vi "SOUR_POW_CORR_STAT.vi"(0 "VISA IN":refnum<visa-resource-name>, 5 "error in":errorcluster, 7 "Channel":i32) -> (14 "VISA Out":refnum<visa-resource-name>, 16 "Data":string, 19 "error out":errorcluster)   [LabVIEW 2018, in "PNA-X.lvlib"]
doc: "SOURce:POWer:CORRection[:STATe]? [src] \nReturn \nType \nBoolean (1 = ON, 0 = OFF) \nDefault OFF (0) \nLast modified: \nApril 17, 2007 Removed ch and port arguments for 4 settling and accuracy commands. \n9/12/06 MQ Modified for receiver only SPC \n1849\n\nStatus Register Commands \nThe status registers enable you to query the state of selected events that occur in the analyzer. \nNote: This documentation requires familiarity with the \"Standard Status Data Structure - Register \nModel\" as defined in IEEE Std 488.2-1992. \nClick on a blue keyword to view the command details. \nSee Also \nExample Programs \nLearn about Status Registers \nSynchronizing the PNA and Controller \nSCPI Command Tree \nNote: Any bit not shown in the registers is not used but may be reserved for future use. \n1850\n\nStatus Byte Register \nSummarizes the states of the other registers and monitors the PNA output queue. It also generates \nservice requests. The Enable register is called the Service Request Enable Register. \nCommands Description \n*CLS Clears ALL \"event\" registers and the SCPI Error / Event queue. The corresponding \nENABLE registers are unaffected. \n*STB? Reads the value of the analyzer's status byte. The byte remains after being read. \n*SRE? Reads the current state of the Service Request Enable Register. \n*SRE <num> Sets bits in the Service Request Enable register. The current setting of the SRE \nregister is stored in non-volatile memory. Use *SRE 0 to clear the enable. \n<num> Combined value of the weights for bits to be set. \nBit Weight Description Bit is set to 1 when the following conditions exist: \n2 4 Error / Event \nqueue Summary \n(EAV) \nthe Error / Event queue is not empty. To read the error \nmessage, use SYST:ERR? \n3 8 Questionable \nRegister Summary \nany enabled bit in the questionable event status register is \nset to 1 \n4 16 Message Available the output queue is not empty \n5 32 Standard Event \nRegister Summary \nany enabled bit in the standard event status register is set to \n1 \n6 64 Request Service any of the other bits in the status byte register is set to 1 \n(used to alert the controller of a service request within the \nanalyzer). This bit cannot be disabled. \n7 128 Operation Register \nSummary \nany enabled bit in the standard operation event status \nregister is set to 1 \n1851\n\nSTATus:QUEStionable:<keyword> \nSummarizes conditions that monitor the quality of measurement data. \n<keyword> Example \n:CONDition? STAT:QUES:COND? \n:ENABle \n<bits> \nSTAT:QUES:ENAB 1024 \n[:EVENt]? STAT:QUES? \n:NTRansition \n<bits> \nSTAT:QUES:NTR 1024 \n:PTRansition \n<bits> \nSTAT:QUES:PTR 0 \nBit Weight Description Bit is set to 1 when the following conditions exist: \n9 512 Integrity Reg \nsummary \nany enabled bit in the Integrity event register is set to 1 \n10 1024 Limit Registers \nsummary \nany enabled bit in the Limit event registers is set to 1 \n11 2048 Define Registers \nsummary \nany enabled bit in the Define event registers is set to 1 \nSTATus:QUEStionable:INTegrity <keyword> \nSummarizes conditions in the Measurement Integrity register. \n<keyword> Example \n:CONDition? STAT:QUES:INT:COND? \n:ENABle <bits> STAT:QUES:INT:ENAB 1024 \n[:EVENt]? STAT:QUES:INT? \n:NTRansition <bits> STAT:QUES:INT:NTR 1024 \n:PTRansition <bits> STAT:QUES:INT:PTR 0 \n1852\n\nBit Weight Description Bit is set to 1 when the following conditions exist: \n0 1 Measurement \nSummary \nany bit in the Measurement Integrity event register is set to \n1 \n2 4 Hardware \nSummary \nany bit in the Hardware event register is set to 1 \nSTATus:QUEStionable:INTegrity:HARDware<keyword> \nMonitors the status of hardware failures. \n<keyword> Example \n:CONDition? STAT:QUES:INT:HARD:COND? \n:ENABle <bits> STAT:QUES:INT:HARD:ENAB 1024 \n[:EVENt]? STAT:QUES:INT:HARD? \n:NTRansition <bits> STAT:QUES:INT:HARD:NTR 1024 \n:PTRansition <bits> STAT:QUES:INT:HARD:PTR 0 \nBit Weight Description Bit is set to 1 when the following conditions exist: \n1 2 Phase Unlock the source has lost phaselock, possibly caused by a reference \nchannel open or a hardware failure. \n2 4 Unleveled the source power is unleveled. This could be caused by a \nsource set for more power than it can deliver at the tuned \nfrequency. Or it could be caused by a hardware failure. \n3 8 Not used N/A \n4 16 EE Write Failed an attempted write to the EEPROM has failed, possibly \ncaused by a hardware failure. \n5 32 Not used N/A \n6 64 Ramp Cal Failed the analyzer was unable to calibrate the analog ramp \ngenerator due to a possible hardware failure. \n7 128 Not used N/A \n1853\n\nSTATus:QUEStionable:INTegrity:MEASurement<n> <keyword> \nMonitors the lag between changing a channel setting and when the data is ready to query. \nWhen you change the channel state (start/stop freq, bandwidth, and so forth), then the questionable bit \nfor that channel is set. This indicates that your desired channel state does not yet match the data you \nwould get if querying a data trace. When the next sweep is complete (without aborting in the middle), \nand the data trace matches the channel state that produced it, the bit is cleared for that channel. \n<n> Measurement register number. Choose from 1 to 3 \n<keyword> Example \n:CONDition? STAT:QUES:INT:MEAS1:COND? \n:ENABle <bits> STAT:QUES:INT:MEAS2:ENAB 1024 \n[:EVENt]? STAT:QUES:INT:MEAS3? \n:NTRansition <bits> STAT:QUES:INT:MEAS2:NTR 1024 \n:PTRansition <bits> STAT:QUES:INT:MEAS1:PTR 0 \nMeasurement Register <n> \nBit Weight 1 2 3 Bit is set to 1 when the following conditions exist: \n0 1 1 Summary \nfrom \nMeas \nReg 3 \na setting change on this channel has occurred and the \ndata does not yet reflect that change. \n1 2 2 15 29 a setting change on this channel has occurred and the \ndata does not yet reflect that change. \n2 4 3 16 30 a setting change on this channel has occurred and the \ndata does not yet reflect that change. \n3 8 4 17 31 a setting change on this channel has occurred and the \ndata does not yet reflect that change. \n4 16 5 18 32 a setting change on this channel has occurred and the \ndata does not yet reflect that change. \n5 32 6 19 a setting change on this channel has occurred and the \ndata does not yet reflect that change. \n6 64 7 20 a setting change on this channel has occurred and the \ndata does not yet reflect that change. \n1854\n\n7 128 8 21 a setting change on this channel has occurred and the \ndata does not yet reflect that change. \n8 256 9 22 a setting change on this channel has occurred and the \ndata does not yet reflect that change. \n9 512 10 23 a setting change on this channel has occurred and the \ndata does not yet reflect that change. \n10 1024 11 24 a setting change on this channel has occurred and the \ndata does not yet reflect that change. \n11 2048 12 25 a setting change on this channel has occurred and the \ndata does not yet reflect that change. \n12 4096 13 26 a setting change on this channel has occurred and the \ndata does not yet reflect that change. \n13 8192 14 27 a setting change on this channel has occurred and the \ndata does not yet reflect that change. \n14 16384 Summary \nfrom \nMeas \nReg 2 \n28 a setting change on this channel has occurred and the \ndata does not yet reflect that change. \nSTATus:QUEStionable:LIMit<n> <keyword> \nMonitors and summarizes the status of limit line failures. When a trace fails, the representative bit is \nset to 1. \nBit 0 is used to summarize failures in the registers that follow. For example, Limit Register 3, bit 0, \nsummarizes the failures from registers 4 through 10. \nAll enable bits are set to 1 by default. \nTo find the measurement number, use Calc:Par:Mnum \n<n> Limit register: Choose from 1 to 10. \n<keyword> Example \n:CONDition? STAT:QUES:LIM4:COND? \n:ENABle <bits> STAT:QUES:LIM1:ENAB 1024 \n[:EVENt]? STAT:QUES:LIM3? \n:NTRansition <bits> STAT:QUES:LIM2:NTR 1024 \n:NTRansition? STAT:QUES:LIM1:NTR? \n1855\n\n:PTRansition <bits> STAT:QUES:LIM5:PTR 0 \n:PTRansition? STAT:QUES:LIM1:PTR? \nLimit Register <n> \nBit Weight 1 2 3 4 5 6 7 8 ... 41 Bit is set to 1 when the \nfollowing conditions exist: \n0 1 2-42 3-42 4-42 5-42 6-42 7-42 8-42 9-42 ... 42 Summary Bit - If any bit \nfrom that register fails, it \npropagates to the previous \nregister, bit 0. \nTrace Numbers \n1 2 1 15 29 43 57 71 85 99 ... 575 any point on trace fails the \nlimit test \n2 4 2 16 30 44 58 72 86 100 ... 576 any point on trace fails the \nlimit test \n3 8 3 17 31 45 59 73 87 101 ... 577 any point on trace fails the \nlimit test \n4 16 4 18 32 46 60 74 88 102 ... 578 any point on trace fails the \nlimit test \n5 32 5 19 33 47 61 75 89 103 ... 579 any point on trace fails the \nlimit test \n6 64 6 20 34 48 62 76 90 104 ... 580 any point on trace fails the \nlimit test \n7 128 7 21 35 49 63 77 91 105 ... -- any point on trace fails the \nlimit test \n8 256 8 22 36 50 64 78 92 106 ... -- any point on trace fails the \nlimit test \n9 512 9 23 37 51 65 79 93 107 ... -- any point on trace fails the \nlimit test \n10 1024 10 24 38 52 66 80 94 108 ... -- any point on trace fails the \nlimit test \n11 2048 11 25 39 53 67 81 95 109 ... -- any point on trace fails the \nlimit test \n1856\n\n12 4096 12 26 40 54 68 82 96 110 ... -- any point on trace fails the \nlimit test \n13 8192 13 27 41 55 69 83 97 111 ... -- any point on trace fails the \nlimit test \n14 16384 14 28 42 56 70 84 98 112 ... -- any point on trace fails the \nlimit test \nTo determine Register, Bit number, and Weight for trace numbers between 113 and 574 (not shown in \nthe above table) use the following calculations. \nThe limit status for trace numbers higher than 580 can NOT be tracked. \nThe following example calculates the Register, Bit number, and Bit Weight for trace # 400: \nTo determine Limit Register number, use ((Trace # - 1) / 14) + 1. \nTo determine Limit Bit Number, use the remainder +1 of the above calculation. \n((400-1)/14) + 1 = Register# r+1Bit \n399/14 = 28 r7 \n28+1= Register 29 \n7+1= Bit number 8 \nTo determine Limit Bit Weight: Use above table. For example: Bit 8 = 256 \nSTATus:QUEStionable:DEFine<keyword> \nSummarizes conditions in the Questionable:Define:User<1|2|3> event registers. \n<keyword> Example \n:CONDition? STAT:QUES:DEF:COND? \n:ENABle <bits> STAT:QUES:DEF:ENAB 1024 \n[:EVENt]? STAT:QUES:DEF? \n:NTRansition <bits> STAT:QUES:DEF:NTR 1024 \n:PTRansition <bits> STAT:QUES:DEF:PTR 0 \n1857\n\nBit Weight Description Bit is set to 1 when the following conditions exist: \n1 2 USER1 any bit in the USER1 event register is set to 1 \n2 4 USER2 any bit in the USER2 event register is set to 1 \n3 8 USER3 any bit in the USER3 event register is set to 1 \nSTATus:QUEStionable:DEFine:USER<1|2|3><keyword> \nMonitors conditions that you define and map in any of the three QUES:DEF:USER event registers. \n<keyword> Example \n:ENABle <bits> STAT:QUES:DEF:USER1:ENABle 1024 \n[:EVENt]? STAT:QUES:DEF:USER1? \n:MAP <bit>,<error> STAT:QUES:DEF:USER1:MAP 0,-113 'when error -113 occurs, \nbit 0 in USER1 will set to 1. \nBit Weight Description Bit is set to 1 when the following conditions exist: \n0 1 for user user defined \n1 2 for user user defined \n2 4 for user user defined \n3 8 for user user defined \n4 16 for user user defined \n5 32 for user user defined \n6 64 for user user defined \n7 128 for user user defined \n8 256 for user user defined \n9 512 for user user defined \n10 1024 for user user defined \n11 2048 for user user defined \n12 4096 for user user defined \n13 8192 for user user defined \n14 16384 for user user defined \n1858\n\nStandard Event Status Register \nMonitors \"standard\" events that occur in the analyzer. This register can only be cleared by: \na Clear Command (*CLS). \nreading the Standard Enable Status Register (*ESE?). \na power-on transition. The analyzer clears the register and then records any transitions that occur, including \nsetting the Power On bit (7). \nCommands Description \n*ESE? Reads the settings of the standard event ENABLE register. \n*ESE <bits> Sets bits in the standard event ENABLE register. The current setting is saved in \nnon-volatile memory. \n<bits> The sum of weighted bits in the register. Use *ESE 0 to clear the enable \nregister. \n*ESR? Reads and clears the EVENT settings in the Standard Event Status register. \n*OPC Sets bit 0 when the overlapped command is complete. (see Understanding \nCommand Synchronization / OPC). \n*OPC? Operation complete query - read the Operation Complete bit (0). \nBit Weight Description Bit is set to 1 when the following conditions exist: \n0 1 Operation \nComplete \nthe two following events occur in order: \nthe *OPC command is sent to the analyzer 1. \nthe analyzer completes all pending overlapped commands 2. \n1 NA Request \nControl \nNot Supported - the analyzer application is not configured to \ncontrol GPIB operation \n2 4 Query Error a query error is detected indicating: \n- an attempt to read data from the output queue when no data was \npresent OR \n- data in the output queue was lost, as in an overflow \n4 16 Execution \nError \nan execution error is detected indicating: \n- a <PROGRAM DATA> element was outside the legal range or \ninconsistent with the operation of the analyzer OR \n1859\n\n- the analyzer could not execute a valid command due to some \ninternal condition \n5 32 Command \nError \na command error is detected indicating that the analyzer received \na command that: \ndid not follow proper syntax \nwas misspelled \nwas an optional command it does not implement \n7 128 Power ON Power to the analyzer has been turned OFF and then ON since the \nlast time this register was read. \nSTATus:OPERation<keyword> \nSummarizes conditions in the Averaging and Operation:Define:User<1|2|3> event registers. \n<keyword> Example \n:CONDition? STAT:OPER:COND? \n:ENABle <bits> STAT:OPER:ENAB 1024 \n[:EVENt]? STAT:OPER? \n:NTRansition <bits> STAT:OPER:NTR 1024 \n:PTRansition <bits> STAT:OPER:PTR 0 \nBit Weight Description Bit is set to 1 when the following conditions exist: \n8 256 Averaging \nsummary \neither enabled bit in the Averaging summary event register is set \nto 1 \n9 512 User Defined \nsummary \n10 1024 Device \nsummary \neither enabled bit in the Device summary event register is set to \n1 \n1860\n\nSTATus:OPERation:AVERaging<n> <keyword> \nMonitors and summarizes the status of Averaging on traces 1 to 128. When averaging for a trace is \ncomplete, the representative bit is set to 1. \nBit 0 is used to summarize the status in the registers that follow. For example, Average Register, bit 0, \nsummarizes the status from registers 4 through 10. \nAll enable bits are set to 1 by default. \nTo find the measurement number, use Calc:Par:Mnum. \n<n> Averaging Register. Choose from 1 to 10 \n<keyword> Example \n:CONDition? STAT:OPER:AVER1:COND? \n:ENABle <bits> STAT:OPER:AVER1:ENAB 1024 \n[:EVENt]? STAT:OPER:AVER1? \n:NTRansition <bits> STAT:OPER:AVER1:NTR 1024 \n:PTRansition <bits> STAT:OPER:AVER1:PTR 0 \nAveraging Register <n> \nBit Weight 1 2 3 4 5 6 7 8 ... 42 Bit is set to 1 when the \nfollowing conditions exist: \n0 1 2-42 3-42 4-42 5-42 6-42 7-42 8-42 9-42 ... 42 Summary Bit - If any bit \nfrom that register fails, it \npropagates to the previous \nregister, bit 0. \nTrace Numbers \n1 2 1 15 29 43 57 71 85 99 ... 575 Averaging on this trace is \ncomplete \n2 4 2 16 30 44 58 72 86 100 ... 576 Averaging on this trace is \ncomplete \n3 8 3 17 31 45 59 73 87 101 ... 577 Averaging on this trace is \ncomplete \n4 16 4 18 32 46 60 74 88 102 ... 578 Averaging on this trace is \ncomplete \n1861\n\n5 32 5 19 33 47 61 75 89 103 ... 579 Averaging on this trace is \ncomplete \n6 64 6 20 34 48 62 76 90 104 ... 580 Averaging on this trace is \ncomplete \n7 128 7 21 35 49 63 77 91 105 ... -- Averaging on this trace is \ncomplete \n8 256 8 22 36 50 64 78 92 106 ... -- Averaging on this trace is \ncomplete \n9 512 9 23 37 51 65 79 93 107 ... -- Averaging on this trace is \ncomplete \n10 1024 10 24 38 52 66 80 94 108 ... -- Averaging on this trace is \ncomplete \n11 2048 11 25 39 53 67 81 95 109 ... -- Averaging on this trace is \ncomplete \n12 4096 12 26 40 54 68 82 96 110 ... -- Averaging on this trace is \ncomplete \n13 8192 13 27 41 55 69 83 97 111 ... -- Averaging on this trace is \ncomplete \n14 16384 14 28 42 56 70 84 98 112 ... -- Averaging on this trace is \ncomplete \nTo determine Register, Bit number, and Weight for trace numbers between 113 and 574 (not shown in \nthe above table) use the following calculations. \nThe averaging status for trace numbers higher than 580 can NOT be tracked. \nThe following example calculates the Register, Bit number, and Bit Weight for trace # 400: \nTo determine Register number, use ((Trace # - 1) / 14) + 1. \nTo determine Bit Number, use the remainder +1 of the above calculation. \n((400-1)/14) + 1 = Register# r+1Bit \n399/14 = 28 r7 \n28+1= Register 29 \n7+1= Bit number 8 \n1862\n\nTo determine Bit Weight: Use above table. For example: Bit 8 = 256 \nSTATus:OPERation:DEFine<keyword> \nSummarizes conditions in the OPERation:Define:User<1|2|3> event registers. \n<keyword> Example \n:CONDition? STAT:OPER:DEF:COND? \n:ENABle <bits> STAT:OPER:DEF:ENAB 12 \n[:EVENt]? STAT:OPER:DEF? \n:NTRansition <bits> STAT:OPER:DEF:NTR 12 \n:PTRansition <bits> STAT:OPER:DEF:PTR 0 \nBit Weight Description Bit is set to 1 when the following conditions exist: \n1 2 USER1 any bit in the USER1 event register is set to 1 \n2 4 USER2 any bit in the USER2 event register is set to 1 \n3 8 USER3 any bit in the USER3 event register is set to 1 \nSTATus:OPERation:DEFine:USER<1|2|3><keyword> \nMonitors conditions that you define and map in any of the three OPER:DEF:USER event registers. \n<keyword> Example \n:ENABle <bits> STAT:OPER:DEF:USER1:ENAB 1024 \n[:EVENt]? STAT:OPER:DEF:USER1? \n:MAP <bit>,<error> STAT:OPER:DEF:USER1:MAP 0,-113 'when error -113 occurs, \nbit 0 in USER1 will set to 1. \n1863\n\nBit Weight Description Bit is set to 1 when the following conditions exist: \n0 1 for user user defined \n1 2 for user user defined \n2 4 for user user defined \n3 8 for user user defined \n4 16 for user user defined \n5 32 for user user defined \n6 64 for user user defined \n7 128 for user user defined \n8 256 for user user defined \n9 512 for user user defined \n10 1024 for user user defined \n11 2048 for user user defined \n12 4096 for user user defined \n13 8192 for user user defined \n14 16384 for user user defined \nSTATus:OPERation:DEVice<keyword> \nSummarizes conditions in the OPERation:DEVice event registers. \n<keyword> Example \n:CONDition? STAT:OPER:DEV:COND? \n:ENABle <bits> STAT:OPER:DEV:ENAB 16 \n[:EVENt]? STAT:OPER:DEV? \n:NTRansition <bits> STAT:OPER:DEV:NTR 16 \n:PTRansition <bits> STAT:OPER:DEV:PTR 0 \n1864\n\nBit Weight Description Bit is set to 1 when the following conditions exist: \n0 1 Unused \n1 2 Unused \n2 4 Unused \n3 8 Unused \n4 16 Sweep Completed When sweep is complete \n5 32 Unused \n6 64 Unused \n7 128 Unused \n8 256 Unused \n9 512 Unused \n10 1024 Unused \n11 2048 Unused \n12 4096 Unused \n13 8192 Unused \n14 16384 Unused \nLast modified: \nMay 31, 2007 Fixed typo in STAT:QUES:INT register \n9/19/06 MQ Modified for unlimited windows. \n1865\n\nSystem Commands \n1866\n\n1867\n\nClick on a blue keyword to view the command details. \nSee Also \nExample Programs \nLearn about Preset \nSynchronizing the PNA and Controller \nSCPI Command Tree \nSYSTem:ACTive:CHANnel? \n(Read-only) Returns the number of the active channel or an error message if there is no active \nchannel. The active channel is the channel number that contains the active measurement. \nExamples SYST:PRES \nSYST:ACT:CHAN? \n'Returns 1 \nReturn Type Integer \nDefault Not Applicable \nSYSTem:ACTive:MEASurement? \n(Read-only) Returns the name of the active measurement or an error message if there is no active \nmeasurement. While looking at the PNA display, the active measurement is the trace that has an \nindented Trace Status button and a label in the upper-left corner of the display. Only displayed \nmeasurements can be active. \nExamples SYST:PRES \nSYST:ACT:MEAS? \n'Returns \"CH1_S11_1\" \nReturn Type String \nDefault Not Applicable \nSYSTem:CHANnels:HOLD \n1868\n\n(Write-only) Places all channels in hold mode. To place a single channel in hold mode, use \nSENS:SWE:MODE. \nExamples SYST:CHAN:HOLD \nQuery Syntax Not Applicable \nDefault Not Applicable \nSYSTem:CHANnels:RESume \n(Write-only) Resumes the trigger mode of all channels that was in effect before sending \nSYSTem:CHANnels:HOLD (must be sent before SYST:CHAN:RESume). \nExamples SYST:CHAN:RES \nQuery Syntax Not Applicable \nDefault Not Applicable \nSYSTem:COMMunicate:GPIB:PMETer:ADDRess <num> \n(Read-Write) Specifies the GPIB address of the power meter to be used in a source power calibration. \nWhen performing a source power cal, the PNA will search VISA interfaces that are configured in the \nAgilent IO LIbraries on the PNA. \nParameters \n<num> GPIB address of the power meter. Choose any integer between 0 and 30. \nExamples SYST:COMM:GPIB:PMET:ADDR 13 \nsystem:communicate:gpib:pmeter:address 14 \nQuery Syntax SYSTem:COMMunicate:GPIB:PMETer:ADDRess? \nReturn Type Numeric \nDefault 13 \nSYSTem:COMMunicate:GPIB:RDEVice:CLOSe <ID> \n1869\n\n(Write only) Closes the remote GPIB session. This command should be sent when ending every \nsuccessful OPEN session. \nParameters \n<ID> Session identification number that was returned with the OPEN? command. \nExamples See an example program \nQuery Syntax Not Applicable \nDefault Not Applicable \nSYSTem:COMMunicate:GPIB:RDEVice:OPEN <bus>, <addr>, <timeout> \n(Read-Write) Initiates a GPIB pass-through session. First send this OPEN command, then send the \nOPEN query to read the session ID number. An existing GPIB pass-through session remains open \nafter an instrument preset. \nTo learn more about GPIB pass-through capability, see the example program. \nParameters \n<bus> Bus ID number. You can find the USB-GPIB adapter bus number by looking at \nthe dialog that appears when the USB-GPIB device is connected. Error 1073 \nindicates the bus or address number is incorrect. \n<addr> GPIB Address of the device to be controlled \n<timeout> The amount of time (in milliseconds) to wait for a response from the remote \ndevice after sending a command. A \"timeout\" error is displayed after this time \nhas passed without a response. \nExamples See an example program \nQuery Syntax SYSTem:COMMunicate:GPIB:RDEVice:OPEN? \nReturns the session identification number that is used when communicating \nwith this device. \nReturn Type Numeric \nDefault Not Applicable \nSYSTem:COMMunicate:GPIB:RDEVice:READ? <ID> \n1870\n\n(Read-only) Returns data from the GPIB pass-through device. \nParameters \n<ID> Session identification number that was returned with the OPEN? command. \nExamples See an example program \nReturn Type String \nDefault Not Applicable \nSYSTem:COMMunicate:GPIB:RDEVice:RESet \n(Write-only) Performs the same function as SYST:COMM:GPIB:RDEV:CLOS except that ALL \npass-through sessions are closed. \nExamples SYST:COMM:GPIB:RDEV:RES \nQuery Syntax Not Applicable \nDefault Not Applicable \nSYSTem:COMMunicate:GPIB:RDEVice:WBINary <ID>,<data> \n(Write-only) Sends data to a GPIB pass-through device. This command requires a header that \nspecifies the size of the data to be written. The header (described below) is not passed along to the \ndevice. \nUse this command if too many embedded quotes prevent you from using \nSYST:COMM:GPIB:RDEV:WRIT. \nUse SYST:COMM:GPIB:RDEV:OPEN to open the pass through session. \nParameters \n<ID> Session identification number that was returned with the OPEN? command. \n<data> Data to be sent to the GPIB pass-through device. Use the following syntax: \n#<num digits><byte count><data bytes><NL><END> \n<num_digits> specifies how many digits are contained in <byte_count> \n<byte_count> specifies how many data bytes will follow in <data bytes> \nExamples SYSTem:COMMunicate:GPIB:RDEVice:WBINary 101,#17ABC+XYZ<nl><end> \n# - always sent before data.\n1871\n\n1 - specifies that the byte count is one digit (7). \n7 - specifies the number of data bytes that will follow, not counting \n<NL><END>. \nABC+XYZ - Data block \n<nl><end> - always sent at the end of block data. \nThe following example sends a line feed at the end. \nSYST:COMM:GPIB:RDEV:WBIN 1,#210SYST:PRES<EOL> \nThe <EOL> represents your linefeed character. \nQuery Syntax Not Applicable \nDefault Not Applicable \nSYSTem:COMMunicate:GPIB:RDEVice:WBLock <ID>,<data> \n(Write-only) Same as SYSTem:COMM:GPIB:RDEV:WBIN (above) but the header IS passed along \nto the device. \nUse this command if too many embedded quotes prevent you from using \nSYST:COMM:GPIB:RDEV:WRIT. \nParameters \n<ID> Session identification number that was returned with the OPEN? command. \n<data> Data to be sent to the GPIB pass-through device. See previous command. \nExamples See previous example. \nQuery Syntax Not Applicable \nDefault Not Applicable \nSYSTem:COMMunicate:GPIB:RDEVice:WRITe <ID>,<string> \n1872\n\n(Write-only) Sends ASCII string data to the GPIB pass-through device. \nA line feed is NOT appended to the string data. To send a line feed, see the example in \nSYST:COMM:GPIB:RDEV:WBIN. \nParameters \n<ID> Session identification number that was returned with the OPEN? command. \n<string> Commands to be sent to the GPIB pass-through device. \nExamples See an example program \nQuery Syntax Not Applicable \nDefault Not Applicable \nSYSTem:CONFigure <model>,<address> \n(Write-only) Restarts as an \"N-port\" PNA using the specified multiport test set. \nLearn more about PNA Multiport capability. \nSee other commands to configure multiport test sets. \nParameters \n<model> String - Model of the test set with which to restart. \nUse \"Native\" to restart without a test set. \nTo see a list of supported test sets, use SENS:MULT:CAT? \n<address> Numeric - GPIB Address of the test set. Ignored when model = \"Native\". \nExamples SYST:CONF \"NATIVE\",0 \nsystem:configure \"N44xx\",18 \nQuery Syntax Not Applicable \nDefault Not Applicable \nSYSTem:CORRection:WIZard <char> \n1873\n\n(Write-only) Launches either the Calibration Wizard or the Version 2 Calibration Kit File Manager \ndialog box. \nParameters \n<char> Choose from: \nMAIN - Launches the Calibration Wizard \nCKIT - Launches the Version 2 Calibration Kit File Manager dialog box. \nBoth display on the PNA screen. \nExamples SYST:CORR:WIZ MAIN \nsystem:correction:wizard ckit \nQuery Syntax Not Applicable \nDefault Not Applicable \nSYSTem:ERRor? \n(Read-only) Returns the next error in the error queue. Each time the analyzer detects an error, it places \na message in the error queue. When the SYSTEM:ERROR? query is sent, one message is moved from \nthe error queue to the output queue so it can be read by the controller. Error messages are delivered to \nthe output queue in the order they were received. The error queue is cleared when any of the following \nconditions occur: \nWhen the analyzer is switched ON. \nWhen the *CLS command is sent to the analyzer. \nWhen all of the errors are read. \nIf the error queue overflows, the last error is replaced with a \"Queue Overflow\" error. The \noldest errors remain in the queue and the most recent error is discarded. \nExamples SYST:ERR? \nsystem:error? \nDefault Not Applicable \nSYSTem:ERRor:COUNt? \n1874\n\n(Read-only) Returns the number of errors in the error queue. Use SYST:ERR? to read an error. \nExamples SYST:ERR:COUN? \nsystem:error:count? \nDefault Not Applicable \nSYSTem:ERRor:REPort:SUNLeveled <bool> \n(Read-Write) Specifies whether or not to report Source Unleveled errors to the SCPI system error \nbuffer. \nParameters \n<bool> True (or 1) Report Source Unleveled Errors. Read errors from the system \nerror buffer using SYST:ERR? \nFalse (or 0) Do NOT report Source Unleveled Errors. \nExamples SYST:ERR:REP:SUNL 1 \nsystem:error:report:sunleveled true \nQuery Syntax SYSTem:ERRor:REPort:UNLeveled? \nDefault False \nSYSTem:FPReset \n(Write-only) Performs a standard Preset, then deletes the default trace, measurement, and window. \nThe PNA screen becomes blank. \nExamples SYST:FPR \nsystem:fpreset \nDefault Not applicable \nSYSTem:MACRo:COPY:CHANnel<cnum>[:TO] <num> \n1875\n\n(Write-only) Sets up channel <num> as a copy of channel <cnum>. Learn more about copy channels. \nParameters \n<cnum> Any existing channel number. If unspecified, value is set to 1. \n<num> Number of the channel which is to become a copy of channel <cnum>. \nExamples SYST:MACR:COPY:CHAN1 2 \nsystem:macro:copy:channel2:to 3 \nQuery Syntax Not Applicable \nDefault Not Applicable \nSYSTem:PRESet \n(Write-only) Deletes all traces, measurements, and windows. In addition, resets the analyzer to factory \ndefined default settings and creates a S11 measurement named \"CH1_S11_1\". For a list of default \nsettings, see Preset. \nRegardless of the state of the User Preset Enable checkbox, the SYST:PRESet command will always \npreset the PNA to the factory preset settings, and SYST:UPReset will always perform a User Preset. \nIf the PNA display is disabled with DISP:ENAB OFF then SYST:PRES will NOT enable the display. \nThis command performs the same function as *RST. \nExamples SYST:PRES \nsystem:preset \nDefault Not applicable \nSYSTem:PREFerences:ITEM:OFFSet:RCV <bool> \n1876\n\n(Read-Write) Set and return whether to offset the test port receivers by the amount of receiver \nattenuation. Learn more. \nTo send this command using the PNA front panel, open the GPIB Command Processor Console, then \ntype either of the following examples at the command prompt. Then type the Query Syntax and press \nenter to be sure the PNA took the command. \nThis setting remains until changed again using this command, or until the hard drive is changed or \nreformatted. \nParameters \n<bool> Choose from: \nTrue (1) Offset the test port receivers \nFalse (0) Do NOT offset the test port receivers \nExamples SYST:PREF:ITEM:OFFS:RCV 1 \nsystem:preferences:item:offset:rcv false \nQuery Syntax SYSTem:PREFerences:ITEM:OFFSet:RCV? \nReturn Type Boolean \nDefault PNA-L and E836xB: False (does NOT offset the display). \nPNA-X: True (offsets the display). \nSYSTem:PREFerences:ITEM:OFFSet:SRC <bool> \n(Read-Write) Set and return whether to offset the reference receiver by the amount of source \nattenuation. Learn more. \nTo send this command using the PNA front panel, open the GPIB Command Processor Console, then \ntype either of the following examples at the command prompt. Then type the Query Syntax and press \nenter to be sure the PNA took the command. \nThis setting remains until changed again using this command, or until the hard drive is changed or \nreformatted. \nParameters \n<bool> Choose from: \nTrue (1) Offset the reference receivers. \nFalse (0) Do NOT Offset the reference receivers. \n1877\n\nExamples SYST:PREF:ITEM:OFFS:SRC 1 \nsystem:preferences:item:offset:src false \nQuery Syntax SYSTem:PREFerences:ITEM:OFFSet:SRC? \nReturn Type Boolean \nDefault All models: True (offset the display). \nSYSTem:PREFerences:ITEM:PSRTrace <char> \n(Read-Write) At the end of a power sweep, while waiting to trigger the next sweep, maintain source \npower at either the start power level or at the stop power level. \nTo send this command using the PNA front panel, open the GPIB Command Processor Console, then \ntype either of the following examples at the command prompt. Then type the Query Syntax and press \nenter to be sure the PNA took the command. \nThis setting remains until changed again using this command, or until the hard drive is changed or \nreformatted. \nParameters \n<char> Choose from: \nSTARt - Maintain source power at the start power level. \nSTOP - Maintain source power at the stop power level. \nExamples SYST:PREF:ITEM:PSRT STOP \nsystem:preferences:item:psrtrace start \nQuery Syntax SYSTem:PREFerences:ITEM:PSRTrace? \nReturn Type Character \nDefault STARt \nSYSTem:PREFerences:ITEM:RETRace:POWer <char> \n1878\n\n(Read-Write) For single-band frequency or segment sweeps ONLY, specify whether to turn RF power \nON or OFF during a retrace. Learn more about RF power during sweep retrace. \nTo send this command using the PNA front panel, open the GPIB Command Processor Console, then \ntype either of the following examples at the command prompt. Then type the Query Syntax and press \nenter to be sure the PNA took the command. \nThis setting remains until changed using this command, or until the hard drive is changed or \nreformatted. \nParameters \n<char> Choose from: \nAUTO: Power is left ON during retrace of single-band frequency or segment \nsweeps ONLY. \nOFF: Power is turned OFF during retrace of single-band frequency or segment \nsweeps ONLY. \nExamples SYST:PREF:ITEM:RETR:POW OFF \nsystem:preferences:item:retrace:power auto \nQuery Syntax SYSTem:PREFerences:ITEM:RETRace:POWer? \nReturn Type Character \nDefault AUTO \nSYSTem:SECurity[:LEVel] <char> \n(Read-Write) Sets and returns the display of frequency information on the PNA screen and printouts. \nLearn more about security level. \nParameters \n<char> Choose from: \nNone - ALL frequency information is displayed \nLow - NO frequency information is displayed. Frequency information can be \nredisplayed using the Security Setting dialog box or this command.. \nHigh - NO frequency information is displayed. Frequency information can be \nredisplayed ONLY by performing a Preset or recalling an instrument state with \nNone or Low security settings, or using this command. \n1879\n\nExamples SYST:SEC LOW \nsystem:security:level high \nQuery Syntax SYSTem:SECurity[:LEVel]? \nReturn Type Character \nDefault None \nSYSTem:UPReset \n(Write-only) Performs a User Preset. There must be an active User Preset state file (see Load and \nSave) or an error will be returned. Learn more about User Preset. \nRegardless of the state of the User Preset Enable checkbox, the SYST:PRESet command will always \npreset the PNA to the factory preset settings, and SYST:UPReset will always perform a User Preset. \nExamples SYST:UPReset \nsystem:upreset \nQuery Syntax Not Applicable \nDefault Not Applicable \nSYSTem:UPReset:FPANel[:STATe] <bool> \n(Read-Write) 'Checks' and 'clears' the enable box on the User Preset dialog box. This only affects \nsubsequent Presets from the front panel user interface. \nRegardless of the state of the User Preset Enable checkbox, the SYST:PRESet command will always \npreset the PNA to the factory preset settings, and SYST:UPReset will always perform a User Preset. \nParameters \n<bool> Front Panel User Preset State. Choose from: \n0 User Preset OFF \n1 User Preset ON \nExamples SYST:UPR:FPAN 1 \nsystem:upreset:fpanel:state 0 \nQuery Syntax SYSTem:UPREset:FPANel[:STATe]? \nReturn Type Boolean \nDefault 0 \n1880\n\nSYSTem:UPReset:LOAD <file> \n(Read-Write) Loads an existing instrument state file (.sta or .cst) to be used for User Preset. \nSubsequent execution of SYSTem:UPReset will cause the PNA to assume this instrument state. \nRegardless of the state of the User Preset Enable checkbox, the SYST:PRESet command will always \npreset the PNA to the factory preset settings, and SYST:UPReset will always perform a User Preset. \nLearn more about User Preset. \nParameters \n<file> String - Name of the file to be loaded. The default folder \"C:\\Program \nFiles\\Agilent\\Network Analyzer\\Documents\" is used if unspecified. Change \nthe default folder name using MMEMory:CDIRectory. \nExamples SYST:UPR:LOAD '1MHzto20GHzUserPreset.cst' \nsystem:upreset:load 'C:\\Documents and Settings\\Administrator\\My \nDocuments\\NewUserPreset.cst' \nQuery Syntax Not Applicable \nDefault Not Applicable \nSYSTem:UPReset:SAVE[:STATe] \n(Write-only) Saves the current instrument settings as UserPreset.sta. Subsequent execution of \nSYSTem:UPReset will cause the PNA to assume this instrument state. \nRegardless of the state of the User Preset Enable checkbox, the SYST:PRESet command will always \npreset the PNA to the factory preset settings, and SYST:UPReset will always perform a User Preset. \nLearn more about User Preset. \nExamples SYST:UPR:SAVE \nsystem:upreset:save:state \nQuery Syntax Not Applicable \nDefault Not Applicable \nSYSTem:SHORtcut<n>:ARGuments<string> \n1881\n\n(Read-Write) Reads and writes the arguments for the specified macro. On the Edit Macro Dialog, this \nis called the \"Macro run string parameters\". \nParameters \n<n> Numeric. Number of the macro that is stored in the PNA. \nTo find the number of a macro, either open the Macro Setup dialog and count \nthe line number of the desired macro, or query the titles of all 12 macros for the \ndesired macro title. \n<string> Arguments for the specified macro. \nExamples SYST:SHOR1:ARG \n\"http://na.tm.agilent.com/pna/help/PNAWebHelp/help.htm\" \nQuery Syntax SYSTem:SHORtcut<n>:ARGuments? \nDefault Not Applicable \nSYSTem:SHORtcut<n>:DELete \n(Write-only) Removes the specified macro from the list of macros in the PNA. Does not delete the \nmacro executable file. \nParameters \n<n> Numeric. Number of the macro that is stored in the PNA. \nTo find the number of a macro, either open the Macro Setup dialog and count \nthe line number of the desired macro, or query the titles of all 12 macros for the \ndesired macro title. \nExamples SYST:SHOR1:DEL \nQuery Syntax Not Applicable \nDefault Not Applicable \nSYSTem:SHORtcut<n>:EXECute \n1882\n\n(Write-only) Executes (runs) the specified Macro (shortcut) that is stored in the PNA. \nParameters \n<n> Numeric. Number of the macro that is stored in the PNA. \nTo find the number of a macro, either open the Macro Setup dialog and count \nthe line number of the desired macro, or query the titles of all 12 macros for the \ndesired macro title. \nExamples SYST:SHOR1:EXEC \nQuery Syntax Not Applicable \nDefault Not Applicable \nSYSTem:SHORtcut<n>:PATH <string> \n(Read-Write) Defines a Macro (shortcut) by linking a path and file name to the Macro number. To be \nexecuted, the executable file must be put in the PNA at the location indicated by this command. \nParameters \n<n> Numeric. Number of the macro to be stored in the analyzer. If the index \nnumber already exists, the existing macro is replaced with the new macro. \n<string> Full path, file name, and extension, of the existing macro \"executable\" file. \nTo find the number of a macro, either open the Macro Setup dialog and count \nthe line number of the desired macro, or query the titles of all 12 macros for the \ndesired macro title. \nExamples SYST:SHOR1:PATH \"C:\\Program Files\\Agilent\\Network \nAnalyzer\\Documents\\unguideMultiple.vbs\" \nQuery Syntax SYSTem:SHORtcut<n>:PATH? \nDefault Not Applicable \nSYSTem:SHORtcut<n>:TITLe<string> \n1883\n\n(Read-Write) Reads and writes the name of the specified macro. \nParameters \n<n> Numeric. Number of the macro that is stored in the PNA. \nTo find the number of a macro, either open the Macro Setup dialog and count \nthe line number of the desired macro, or query the titles of all 12 macros for the \ndesired macro title. \n<string> The name to be assigned to the macro. \nExamples SYST:SHOR1:TITL \"Guided 4-Port Cal\" \nQuery Syntax SYSTem:SHORtcut<n>:TITLe? \nDefault Not Applicable \nSYSTem:TOUChscreen[:STATe] <bool> \n(Read-Write) Enables and disables the PNA-X touchscreen. \nThis setting remains until changed again from the front-panel or remotely, or until the hard drive is \nchanged or reformatted. \nParameters \n<bool> Choose from: \nTrue (1) Enables the touchscreen. \nFalse (0) Disables the touchscreen. \nExamples SYST:TOUC 1 \nsystem:touchscreen:state false \nQuery Syntax SYSTem:TOUChscreen[:STATe]? \nReturn Type Boolean \nDefault TRUE when shipped from factory. \nLast modified: \nFebruary 23, 2007 MX Added touchscreen command \nNov. 15, 2006 MX Added Unleveled Error reporting \nOct 31, 2006 Added PSRTrace command \n1884\n\n1885\n\nTrigger Commands \nControls the starts or ends of data acquisition. \nClick on a blue keyword to view the command details. \nSee Also \nExample program Triggering the PNA \nSee other SCPI Triggering commands \nLearn about External / Aux Triggering \nSynchronizing the PNA and Controller \n1886\n\nSCPI Command Tree \nTRIGger:AUX:COUNt? \n(Read-only) Returns the number of AUX trigger input / output connector pairs in the instrument. \nPNA-X = 2 \nE836xB and PNA-L models = 1 \nParameters \nExamples TRIG:CHAN:AUX:COUN? \ntrigger:channel2:aux:count? \nReturn Type Numeric \nDefault Not Applicable \nTRIGger:CHANnel<ch>:AUX<n>:DELay <num> \n(Read-Write) Specifies the delay that should be applied by the PNA after the Aux trigger input is \nreceived and before the acquisition is made. \nParameters \n<ch> Any existing channel number. If unspecified, value is set to 1. \n<n> Rear panel connectors used to send or receive signals. \nPNA-X - choose from 1 (AUX TRIG 1 IN) or 2 (AUX TRIG 2 IN) \nAll other models: choose 1. \nIf unspecified, value is set to 1. \n<num> Delay value in seconds. Choose a value between 0 and 3.0 seconds. \nExamples TRIG:CHAN:AUX:DEL .5 \ntrigger:channel2:aux2:delay 1.5 \nQuery Syntax TRIGger:CHANnel<ch>:AUX<n>:DELay? \nReturn Type Numeric \nDefault 0 \n1887\n\nTRIGger:CHANnel<ch>:AUX<n>:DURation <num> \n(Read-Write) Specifies the width of the output pulse, which is the time that the Aux trigger output \nwill be asserted. \nParameters \n<ch> Any existing channel number. If unspecified, value is set to 1. \n<n> Rear panel connector used to send or receive signals. \nPNA-X - choose from 1 (AUX TRIG 1) or 2 (AUX TRIG 2) \nAll other models: choose 1. (BNC Trig I/O \nIf unspecified, value is set to 1. \n<num> Duration value in seconds. Choose a value between 1us (1E-6) and 1 \nExamples TRIG:CHAN:AUX:DUR .1 \ntrigger:channel2:aux2:duration .01 \nQuery Syntax TRIGger:CHANnel<ch>:AUX<n>:DURation? \nReturn Type Numeric \nDefault 1E-6 \nTRIGger:CHANnel<ch>:AUX<n>[:ENABle] <bool> \n(Read-Write) Turns ON / OFF the trigger output. \nParameters \n<ch> Any existing channel number. If unspecified, value is set to 1. \n<n> Rear panel connector used to send or receive signals. \nPNA-X - choose from 1 (AUX TRIG 1) or 2 (AUX TRIG 2) \nAll other models: choose 1. (BNC Trig I/O \nIf unspecified, value is set to 1. \n<bool> ON (or 1) - turns trigger output ON. \nOFF (or 0) - turns trigger output OFF. \nExamples TRIG:CHAN:AUX 1 \ntrigger:channel2:aux2:enable off \n1888\n\nQuery Syntax TRIGger:CHANnel<ch>:AUX<n>:[ENABle]? \nReturn Type Boolean \nDefault OFF \nTRIGger:CHANnel<ch>:AUX<n>:HANDshake <bool> \n(Read-Write) Turns handshake ON / OFF. \nTo enable handshake, the main trigger enable must also be set using TRIG:CHAN:AUX:ENAB. \nWhen ON, PNA waits indefinitely for the input line to be asserted before continuing with the \nacquisition. When OFF, the PNA acquires data without waiting. \nParameters \n<ch> Any existing channel number. If unspecified, value is set to 1. \n<n> Rear panel connector used to send or receive signals. \nPNA-X - choose from 1 (AUX TRIG 1) or 2 (AUX TRIG 2) \nAll other models: choose 1. (BNC Trig I/O \nIf unspecified, value is set to 1. \n<bool> ON (or 1) - turns handshaking ON. \nOFF (or 0) - turns handshaking OFF. \nExamples TRIG:CHAN:AUX:HAND 1 \ntrigger:channel2:aux2:handshake off \nQuery Syntax TRIGger:CHANnel<ch>:AUX<n>:HANDshake? \nReturn Type Boolean \nDefault OFF \nTRIGger:CHANnel<ch>:AUX<n>:INTerval <char> \n1889\n\n(Read-Write) Specifies how often a trigger output signal is sent. \nParameters \n<ch> Any existing channel number. If unspecified, value is set to 1. \n<n> Rear panel connector used to send or receive signals. \nPNA-X - choose from 1 (AUX TRIG 1) or 2 (AUX TRIG 2) \nAll other models: choose 1. (BNC Trig I/O \nIf unspecified, value is set to 1. \n<char> Choose from: \nPOINt Trigger signal is sent every data point. (effectively the same as Point \nsweep) \nSWEep Trigger signal is sent once every sweep. \nExamples TRIG:CHAN:AUX:INT POI \ntrigger:channel2:aux2:interval sweep \nQuery Syntax TRIGger:CHANnel<ch>:AUX<n>:INTerval? \nReturn Type Character \nDefault SWEep \nTRIGger:CHANnel<ch>:AUX<n>:IPOLarity <char> \n(Read-Write) Specifies the polarity of the trigger IN signal to which the PNA will respond. \nParameters \n<ch> Any existing channel number. If unspecified, value is set to 1. \n<n> Rear panel connector used to send or receive signals. \nPNA-X - choose from 1 (AUX TRIG 1) or 2 (AUX TRIG 2) \nAll other models: choose 1. (BNC Trig I/O \nIf unspecified, value is set to 1. \n<char> Choose from: \nPOSitive PNA responds to leading edge or HIGH level \n1890\n\nNEGative PNA responds to trailing edge or LOW level. \nSet Edge or Level triggering using TRIG:CHAN:AUX:TYPE \nExamples TRIG:CHAN:AUX:IPOL POS \ntrigger:channel2:aux2:ipolarity negative \nQuery Syntax TRIGger:CHANnel<ch>:AUX<n>:IPOLarity? \nReturn Type Character \nDefault NEGative \nTRIGger:CHANnel<ch>:AUX<n>:OPOLarity <char> \n(Read-Write) Specifies the polarity of the Aux Output signal being supplied by the PNA. \nParameters \n<ch> Any existing channel number. If unspecified, value is set to 1. \n<n> Rear panel connector used to send or receive signals. \nPNA-X - choose from 1 (AUX TRIG 1) or 2 (AUX TRIG 2) \nAll other models: choose 1. (BNC Trig I/O \nIf unspecified, value is set to 1. \n<char> Choose from: \nPOSitive PNA sends positive going pulse. \nNEGative PNA sends negative going pulse. \nExamples TRIG:CHAN:AUX:OPOL NEG \ntrigger:channel2:aux2:opolarity positive \nQuery Syntax TRIGger:CHANnel<ch>:AUX<n>:OPOLarity? \nReturn Type Character \nDefault NEGative \nTRIGger:CHANnel<ch>:AUX<n>:POSition <char> \n1891\n\n(Read-Write) Specifies whether the aux trigger out signal is sent BEFore or AFTer the acquisition. \nParameters \n<ch> Any existing channel number. If unspecified, value is set to 1. \n<n> Rear panel connector used to send or receive signals. \nPNA-X - choose from 1 (AUX TRIG 1) or 2 (AUX TRIG 2) \nAll other models: choose 1. (BNC Trig I/O \nIf unspecified, value is set to 1. \n<char> Choose from: \nBEFore Use if the external device needs to be triggered before the data is \nacquired, such as a power meter. \nAFTer Use if the external device needs to be triggered just after data has been \nacquired, such as an external source. This could be more efficient since it allows \nthe external device to get ready for the next acquisition at the same time as the \nPNA. \nExamples TRIG:CHAN:AUX:POS BEF \ntrigger:channel2:aux2:position after \nQuery Syntax TRIGger:CHANnel<ch>:AUX<n>:POSition? \nReturn Type Character \nDefault AFTer \nTRIGger:CHANnel<ch>:AUX<n>:TYPE <char>\n1892\n\n(Read-Write) Specifies the type of Aux input detection that the PNA will employ. \nParameters \n<ch> Any existing channel number. If unspecified, value is set to 1. \n<n> Rear panel connector used to send or receive signals. \nPNA-X - choose from 1 (AUX TRIG 1) or 2 (AUX TRIG 2) \nAll other models: choose 1. (BNC Trig I/O \nIf unspecified, value is set to 1. \n<char> Choose from: \nEDGE PNA responds to the leading edge of a signal \nLEVel PNA responds to the level (HIGH or LOW) of a signal \nExamples TRIG:CHAN:AUX:TYPE EDGE \ntrigger:channel2:aux2:type level \nQuery Syntax TRIGger:CHANnel<ch>:AUX<n>:TYPE? \nReturn Type Character \nDefault EDGE \nTRIGger:DELay <num> \n(Read-Write) Sets and reads the trigger delay. This delay is only applied while in External Trigger \nmode. After an external trigger is applied, the start of the sweep is held off for an amount of time \nequal to the delay setting plus any inherent latency. \nParameters \n<num> Delay value in seconds. Choose from 0 to 107. \nExamples TRIG:DEL .0003 \nSets the trigger delay to 300 microseconds. The sweep will not \nstart until approximately 300 microseconds after an external \ntrigger is applied. \nQuery Syntax TRIGger:DELay? \nReturn Type Numeric \nDefault 0 \n1893\n\nTRIGger:CHANnel<ch>:ROUTe:INPut <char> \n(Read-Write) Specifies the connector to use for the external trigger input.(Similar to \nCONTROL:SIGNal <conn>) \nParameters \n<ch> Any existing channel number. If unspecified, value is set to 1. \n<char> Choose from: \nMAIN - meas trig ready \nMATH - material handler \nAUXT - auxio (PNA-L and E836xB ONLY) \nExamples TRIG:CHAN:ROUT:INP MAIN \ntrigger:channel2:route:input main \nQuery Syntax TRIGger:CHANnel<ch>:ROUTe:INPut? \nReturn Type Character \nDefault \nTRIGger:CHANnel<ch>:ROUTe:READy <char> \n(Read-Write) Specifies the connector to use for the external trigger OUT ready line. \nParameters \n<ch> Any existing channel number. If unspecified, value is set to 1. \n<char> Choose from: \nMAIN - Meas trig ready \nMATH - Material handler pin 21 \nAUXT - AUX I/O pin 18 (PNA-L and E836xB ONLY) \nExamples TRIG:CHAN:ROUT:READ main \ntrigger:channel2:route:ready auxt \nQuery Syntax TRIGger:CHANnel<ch>:ROUTe:READy? \nReturn Type Character \nDefault \n1894\n\nTRIGger:PREFerence:AIGLobal <bool> \n(Read-Write) Sets the External Trigger OUT behavior to either Global or Channel. Learn more. \nThis command will cause the PNA to Preset. \nThis setting remains until changed again using this command, or until the hard drive is changed or \nreformatted. \nTo send this command using the PNA front panel, open the GPIB Command Processor Console, then \ntype either of the following examples at the command prompt. Then type the Query Syntax and press \nenter to be sure the PNA took the command. \nParameters \n<bool> Choose from: \nON (or 1) - External I/O Trig properties apply to ALL channels (Global) \nOFF (or 0) - External I/O Trig properties apply to each channel independently. \nExamples TRIG:PREF:AIGL 1 \ntrigger:preference:aiglobal 0 \nQuery Syntax TRIGger:PREFerence:AIGLobal? \nReturn Type Boolean \nDefault 1 - E836xB and PNA-L models \n0 - PNA-X models \nTRIGger[:SEQuence]:LEVel <char> - Superseded \n1895\n\nThis command is replaced with CONTrol:SIGNal \n(Read-Write) Triggers either on a High or Low level trigger signal. This setting only has an effect \nwhen TRIG:SOURce EXTernal is selected. \nParameters \n<char> Choose from: \nHIGH - analyzer triggers on TTL High \nLOW - analyzer triggers on TTL Low \nExamples TRIG:LEV HIGH \ntrigger:sequence:level low \nQuery Syntax TRIGger[:SEQuence]:LEVel? \nReturn Type Character \nDefault LOW \nTRIGger[:SEQuence]:SCOPe <char> \n(Read-Write) Specifies whether a trigger signal is sent to all channels or only the current channel. \nSee Triggering the PNA using SCPI. \nParameters \n<char> Choose from: \nALL - trigger signal is sent to all channels. Also sets SENS:SWEep:TRIG:POINt \nOFF on ALL channels. \nCURRent - trigger signal is sent to only one channel at a time. With each trigger \nsignal, the channel is incremented to the next triggerable channel. \nExamples TRIG:SCOP ALL \ntrigger:sequence:scope current \nQuery Syntax TRIGger[:SEQuence]:SCOPe? \nReturn Type Character \nDefault ALL \nTRIGger[:SEQuence]:SOURce <char> \n1896\n\n(Read-Write) Sets the source of the sweep trigger signal. This command is a super-set of \nINITiate:CONTinuous, which can NOT set the source to External. To configure external triggering, \nsee CONTrol:SIGNal. \nSee Triggering the PNA using SCPI. \nParameters \n<char> Choose from: \nEXTernal - external (rear panel) source. \nIMMediate - internal source sends continuous trigger signals \nMANual - sends one trigger signal when manually triggered from the front panel or \nINIT:IMM is sent. \nExamples TRIG:SOUR EXT \ntrigger:sequence:source immediate \nQuery Syntax TRIGger[:SEQuence]:SOURce? \nReturn Type Character \nDefault IMMediate \nTRIGger:TYPE <char> \n(Read-Write) Specifies the type of EXTERNAL trigger input detection used to listen for signals on \nthe Ext I/O Trig and Meas Trig IN connectors. Edge triggers are most commonly used. \nParameters \n<ch> Any existing channel number. If unspecified, value is set to 1. \n<char> Choose from: \nEDGE PNA responds to the rising and falling edge of a signal \nLEVel PNA responds to a level (HIGH or LOW). \nExamples TRIG:TYPE EDGE \ntrigger:type level \nQuery Syntax TRIGger:TYPE? \nReturn Type Character \nDefault EDGE \n1897\n\nLast modified: \nApril 24, 2007 Clarified trigger source and scope \nFeb 15, 2007 MX Updated for AUX triggering \n1898\n\nCatalog Measurements using SCPI \nThis Visual Basic Program does the following: \nCatalogs the currently defined measurements, windows, and traces \nSelects a measurement for further definition \nAdds a Title to the window \nTo run this program, you need: \nAn established GPIB interface connection \nSee Other SCPI Example Programs \nDim Meas as String \nDim Win as String \nDim Trace as String \n'Read the current measurements in Channel 1 \nGPIB.Write \"CALCulate1:PARameter:CATalog?\" \nMeas = GPIB.Read \nMsgBox (\"Ch1 Measurments: \" & Meas) \n'Read the current windows \nGPIB.Write \"DISPlay:CATalog?\" \nWin = GPIB.Read \nMsgBox (\"Windows: \" & Win) \n'Read current traces in window 1 \nGPIB.Write \"DISPlay:WINDow1:CATalog?\" \nTrace = GPIB.Read \nMsgBox (\"Traces in Window1: \" & Win) \n1899\n\nCreate an FOM Measurement \nThis example program does the following: \ncreates several Frequency Offset measurements in separate windows \ngenerates markers \ncalculates statistics \nsets limit lines and queries results \nqueries a measurement to determine if we have a balanced parameter and what type it is. \nThe SCPI commands in this example are sent over a COM interface using the SCPIStringParser object. You do \nNOT need a GPIB connection to run this example. \nThis VBScript (*.vbs) program can be run as a macro in the PNA. To do this, copy the following code into a text \neditor file such as Notepad and save it on the PNA hard drive as Balanced.vbs. Learn how to setup and run the \nmacro. \nSee Other SCPI Example Programs \nDim app \nDim scpi \nDim Rcount \nDim Rname \n' Create / Get the PNA application. \nSet app = CreateObject(\"AgilentPNA835x.Application\") \nSet scpi = app.ScpiStringParser \n' A comment \nscpi.Execute(\"SYST:FPRESET\") \n'Create an Uncoupled S21 measurement on Chan 1 \n'Query available ranges \nRcount= scpi.Execute(\"SENS:FOM:COUN?\" \nMsgBox(Rcount) \nFor i=1 to Rcount \nRname(i)=sens:fom:rang:name? \nMsgBox(Rname(i)) \nNext \nSENS:FOM:RANG2:COUPLED OFF \n1900\n\nSENS:FOM:RANG2:FREQ:START 1Ghz \nSENS:FOM:RANG2:FREQ:STOP 2Ghz \nSENS:FOM:RANG3:COUPLED OFF \nSENS:FOM:RANG3:FREQ:START 2Ghz \nSENS:FOM:RANG3:FREQ:STOP 3Ghz \nQuestions \nIs cnum necessary on Sens FOM Count? or CAT? Name?\n1901\n\nCreate a Measurement using SCPI \nThis VBScript program creates a new S21 measurement and displays it on the PNA screen. \nThe SCPI commands in this example are sent over a COM interface using the SCPIStringParser object. You do \nNOT need a GPIB connection to run this example. \nThis VBScript (*.vbs) program can be run as a macro in the PNA. To do this, copy the following code into a text \neditor file such as Notepad and save it on the PNA hard drive as NewMeas.vbs. Learn how to setup and run the \nmacro. \nSee Other SCPI Example Programs \nDim app \nDim scpi \n' Create / Get the PNA application. \nSet app = CreateObject(\"AgilentPNA835x.Application\") \nSet scpi = app.ScpiStringParser \n' A comment \n'Preset the analyzer \nscpi.Execute (\"SYST:FPReset\") \n' Create and turn on window 1 \nscpi.Execute (\"DISPlay:WINDow1:STATE ON\") \n'Define a measurement name, parameter \nscpi.Execute (\"CALCulate:PARameter:DEFine 'MyMeas',S21\") \n'Associate (\"FEED\") the measurement name ('MyMeas') to WINDow (1), and give the new \nTRACe a number (1). \nscpi.Execute (\"DISPlay:WINDow1:TRACe1:FEED 'MyMeas'\") \n1902\n\nCreate a Balanced Measurement using SCPI \nThis example program does the following: \ncreates several Balanced measurements in separate windows \ngenerates markers \ncalculates statistics \nsets limit lines and queries results \nqueries a measurement to determine if we have a balanced parameter and what type it is. \nNote: By their nature, balanced measurements are extremely sensitive to phase differences between the two RF \npaths that make up the balanced port, especially at higher frequencies. A good calibration (not performed in this \nexample) is critical to achieving good balanced measurement results. \nThe SCPI commands in this example are sent over a COM interface using the SCPIStringParser object. You do \nNOT need a GPIB connection to run this example. \nThis VBScript (*.vbs) program can be run as a macro in the PNA. To do this, copy the following code into a text \neditor file such as Notepad and save it on the PNA hard drive as Balanced.vbs. Learn how to setup and run the \nmacro. \nSee Other SCPI Example Programs \nDim app \nDim scpi \n' Create / Get the PNA application. \nSet app = CreateObject(\"AgilentPNA835x.Application\") \nSet scpi = app.ScpiStringParser \n' A comment \nscpi.Execute(\"SYST:FPRESET\") \n' Put in \"Single\" trigger mode. \nscpi.Execute(\"SENS:SWE:GROups:COUNt 1\") \nscpi.Execute(\"SENS:SWE:MODE GROUPS\") \n' This example uses DUT topology Bal-Bal - \n' a DUT with a balanced input and balanced output. \n'\n' Port mapping for our DUT: \n' logical port 1 = physical ports 1 and 4 \n' logical port 2 = physical ports 2 and 3 \n' The default is: \n' logical port 1 = physical ports 1 and 2 \n' logical port 2 = physical ports 3 and 4 \n'\n' logical 1 logical 2 \n' ___________ \n' 1 ------| |------ 2 + \n' | DUT | \n' 4 ------|___________|------ 3 - \n1903\n\nscpi.Execute(\"CALC:FSIM:BAL:DEVice BBALanced\") \nscpi.Execute(\"CALC:FSIM:BAL:TOPology:BBAL:PPORts 1,4,2,3\") \n' Set up stimulus \nscpi.Execute(\"SENS:SWE:POINts 801\") \nscpi.Execute(\"SENS:FREQ:STARt 10e6\") \nscpi.Execute(\"SENS:FREQ:STOP 1e9\") \n' Turn on Four windows \nscpi.Execute(\"DISP:WIND1:STATe ON\") \nscpi.Execute(\"DISP:WIND2:STATe ON\") \nscpi.Execute(\"DISP:WIND3:STATe ON\") \nscpi.Execute(\"DISP:WIND4:STATe ON\") \n' Create a trace called \"sdd21\", and for that trace turn on the balanced \n' transformation and set the balanced transformation to BBAL SDD21. \nscpi.Execute(\"CALC:PAR:DEF \"\"sdd21\"\",S11\") \nscpi.Execute(\"CALC:PAR:SEL \"\"sdd21\"\"\") \nscpi.Execute(\"CALC:FSIM:BAL:PAR:STATe ON\") \nscpi.Execute(\"CALC:FSIM:BAL:PAR:BBAL:DEF SDD21\") \n' Feed the sdd21 trace to window 1, trace 1 \nscpi.Execute(\"DISP:WIND1:TRAC1:FEED \"\"sdd21\"\"\") \n' Similarly create 3 more balanced transmission/conversion parameters \n' Create Scd21 \nscpi.Execute(\"CALC:PAR:DEF \"\"scd21\"\",S11\") \nscpi.Execute(\"CALC:PAR:SEL \"\"scd21\"\"\") \nscpi.Execute(\"CALC:FSIM:BAL:PAR:STATe ON\") \nscpi.Execute(\"CALC:FSIM:BAL:PAR:BBAL:DEF SCD21\") \nscpi.Execute(\"DISP:WIND1:TRAC2:FEED \"\"scd21\"\"\") \n' Create Sdc21 \nscpi.Execute(\"CALC:PAR:DEF \"\"sdc21\"\",S11\") \nscpi.Execute(\"CALC:PAR:SEL \"\"sdc21\"\"\") \nscpi.Execute(\"CALC:FSIM:BAL:PAR:STATe ON\") \nscpi.Execute(\"CALC:FSIM:BAL:PAR:BBAL:DEF SDC21\") \nscpi.Execute(\"DISP:WIND1:TRAC3:FEED \"\"sdc21\"\"\") \n' Create Scc21 \nscpi.Execute(\"CALC:PAR:DEF \"\"scc21\"\",S11\") \nscpi.Execute(\"CALC:PAR:SEL \"\"scc21\"\"\") \nscpi.Execute(\"CALC:FSIM:BAL:PAR:STATe ON\") \nscpi.Execute(\"CALC:FSIM:BAL:PAR:BBAL:DEF SCC21\") \nscpi.Execute(\"DISP:WIND1:TRAC4:FEED \"\"scc21\"\"\") \n' Now create logical port 1 reflection parameters, and place them in window 2 \nscpi.Execute(\"CALC:PAR:DEF \"\"sdd11\"\",S11\") \nscpi.Execute(\"CALC:PAR:SEL \"\"sdd11\"\"\") \nscpi.Execute(\"CALC:FSIM:BAL:PAR:STATe ON\") \nscpi.Execute(\"CALC:FSIM:BAL:PAR:BBAL:DEF SDD11\") \n' Feed the sdd11 trace to window 2, trace 1 \nscpi.Execute(\"DISP:WIND2:TRAC1:FEED \"\"sdd11\"\"\") \n' Similarly create 3 more balanced reflection/conversion parameters \nscpi.Execute(\"CALC:PAR:DEF \"\"scd11\"\",S11\") \nscpi.Execute(\"CALC:PAR:SEL \"\"scd11\"\"\") \nscpi.Execute(\"CALC:FSIM:BAL:PAR:STATe ON\") \nscpi.Execute(\"CALC:FSIM:BAL:PAR:BBAL:DEF SCD11\") \nscpi.Execute(\"DISP:WIND2:TRAC2:FEED \"\"scd11\"\"\") \nscpi.Execute(\"CALC:PAR:DEF \"\"sdc11\"\",S11\") \n1904\n\nscpi.Execute(\"CALC:PAR:SEL \"\"sdc11\"\"\") \nscpi.Execute(\"CALC:FSIM:BAL:PAR:STATe ON\") \nscpi.Execute(\"CALC:FSIM:BAL:PAR:BBAL:DEF SDC11\") \nscpi.Execute(\"DISP:WIND2:TRAC3:FEED \"\"sdc11\"\"\") \nscpi.Execute(\"CALC:PAR:DEF \"\"scc11\"\",S11\") \nscpi.Execute(\"CALC:PAR:SEL \"\"scc11\"\"\") \nscpi.Execute(\"CALC:FSIM:BAL:PAR:STATe ON\") \nscpi.Execute(\"CALC:FSIM:BAL:PAR:BBAL:DEF SCC11\") \nscpi.Execute(\"DISP:WIND2:TRAC4:FEED \"\"scc11\"\"\") \n' Now create reverse transmission parameters, and place them in window 3 \nscpi.Execute(\"CALC:PAR:DEF \"\"sdd12\"\",S11\") \nscpi.Execute(\"CALC:PAR:SEL \"\"sdd12\"\"\") \nscpi.Execute(\"CALC:FSIM:BAL:PAR:STATe ON\") \nscpi.Execute(\"CALC:FSIM:BAL:PAR:BBAL:DEF SDD12\") \n' Feed the sdd11 trace to window 3, trace 1 \nscpi.Execute(\"DISP:WIND3:TRAC1:FEED \"\"sdd12\"\"\") \n' Similarly create 3 more balanced reverse transmission/conversion parameters \nscpi.Execute(\"CALC:PAR:DEF \"\"scd12\"\",S11\") \nscpi.Execute(\"CALC:PAR:SEL \"\"scd12\"\"\") \nscpi.Execute(\"CALC:FSIM:BAL:PAR:STATe ON\") \nscpi.Execute(\"CALC:FSIM:BAL:PAR:BBAL:DEF SCD12\") \nscpi.Execute(\"DISP:WIND3:TRAC2:FEED \"\"scd12\"\"\") \nscpi.Execute(\"CALC:PAR:DEF \"\"sdc12\"\",S11\") \nscpi.Execute(\"CALC:PAR:SEL \"\"sdc12\"\"\") \nscpi.Execute(\"CALC:FSIM:BAL:PAR:STATe ON\") \nscpi.Execute(\"CALC:FSIM:BAL:PAR:BBAL:DEF SDC12\") \nscpi.Execute(\"DISP:WIND3:TRAC3:FEED \"\"sdc12\"\"\") \nscpi.Execute(\"CALC:PAR:DEF \"\"scc12\"\",S11\") \nscpi.Execute(\"CALC:PAR:SEL \"\"scc12\"\"\") \nscpi.Execute(\"CALC:FSIM:BAL:PAR:STATe ON\") \nscpi.Execute(\"CALC:FSIM:BAL:PAR:BBAL:DEF SCC12\") \nscpi.Execute(\"DISP:WIND3:TRAC4:FEED \"\"scc12\"\"\") \n' Now create reverse reflection parameters, and place them in window 4 \nscpi.Execute(\"CALC:PAR:DEF \"\"sdd22\"\",S11\") \nscpi.Execute(\"CALC:PAR:SEL \"\"sdd22\"\"\") \nscpi.Execute(\"CALC:FSIM:BAL:PAR:STATe ON\") \nscpi.Execute(\"CALC:FSIM:BAL:PAR:BBAL:DEF SDD22\") \n' Feed the sdd11 trace to window 3, trace 1 \nscpi.Execute(\"DISP:WIND4:TRAC1:FEED \"\"sdd22\"\"\") \n' Similarly create 3 more balanced reverse reflection parameters \nscpi.Execute(\"CALC:PAR:DEF \"\"scd22\"\",S11\") \nscpi.Execute(\"CALC:PAR:SEL \"\"scd22\"\"\") \nscpi.Execute(\"CALC:FSIM:BAL:PAR:STATe ON\") \nscpi.Execute(\"CALC:FSIM:BAL:PAR:BBAL:DEF SCD22\") \nscpi.Execute(\"DISP:WIND4:TRAC2:FEED \"\"scd22\"\"\") \nscpi.Execute(\"CALC:PAR:DEF \"\"sdc22\"\",S11\") \nscpi.Execute(\"CALC:PAR:SEL \"\"sdc22\"\"\") \nscpi.Execute(\"CALC:FSIM:BAL:PAR:STATe ON\") \nscpi.Execute(\"CALC:FSIM:BAL:PAR:BBAL:DEF SDC22\") \nscpi.Execute(\"DISP:WIND4:TRAC3:FEED \"\"sdc22\"\"\") \nscpi.Execute(\"CALC:PAR:DEF \"\"scc22\"\",S11\") \nscpi.Execute(\"CALC:PAR:SEL \"\"scc22\"\"\") \n1905\n\nscpi.Execute(\"CALC:FSIM:BAL:PAR:STATe ON\") \nscpi.Execute(\"CALC:FSIM:BAL:PAR:BBAL:DEF SCC22\") \nscpi.Execute(\"DISP:WIND4:TRAC4:FEED \"\"scc22\"\"\") \n' Show statistics for forward differential transmission \nscpi.Execute(\"CALC:PAR:SEL \"\"sdd21\"\"\") \nscpi.Execute(\"CALC:FUNC:STATistics:STATe ON\") \n' Set up test range for markers. Set up range 1 to be between 100MHz and 900MHz \nscpi.Execute(\"CALC:FUNC:DOMain:USER:STARt 1,100e6\") \nscpi.Execute(\"CALC:FUNC:DOMain:USER:STOP 1,900e6\") \n' Set up a marker on Sdd21, find minimum differential transmission \n' Set this marker to use user-range 1 (previously defined) \nscpi.Execute(\"CALC:PAR:SEL \"\"sdd21\"\"\") \nscpi.Execute(\"CALC:MARK ON\") \nscpi.Execute(\"CALC:MARK:FUNC:DOM:USER:RANGE 1\") \nscpi.Execute(\"CALC:MARK:FUNC:EXEC MIN\") \n' Find Maximum common mode to differential mode conversion within user-range 1. \nscpi.Execute(\"CALC:PAR:SEL \"\"sdc21\"\"\") \nscpi.Execute(\"CALC:MARK ON\") \nscpi.Execute(\"CALC:MARK:FUNC:DOM:USER:RANGE 1\") \nscpi.Execute(\"CALC:MARK:FUNC:EXEC MAX\") \n' Set up limit lines \n' 'MIN' Limit on Sdd21 between 100MHz and 900MHz at -2dB \nscpi.Execute(\"CALC:PAR:SEL \"\"sdd21\"\"\") \nscpi.Execute(\"CALC:LIM:SEGM:TYPE LMIN\") \nscpi.Execute(\"CALC:LIM:SEGM:STIM:STARt 100e6\") \nscpi.Execute(\"CALC:LIM:SEGM:STIM:STOP 900e6\") \nscpi.Execute(\"CALC:LIM:SEGM:AMPL:STARt -2\") \nscpi.Execute(\"CALC:LIM:SEGM:AMPL:STOP -2\") \nscpi.Execute(\"CALC:LIM:DISP:STATe ON\") \nscpi.Execute(\"CALC:LIM:STATe ON\") \n' 'MAX' Limit on Sdc21 between 100MHz and 900MHz at -20dB \nscpi.Execute(\"CALC:PAR:SEL \"\"sdc21\"\"\") \nscpi.Execute(\"CALC:LIM:SEGM:TYPE LMAX\") \nscpi.Execute(\"CALC:LIM:SEGM:STIM:STARt 100e6\") \nscpi.Execute(\"CALC:LIM:SEGM:STIM:STOP 900e6\") \nscpi.Execute(\"CALC:LIM:SEGM:AMPL:STARt -20\") \nscpi.Execute(\"CALC:LIM:SEGM:AMPL:STOP -20\") \nscpi.Execute(\"CALC:LIM:DISP:STATe ON\") \nscpi.Execute(\"CALC:LIM:STATe ON\") \n' \"Single\" trigger to take data. \nscpi.Execute(\"SENS:SWE:MODE GROUPS\") \nresponse = scpi.Execute(\"*OPC?\") \n' Read the limit status byte to determine pass/fail. \n' If bit 1 is set (+2), then our first measurement failed (Sdd21). \n' If bit 3 is set (+8), then our third measurement failed (Sdc21). \n' Both measurements failing would return +10. \nresponse = scpi.Execute(\"STAT:QUES:LIM1:COND?\") \nIf response <> 0 Then \nWscript.Echo \"Failure of limit lines: \" & response \nEnd If \n' Here we demonstrate how to determine if we have \n1906\n\n' a balanced parameter and what type it is. \n' Read back one parameter to verify its type \nscpi.Execute(\"CALC:PAR:SEL \"\"sdd21\"\"\") \n' Is this a balanced parameter? \nisbal = scpi.Execute(\"CALC:FSIM:BAL:PAR?\") \n' Which topology/device is set? \ndevice = scpi.Execute(\"CALC:FSIM:BAL:DEV?\") \ndevice = Left( device, Len(device)-1 ) ' strip off newline \n' Which parameter are we measuring within that topology? \nbalparam = scpi.Execute(\"CALC:FSIM:BAL:PAR:\" & device & \":DEF?\") \nbalparam = Left( balparam, Len(balparam)-1 ) ' strip off newline \nIf isbal Then \nWScript.Echo \"Balanced Parameter: \" & balparam & \" in topology: \" & device & \".\" \nElse \nWScript.Echo \"Parameter not balanced.\" \nEnd If \n1907\n\nChannels, Windows, and Measurements using SCPI \nSOURce and most SENSe commands act on the channel that is specified in the command. Channel 1 is default if \nnot specified. \nMost DISPlay commands act on the window and trace specified in the command. Window1 and Trace1 are \ndefault if not specified. \nCALCulate commands act on the selected measurement in the specified channel. Select the measurement for \neach channel using CALCulate<channel number>:PARameter:SELect <meas name>. You can select one \nmeasurement in each channel. \nThe following Visual Basic program does the following: \nPresets the analyzer \nCreate 2 windows \nCreate 2 Measurements \nFeed the measurements to windows / traces \nChange frequency ranges for channels \nSelect both measurements \nTurn marker 1 ON for each measurement \nTo run this program, you need: \nAn established GPIB interface connection \nSee Other SCPI Example Programs \nGPIB.Write \"SYSTem:PRESet\" \n'Create Measurements \nGPIB.Write \"CALCulate1:PARameter:DEFine 'Meas1',S11\" \nGPIB.Write \"CALCulate2:PARameter:DEFine 'Meas2',S21\" \n' Turn on windows - creates if new \nGPIB.Write \"DISPlay:WINDow1:STATE ON\" \nGPIB.Write \"DISPlay:WINDow2:STATE ON\" \n'Associate (\"FEED\") the measurement name('Meas1') to WINDow(1), and give the new \nTRACe a number(1). \nGPIB.Write \"DISPlay:WINDow1:TRACe1:FEED 'Meas1'\" \nGPIB.Write \"DISPlay:WINDow2:TRACe2:FEED 'Meas2'\" \n'Change each channel's frequency range \nGPIB.Write \"SENSe1:FREQuency:SPAN 1e9\" \nGPIB.Write \"SENSe2:FREQuency:SPAN 2e9\" \n1908\n\n'Select both measurements \nGPIB.Write \"CALCulate1:PARameter:SELect 'Meas1'\" \nGPIB.Write \"CALCulate2:PARameter:SELect 'Meas2'\" \n'Turn marker 1 ON for each measurement \nGPIB.Write \"CALCulate1:MARKer:STATe ON\" \nGPIB.Write \"CALCulate2:MARKer:STATE ON\" \n1909\n\nSetup Sweep Parameters using SCPI \nThis Visual Basic program sets up sweep parameters on the Channel 1 measurement. \nTo run this program, you need: \nAn established GPIB interface connection \nSee Other SCPI Example Programs \nGPIB.Write \"SYSTem:PRESet\" \n'Select the measurement \nGPIB.Write \"CALCulate:PARameter:SELect 'CH1_S11_1'\" \n'Set sweep type to linear \nGPIB.Write \"SENSe1:SWEep:TYPE LIN\" \n'Set IF Bandwidth to 700 Hz \nGPIB.Write \"SENSe1:BANDwidth 700\" \n'Set Center and Span Freq's to 4 GHz \nGPIB.Write \"SENSe1:FREQuency:CENTer 4ghz\" \nGPIB.Write \"SENSe1:FREQuency:SPAN 4ghz\" \n'Set number of points to 801 \nGPIB.Write \"SENSe1:SWEep:POINts 801\" \n'Set sweep generation mode to Analog \nGPIB.Write \"SENSe1:SWEep:GENeration ANAL\" \n'Set sweep time to Automatic \nGPIB.Write \"SENSe1:SWEep:TIME:AUTO ON\" \n'Query the sweep time \nGPIB.Write \"SENSe1:SWEep:TIME? \nSweepTime = GPIB.Read \n1910\n\nSetup the Display using SCPI \nThis Visual Basic program: \nSets data formatting \nTurns ON the Trace, Title, and Frequency Annotation \nAutoscales the Trace \nQueries Per Division, Reference Level, and Reference Position \nTurn ON and set averaging \nTurn ON and set smoothing \nTo run this program, you need: \nAn established GPIB interface connection \nSee Other SCPI Example Programs \nGPIB.Write \"SYSTem:PRESet\" \n'Select the measurement \nGPIB.Write \"CALCulate:PARameter:SELect 'CH1_S11_1'\" \n'Set the Data Format to Log Mag \nGPIB.Write \":CALCulate1:FORMat MLOG\" \n'Turn ON the Trace, Title, and Frequency Annotation \nGPIB.Write \"Display:WINDow1:TRACe1:STATe ON\" \nGPIB.Write \"DISPlay:WINDow1:TITLe:STATe ON\" \nGPIB.Write \"DISPlay:ANNotation:FREQuency ON\" \n'Autoscale the Trace \nGPIB.Write \"Display:WINDow1:TRACe1:Y:Scale:AUTO\" \n'Query back the Per Division, Reference Level, and Reference Position \nGPIB.Write \"DISPlay:WINDow1:TRACe1:Y:SCALe:PDIVision?\" \nPdiv = GPIB.Read \nGPIB.Write \"DISPlay:WINDow1:TRACe1:Y:SCALe:RLEVel?\" \nRlev = GPIB.Read \nGPIB.Write \"DISPlay:WINDow1:TRACe1:Y:SCALe:RPOSition?\" \nPpos = GPIB.Read \n'Turn ON, and average five sweeps \nGPIB.Write \"SENSe1:AVERage:STATe ON\" \nGPIB.Write \"SENSe1:AVERage:Count 5\" \n'Turn ON, and set 20% smoothing aperture \nGPIB.Write \"CALCulate1:SMOothing:STATe ON\" \n1911\n\nGPIB.Write \"CALCulate1:SMOothing:APERture 20\" \n1912\n\nTriggering the PNA using SCPI \nTo understand how to trigger the PNA using SCPI, it is very important to understand the PNA trigger model. Here is \na very simple explanation. These three separate functions control PNA triggering: \nTrigger:Source - Where the trigger signals originate: \nInternal Continuous \nInternal Manual (Single) \nExternal - a trigger source that is connected to the PNA rear panel. \n1. \nTrigger:Scope - what gets triggered: \nGlobal - each signal triggers all channels in turn. \nChannel - each signal triggers ONE channel. \n2. \nChannel settings (Sense<ch>:Sweep:Mode) How many triggers will each channel accept before going into \nhold. \nHOLD - channel will not trigger \nCONTinuous - channel triggers indefinitely \nGROups - channel accepts the number of triggers specified with the last SENS:SWE:GRO:COUN \n<num>. \nPoint trigger SENS1:SWE:TRIG:POINt \n3. \nWhen controlling the PNA using SCPI, a SINGLE trigger is used to ensure that a complete sweep is taken. This \nexample demonstrates how to Single trigger the PNA using two methods. \nSimplest Triggering This method sets the Trigger Source to Internal Continuous - a stream of trigger \nsignals. Each channel is configured to ACCEPT only a single trigger signal, then HOLD. This method can \nalso be used when an External trigger source sends a continuous stream of trigger signals. \nAdvanced Triggering This method SENDS a single trigger from the Source, either Internal (using INIT:IMM) \nor External triggering. Each channel is configured to accept an unlimited number of triggers. This method is \nthe only way to perform point triggering. See INIT:IMM Advanced for details when requiring multiple channels \nto accept continuous and single triggers. \nThe SCPI commands in this example are sent over a COM interface using the SCPIStringParser object. You do \nNOT need a GPIB connection to run this example. \nThis VBScript (*.vbs) program can be run as a macro in the PNA. To do this, copy the following code into a text \neditor file such as Notepad and save it on the PNA hard drive as Trigger.vbs. Learn how to setup and run the \nmacro. \n1913\n\nMeasurement setup example: sets up S11 traces on two channels, 10 points, sweep time of 2 seconds, which \nallows us to verify that the trace is being triggered. \nDim app \nDim scpi \n' Create / Get the PNA application. \nSet app = CreateObject(\"AgilentPNA835x.Application\") \nSet scpi = app.ScpiStringParser \n'============================================ \n'Setup the PNA \n'Preset the analyzer \nscpi.Execute (\"SYST:FPReset\") \n' Create and turn on window/channel 1 \nscpi.Execute (\"DISPlay:WINDow1:STATE ON\") \n'Define a measurement name, parameter \nscpi.Execute (\"CALCulate1:PARameter:DEFine 'MyMeas1',S11\") \n'Associate (\"FEED\") the measurement name ('MyMeas') to WINDow (1) \nscpi.Execute (\"DISPlay:WINDow1:TRACe1:FEED 'MyMeas1'\") \n' Create and turn on window/channel 2 \nscpi.Execute (\"DISPlay:WINDow2:STATE ON\") \n'Define a measurement name, parameter \nscpi.Execute (\"CALCulate2:PARameter:DEFine 'MyMeas2',S11\") \n'Associate (\"FEED\") the measurement name ('MyMeas') to WINDow (2) \nscpi.Execute (\"DISPlay:WINDow2:TRACe2:FEED 'MyMeas2'\") \n'Set slow sweep so we can see \nscpi.Execute (\"SENS1:SWE:TIME 2\") \nscpi.Execute (\"SENS2:SWE:TIME 2\") \n'set few number of points \nscpi.Execute (\"SENS1:SWE:POIN 10\") \nscpi.Execute (\"SENS2:SWE:POIN 10\") \n'============================================ \n' Put both channels in Hold \nscpi.Execute (\"SENS1:SWE:MODE HOLD\") \nscpi.Execute (\"SENS2:SWE:MODE HOLD\") \n'================================ \n'Pick Single Send or Single Accept \nresp=Msgbox (\"Single Send? - Click No for Single Accept\", 4, \"PNA Trigger Demo\") \n1914\n\nIf resp=6 Then \nSingleSend() \nElse \nSingleAccept() \nEnd If \nSimple Triggering The following example sends a continuous stream of trigger signals and each PNA channels is \nset to ACCEPT only a signal trigger signal, then HOLD using the Groups:Count = 1 setting. \nThis example can be used to configure External triggering where the trigger source sends a continuous \nstream of trigger signals. Configure the type of trigger signal that the PNA responds to using the \nCONTrol:SIGNal command. The command in this example sets the PNA to respond to HIGH TTL signals at \nthe rear-panel BNC1 trigger IN connector. This command also automatically sets Trigger Source to External \nTrigger. \nThe TRIG SCOPE (Global or Channel) setting is NOT practical with a continuous stream of trigger signals. \nThe example program directly controls when each channel is triggered. \nAlso, Point triggering can NOT be used with a continuous stream of trigger signals because, with Group \nCount = 1, the channel will accept as many triggers as necessary to complete ONE full sweep. Therefore, \nALL data points in the channel will be continuously triggered. Use the single SEND example for point \ntriggering. \nSub SingleAccept() \n'PNA sends continuous trigger signals \nscpi.Execute (\"TRIG:SOUR IMMediate\") \n'Uncomment the following to set External triggering \n'scpi.Execute (\"CONT:SIGN BNC1,TILHIGH\") \n'IMPORTANT: First send the Count number =1, \n'This command does not make the channel sweep \nscpi.Execute (\"SENS1:SWE:GRO:COUN 1\") \nscpi.Execute (\"SENS2:SWE:GRO:COUN 1\") \nAcceptOne() \nEnd Sub \nSub AcceptOne() \n'The following command makes the channel immediately sweep \n'*OPC? allows the measurement to complete before the controller sends another \ncommand \nscpi.Execute (\"SENS1:SWE:MODE GROUPS;*OPC?\") \n1915\n\n' You could do something to ch2 here before sweeping it \nscpi.Execute (\"SENS2:SWE:MODE GROUPS;*OPC?\") \nresp=Msgbox (\"Another trigger?\", 1, \"PNA Trigger Demo\") \nIf resp=1 Then \nAcceptOne() \nEnd If \nEnd Sub \nAdvanced Trigger This example section performs Single Send triggering. Here, single triggering is accomplished \nby SENDING one trigger signal from the Trigger source and each channel is setup to accept unlimited trigger \nsignals. See the INIT:IMM command for more details. \nUsing this method, it is possible to change Trigger:Scope to Global or Channel. Set trigger scope to channel \nif there is some code to execute between channel measurements. Similarly, this method can be used to set \nPoint triggering. Use this method if there is some code to execute between data point measurements. \nIn addition, this method can also be used to perform External triggering if the external trigger source is \ncapable of SENDING single triggers. See the CONTrol:SIGNal command to set the type of signal to which \nthe PNA will respond. \nIf the external source can only send a continuous stream of trigger signals, then the Single Accept section \nmust be used. \nSub SingleSend() \n'Set Source Internal - Manual Triggering \nscpi.Execute (\"TRIG:SOUR MANual\") \n'If using an External trigger source that is capable of \n'sending SINGLE trigger signals, then uncomment the following. \n'This command automatically sets trigger source to External \n'scpi.Execute (\"CONT:SIGN BNC1,TILHIGH\") \n'Setup Trigger Scope \n'WHAT gets triggered \n'Pick one using comments \n'Set Channel triggering \n'scpi.Execute (\"TRIG:SCOPe CURRent\") \n'Set Global triggering (Default) \nscpi.Execute (\"TRIG:SCOPe ALL\") \n'Set Channel Settings \n1916\n\n'The channels respond to UNLIMITED trigger signals (Default) \nscpi.Execute (\"SENS1:SWE:MODE CONTinuous\") \nscpi.Execute (\"SENS2:SWE:MODE CONTinuous\") \n'To do Point trigger on one or more channels, uncomment the following \n'Point trigger automatically sets Trig:Scope to Current/Channel \n'scpi.Execute (\"SENS1:SWE:TRIG:POINt ON\") \n'scpi.Execute (\"SENS2:SWE:TRIG:POINt ON\") \nIntTrig() \nEnd Sub \nSub IntTrig() \n'If External triggering, replace this Sub with code \n'to single trigger the External Trig Source \nDim resp \n'*OPC? allows the measurement to complete before the controller sends another \ncommand \nscpi.Execute (\"INITiate:IMMediate;*OPC?\") \nresp=Msgbox (\"Another trigger?\", 1, \"PNA Trigger Demo\") \nIf resp=1 Then \nIntTrig() \nEnd If \nEnd Sub \nLast modified: \nApril 24, 2007 Updated with links \nOct. 5, 2006 New topic \n1917\n\nGPIB using Visual C++ \nSee Other SCPI Example Programs \n/* \n* This example assumes the user's PC has a National Instruments GPIB board. The \nexample is comprised of three basic parts: \n* \n* 1. Initialization \n* 2. Main Body \n* 3. Cleanup \n* \n* The Initialization portion consists of getting a handle to the PNA and then doing \na GPIB clear of the PNA. \n* \n* The Main Body consists of the PNA SCPI example. \n* \n* The last step, Cleanup, releases the PNA for front panel control. \n*/ \n#include <stdio.h> \n#include <stdlib.h> \n/* \n* Include the WINDOWS.H and DECL-32.H files. The standard Windows \n* header file, WINDOWS.H, contains definitions used by DECL-32.H and \n* DECL-32.H contains prototypes for the NI GPIB routines and constants. \n*/ \n#include <windows.h> \n#include \"decl-32.h\" \n#define ERRMSGSIZE 1024 // Maximum size of SCPI command string \n#define ARRAYSIZE 1024 // Size of read buffer \n#define BDINDEX 0 // Board Index of GPIB board \n#define PRIMARY_ADDR_OF_PNA 16 // GPIB address of PNA \n#define NO_SECONDARY_ADDR 0 // PNA has no Secondary address \n#define TIMEOUT T10s // Timeout value = 10 seconds \n#define EOTMODE 1 // Enable the END message \n#define EOSMODE 0 // Disable the EOS mode \nint pna; \nchar ValueStr[ARRAYSIZE + 1]; \nchar ErrorMnemonic[21][5] = {\"EDVR\", \"ECIC\", \"ENOL\", \"EADR\", \"EARG\", \n\"ESAC\", \"EABO\", \"ENEB\", \"EDMA\", \"\", \n\"EOIP\", \"ECAP\", \"EFSO\", \"\", \"EBUS\", \n\"ESTB\", \"ESRQ\", \"\", \"\", \"\", \"ETAB\"}; \nvoid GPIBWrite(char* SCPIcmd); \nchar *GPIBRead(void); \n1918\n\nvoid GPIBCleanup(int Dev, char* ErrorMsg); \nint main() \n{\nchar *opc; \nchar *result; \nchar *value; \n/* \n* ========================================= \n* INITIALIZATION SECTION \n* ========================================= \n*/ \n/* \n* The application brings the PNA online using ibdev. A device handle,pna, is \nreturned and is used in all subsequent calls to the PNA. \n*/ \npna = ibdev(BDINDEX, PRIMARY_ADDR_OF_PNA, NO_SECONDARY_ADDR, \nTIMEOUT, EOTMODE, EOSMODE); \nif (ibsta & ERR) \n{ \nprintf(\"Unable to open handle to PNA\\nibsta = 0x%x iberr = %d\\n\", \nibsta, iberr); \nreturn 1; \n} \n/* \n* Do a GPIB Clear of the PNA. If the error bit ERR is set in ibsta, call \nGPIBCleanup with an error message. \n*/ \nibclr (pna); \nif (ibsta & ERR) \n{ \nGPIBCleanup(pna, \"Unable to perform GPIB clear of the PNA\"); \nreturn 1; \n} \n/* \n* ========================================= \n* MAIN BODY SECTION \n* ========================================= \n*/ \n// Reset the analyzer to instrument preset \nGPIBWrite(\"SYSTem:FPRESET\"); \n// Create S11 measurement \nGPIBWrite(\"CALCulate1:PARameter:DEFine 'My_S11',S11\"); \n1919\n\n// Turn on Window #1 \nGPIBWrite(\"DISPlay:WINDow1:STATe ON\"); \n// Put a trace (Trace #1) into Window #1 and 'feed' it from the measurement \nGPIBWrite(\"DISPlay:WINDow1:TRACe1:FEED 'My_S11'\"); \n// Setup the channel for single sweep trigger \nGPIBWrite(\"INITiate1:CONTinuous OFF;*OPC?\"); \nopc = GPIBRead(); \nGPIBWrite(\"SENSe1:SWEep:TRIGger:POINt OFF\"); \n// Set channel parameters \nGPIBWrite(\"SENSe1:SWEep:POINts 11\"); \nGPIBWrite(\"SENSe1:FREQuency:STARt 1000000000\"); \nGPIBWrite(\"SENSe1:FREQuency:STOP 2000000000\"); \n// Send a trigger to initiate a single sweep \nGPIBWrite(\"INITiate1;*OPC?\"); \nopc = GPIBRead(); \n// Must select the measurement before we can read the data \nGPIBWrite(\"CALCulate1:PARameter:SELect 'My_S11'\"); \n// Read the measurement data into the \"result\" string variable \nGPIBWrite(\"FORMat ASCII\"); \nGPIBWrite(\"CALCulate1:DATA? FDATA\"); \nresult = GPIBRead(); \n// Print the data to the display console window \nprintf(\"S11(dB) - Visual C++ SCPI Example for PNA\\n\\n\"); \nvalue = strtok(result, \",\"); \nwhile (value != NULL) \n{ \nprintf(\"%s\\n\", value); \nvalue = strtok(NULL, \",\"); \n} \n/* \n* ========================================= \n* CLEANUP SECTION \n* ========================================= \n*/ \n/* The PNA is returned to front panel control. */ \nibonl(pna, 0); \nreturn 0; \n}\n/* \n* Write to the PNA \n*/ \n1920\n\nvoid GPIBWrite(char* SCPIcmd) \n{\nint length; \nchar ErrorMsg[ERRMSGSIZE + 1]; \nlength = strlen(SCPIcmd) ; \nibwrt (pna, SCPIcmd, length); \nif (ibsta & ERR) \n{ \nstrcpy(ErrorMsg, \"Unable to write this command to PNA:\\n\"); \nstrcat(ErrorMsg, SCPIcmd); \nGPIBCleanup(pna, ErrorMsg); \nexit(1); \n} \n}\n/* \n* Read from the PNA \n*/ \nchar* GPIBRead(void) \n{ \nibrd (pna, ValueStr, ARRAYSIZE); \nif (ibsta & ERR) \n{ \nGPIBCleanup(pna, \"Unable to read from the PNA\"); \nexit(1); \n} \nelse \nreturn ValueStr; \n}\n/* \n* After each GPIB call, the application checks whether the call succeeded. If an \nNI-488.2 call fails, the GPIB driver sets the corresponding bit in the global status \nvariable. If the call failed, this procedure prints an error message, takes the PNA \noffline and exits. \n*/ \nvoid GPIBCleanup(int Dev, char* ErrorMsg) \n{ \nprintf(\"Error : %s\\nibsta = 0x%x iberr = %d (%s)\\n\", \nErrorMsg, ibsta, iberr, ErrorMnemonic[iberr]); \nif (Dev != -1) \n{ \nprintf(\"Cleanup: Returning PNA to front panel control\\n\"); \nibonl (Dev, 0); \n} \n} \n1921\n\nPerform a Guided 2-Port or 4-Port Cal using SCPI \nThis example performs a Guided 2-Port or 4-port Calibration using ONE set of calibration standards or an ECAL \nmodule. \nA measurement must first be set up with desired frequency range, power, and so forth, ready to be calibrated. \nThe SCPI commands in this example are sent over a COM interface using the SCPIStringParser object. You do \nNOT need a GPIB connection to run this example. \nThis VBScript (*.vbs) program can be run as a macro in the PNA. To do this, copy the following code into a text \neditor file, such as Notepad, and save it on the PNA hard drive as *.vbs. \nLearn how to setup and run the macro. \nSee Guided Cal SCPI commands \nSee Other SCPI Example Programs \nDim app \nDim scpi \n' Create / Get the PNA application. \nSet app = CreateObject(\"AgilentPNA835x.Application\") \nSet scpi = app.ScpiStringParser \n' To perform 2-port cal, Uncomment TwoPortGuidedCal() \n' Then comment FourPortGuidedCal() \n'Do 2-port Cal \n'TwoPortGuidedCal() \n'Do 4-port Cal \nFourPortGuidedCal \nSub TwoPortGuidedCal() \n' Select the connectors \nscpi.Execute(\"sens:corr:coll:guid:conn:port1 \"\"APC 3.5 female\"\" \") \nscpi.Execute(\"sens:corr:coll:guid:conn:port2 \"\"APC 3.5 male\"\" \") \nscpi.Execute(\"sens:corr:coll:guid:conn:port3 \"\"Not used\"\" \") \nscpi.Execute(\"sens:corr:coll:guid:conn:port4 \"\"Not used\"\" \") \nMsgBox(\"Connectors defined for Ports 1 and 2\") \n' Select the Cal Kit for each port being calibrated. \nscpi.Execute(\"sens:corr:coll:guid:ckit:port1 \"\"85052D\"\" \") \nscpi.Execute(\"sens:corr:coll:guid:ckit:port2 \"\"85052D\"\" \") \n' To use an ECal module instead, comment out the above two lines \n' and uncomment these two lines and use the part number printed \n' on your module (which in our case was N4691-60004), followed \n' by the word 'ECal'. Your ECal module must already be connected \n' via USB to the PNA. \n'scpi.Execute(\"sens:corr:coll:guid:ckit:port1 \"\"N4691-60004 ECal\"\" \") \n'scpi.Execute(\"sens:corr:coll:guid:ckit:port2 \"\"N4691-60004 ECal\"\" \") \n1922\n\nMsgBox(\"Cal kits defined for Ports 1 and 2\") \n' Initiate the calibration and query the number of steps \nnumSteps = GenerateSteps() \n' Measure the standards, compute and apply the cal \nMeasureAndComplete(numSteps) \nEnd Sub \nSub FourPortGuidedCal() \n' Select the connectors \nscpi.Execute(\"sens:corr:coll:guid:conn:port1 \"\"APC 3.5 female\"\" \") \nscpi.Execute(\"sens:corr:coll:guid:conn:port2 \"\"APC 3.5 female\"\" \") \nscpi.Execute(\"sens:corr:coll:guid:conn:port3 \"\"APC 3.5 female\"\" \") \nscpi.Execute(\"sens:corr:coll:guid:conn:port4 \"\"APC 3.5 female\"\" \") \nMsgBox(\"Connectors defined for Ports 1 to 4\") \n' Select the Cal Kit for each port being calibrated. \nscpi.Execute(\"sens:corr:coll:guid:ckit:port1 \"\"85052D\"\" \") \nscpi.Execute(\"sens:corr:coll:guid:ckit:port2 \"\"85052D\"\" \") \nscpi.Execute(\"sens:corr:coll:guid:ckit:port3 \"\"85052D\"\" \") \nscpi.Execute(\"sens:corr:coll:guid:ckit:port4 \"\"85052D\"\" \") \n' To use an ECal module instead, comment out the above four lines \n' and uncomment these four lines and use the part number printed \n' on your module (which in our case was N4431-60003), followed \n' by the word 'ECal'. Your ECal module must already be connected \n' via USB to the PNA. \n'scpi.Execute(\"sens:corr:coll:guid:ckit:port1 \"\"N4431-60003 ECal\"\" \") \n'scpi.Execute(\"sens:corr:coll:guid:ckit:port2 \"\"N4431-60003 ECal\"\" \") \n'scpi.Execute(\"sens:corr:coll:guid:ckit:port3 \"\"N4431-60003 ECal\"\" \") \n'scpi.Execute(\"sens:corr:coll:guid:ckit:port4 \"\"N4431-60003 ECal\"\" \") \nMsgBox(\"Cal kits defined for Ports 1 to 4\") \n' Initiate the calibration and query the number of steps \nnumSteps = GenerateSteps() \n' If your selected cal kit is not a 4-port ECal module which can \n' mate to all 4 ports at once, then you may want to choose which \n' thru connections to measure for the cal. You must measure at \n' least 3 different thru paths for a 4-port cal (for greatest \n' accuracy you can choose to measure a thru connection for all 6 \n' pairings of the 4 ports). If you omit this command, the default \n' is to measure from port 1 to port 2, port 1 to port 3, and \n' port 1 to port 4. For this example we select to measure \n' from port 1 to port 2, port 2 to port 3, and port 2 to port 4. \nscpi.Execute(\"sens:corr:coll:guid:thru:ports 1,2,2,3,2,4\") \n' Re-generate the connection steps to account for the thru changes \nnumSteps = GenerateSteps() \n' Measure the standards, compute and apply the cal \nMeasureAndComplete(numSteps) \nEnd Sub \nFunction GenerateSteps() \n' Initiate the calibration and query the number of steps \nscpi.Execute(\"sens:corr:coll:guid:init\") \nGenerateSteps = scpi.Execute(\"sens:corr:coll:guid:steps?\") \nEnd Function \n1923\n\nSub MeasureAndComplete(numSteps) \nMsgBox(\"Number of steps is \" + CStr(numSteps)) \n' Measure the standards \nFor i = 1 To numSteps \nstep = \"Step \" + CStr(i) + \" of \" + CStr(numSteps) \nstrPrompt = scpi.Execute(\"sens:corr:coll:guid:desc? \" + CStr(i)) \nMsgBox strPrompt, vbOKOnly, step \nscpi.Execute(\"sens:corr:coll:guid:acq STAN\" + CStr(i)) \nNext \n' Conclude the calibration \nscpi.Execute(\"sens:corr:coll:guid:save\") \nMsgBox (\"Cal is done!\") \nEnd Sub \n1924\n\nPerform a Guided Calibration using SCPI \nThis VBScript program performs a Guided Calibration using ECal or Mechanical standards. This example includes \noptional ECal orientation features. \nThis example has been updated to include the setting of Unknown Thru or Adapter Removal adapter delay. \n(March 2006). \nThis example has been updated to show the activation of a channel to be calibrated. (Aug. 2006). \nThe SCPI commands in this example are sent over a COM interface using the SCPIStringParser object. You do \nNOT need a GPIB connection to run this example. \nThis VBScript (*.vbs) program can be run as a macro in the PNA. To do this, copy the following code into a text \neditor file such as Notepad and save it on the PNA hard drive as Guided.vbs. Learn how to setup and run the \nmacro. \n' Performing a Guided 2-port cal (Ports 1 and 2) \nTwoPortGuidedCal \nSub TwoPortGuidedCal \nDim app \nDim scpi \nDim connList \nDim selectedConn1, selectedConn2 \nDim kitList \nDim selectedKit \nDim message \n' Create / Get the PNA application. \nSet app = CreateObject(\"AgilentPNA835x.Application\") \nSet scpi = app.ScpiStringParser \n'The following demonstrates that the Active Channel is cal'd \n'Preset the PNA \nscpi.Execute \"SYST:PRES\" \n'Create a new measurement on Chan 2 \n'Now there are two windows, channels and measurements \n'This becomes the Active Measurement \nscpi.Execute (\"DISPlay:WINDow2:STATE ON\") \n'Define a measurement name, parameter \nscpi.Execute (\"CALCulate2:PARameter:DEFine 'MyMeas',S21\") \n'\"FEED\" the measurement \nscpi.Execute (\"DISPlay:WINDow2:TRACe1:FEED 'MyMeas'\") \n1925\n\n'This is the Active Measurement \n'Activate the 'Preset' measurement to cal chan 1 \nscpi.Execute (\"CALC1:PAR:SEL 'CH1_S11_1'\") \n' Query the list of connectors that the PNA system recognizes \nconnList = scpi.Execute(\"sens:corr:coll:guid:conn:cat?\") \n' Format the list with linefeed characters in place of the commas \nconnList = FormatList(connList) \nmessage = \"Enter your DUT connector for Port 1. Choose from this list:\" \nmessage = message & Chr(10) & Chr(10) & connList \n' Select the connector for Port 1 \nselectedConn1 = InputBox(message) \nIf selectedConn1 = \"\" Then Exit Sub \nscpi.Execute \"sens:corr:coll:guid:conn:port1 '\" & selectedConn1 & \"'\" \nmessage = \"Enter your DUT connector for Port 2. Again, choose from this list:\" \nmessage = message & Chr(10) & Chr(10) & connList \n' Select the connector for Port 2 \nselectedConn2 = InputBox(message) \nIf selectedConn2 = \"\" Then Exit Sub \nscpi.Execute \"sens:corr:coll:guid:conn:port2 '\" & selectedConn2 & \"'\" \n' Note: If your PNA has more than 2 ports, then uncomment \n' one or both of these next two lines. \n'scpi.Execute \"sens:corr:coll:guid:conn:port3 \"\"Not used\"\" \" \n'scpi.Execute \"sens:corr:coll:guid:conn:port4 \"\"Not used\"\" \" \n' This next block of commented code demonstrates how to specify an adapter \n' and it's electrical delay, in situations where you are performing an \n' Unknown Thru or Adapter Removal calibration. In most situations, the \n' PNA is able to correctly determine an adapter's electrical length \n' at the end of the calibration. However, there are scenarios where \n' the PNA cannot correctly calculate the length -- such as when the channel \n' has a relatively small number of measurement points (for example, 201 or less) \n' and the adapter is significantly long (for example, a cable that is several feet). \n' In these cases, the ADAP commands (below) enable you to explicitly specify \n' the adapter you are using. \n' Send these commands prior to the \"sens:corr:coll:guid:init\" command. \n1926\n\n' Create adapter and return the adapter number \n'adapterNum = scpi.Execute(\"sens:corr:coll:guid:adap:cre? '\" & selectedConn1 & \"','\"& selectedConn2 & \"'\") \n' The adapterNum string contains a '+' character. \n' Here we convert to integer to remove that. \n'adapterNum = CStr( CInt(adapterNum) ) \n' Specify that this adapter has 10 nanoseconds electrical delay (coaxial). \n'scpi.Execute \"sens:corr:coll:guid:adap\" & adapterNum & \":del 10E-9\" \n' Text description of adapter \n'scpi.Execute \"sens:corr:coll:guid:adap\" & adapterNum & \":desc 'My adapter'\" \n' Select to use this adapter specifically between ports 1 and 2 \n'scpi.Execute \"sens:corr:coll:guid:adap\" & adapterNum & \":path 1,2\" \n' End of adapter block \n' Query the list of acceptable cal kits and \n' ECal module characterizations for Port 1. \nkitList = scpi.Execute(\"sens:corr:coll:guid:ckit:port1:cat?\") \n' Format the list with linefeed \n' characters in place of the commas \nkitList = FormatList(kitList) \nmessage = \"Enter your cal kit or ECal module characterization for Port 1. \" \nmessage = message & \"Choose from this list:\" \nmessage = message & Chr(10) & Chr(10) & kitList \n' Select the Cal Kit or ECal module \n' characterization to use for Port 1. \nselectedKit = InputBox(message) \nIf selectedKit = \"\" Then Exit Sub \nscpi.Execute \"sens:corr:coll:guid:ckit:port1 '\" & selectedKit & \"'\" \n' Query the list of acceptable cal kits \n' and ECal module characterizations for Port 2. \nkitList = scpi.Execute(\"sens:corr:coll:guid:ckit:port2:cat?\") \n' Format the list with linefeed characters in place of the commas \nkitList = FormatList(kitList) \nmessage = \"Enter your cal kit or ECal module characterization for Port 2. \" \nmessage = message & \"Choose from this list:\" \nmessage = message & Chr(10) & Chr(10) & kitList \n' Select the Cal Kit or ECal module \n1927\n\n' characterization to use for Port 2. \nselectedKit = InputBox(message) \nIf selectedKit = \"\" Then Exit Sub \nscpi.Execute \"sens:corr:coll:guid:ckit:port2 '\" & selectedKit & \"'\" \n' This next block of commented code \n' shows optional functions when using ECal. \n' Send these \"sens:corr:pref\" commands prior to the \n' \"sens:corr:coll:guid:init\" command. \n' Read ECAL information from ECal module #1 on the USB bus \n' about the Agilent factory characterization data \n'module1Info = scpi.Execute(\"sens:corr:coll:ckit:inf? ECAL1,CHAR0\") \n'MsgBox \"Description of ECal Module #1:\" & Chr(10) & Chr(10) & module1Info \n' The following command enables auto orientation of \n' the ECal module (The PNA senses which port of the \n' module is connected to which port of the PNA). \n'scpi.Execute \"sens:corr:pref:ecal:ori ON\" \n' However, if you are measuring at very low power levels where \n' the PNA may fail to sense the module's orientation, then turn auto \n' orientation OFF and specify how the module is connected. \n' \"A1,B2\" indicates Port A of the module is connected \n' to PNA Port 1 and Port B is connected to PNA Port 2). \n'scpi.Execute \"sens:corr:pref:ecal:ori OFF\" \n'scpi.Execute \"sens:corr:pref:ecal:pmap ECAL1,'A1,B2'\" \n' End of optional ECal setup \n' Select the thru method of \"Default\". This instructs the PNA to \n' determine which thru standard measurement technique to use \n' based upon the selected connectors and \n' calibration kit(s) and the PNA model number. \n' with new CMET and TMET 'default' is set by not sending the commands \n'\n' Initiate the calibration and query the number of steps \nscpi.Execute \"sens:corr:coll:guid:init\" \nnumSteps = scpi.Execute(\"sens:corr:coll:guid:steps?\") \n1928\n\nMsgBox \"Number of steps is \" + CStr(numSteps) \n' Measure the standards \nFor i = 1 To numSteps \nstep = \"Step \" + CStr(i) + \" of \" + CStr(numSteps) \nstrPrompt = scpi.Execute(\"sens:corr:coll:guid:desc? \" + CStr(i)) \nMsgBox strPrompt, vbOKOnly, step \nscpi.Execute \"sens:corr:coll:guid:acq STAN\" + CStr(i) \nNext \n' Conclude the calibration \nscpi.Execute \"sens:corr:coll:guid:save\" \nMsgBox \"Cal is done!\" \nEnd Sub \nFunction FormatList(list) \nDim tokens \n' Strip the leading and trailing quotation \n' marks from the list string \nlist = Mid(list, 2, Len(list) - 3) \n' Tokenize the comma-delimited list string \n' into an array of the individual substrings \ntokens = Split(list, \",\") \n' Rebuild the list string, placing linefeed \n' characters where the commas were, \n' using Trim to remove leading and trailing spaces. \nlist = \"\" \nFor i = 0 To UBound(tokens) \ntokens(i) = Trim(tokens(i)) \nlist = list & tokens(i) & Chr(9) \nIf i < UBound(tokens) Then \ni = i + 1 \ntokens(i) = Trim(tokens(i)) \nlist = list & tokens(i) & Chr(10) \nEnd If \nNext \nFormatList = list \nEnd Function \n1929\n\nLast Modified: \n14-May-2007 MX Updated for new CMET and TMET commands \n1930\n\nPerform Guided ECal using SCPI \nThis VBScript program performs a Guided ECal Calibration. While this example is good to use as a starting point \nfor Guided ECal, the Guided comprehensive cal example has some advanced features that are not in this program. \nThe SCPI commands in this example are sent over a COM interface using the SCPIStringParser object. You do \nNOT need a GPIB connection to run this example. \nThis VBScript (*.vbs) program can be run as a macro in the PNA. To do this, copy the following code into a text \neditor file such as Notepad and save it on the PNA hard drive as Guided.vbs. Learn how to setup and run the \nmacro. \n' Performing a 2-port cal (Ports 1 and 2) \nDim app \nDim scpi \n' Create / Get the PNA application. \nSet app = CreateObject(\"AgilentPNA835x.Application\") \nSet scpi = app.ScpiStringParser \n' Specify the DUT connectors \n' (for each connector of your DUT, one of the ECal module's ports must have \n' that same connector, or else you cannot achieve the cal using that module). \nscpi.Execute \"sens:corr:coll:guid:conn:port1 \"\"APC 3.5 female\"\" \" \nscpi.Execute \"sens:corr:coll:guid:conn:port2 \"\"APC 3.5 male\"\" \" \n' Note: If your PNA has more than 2 ports, you would need to uncomment \n' one or both of these next two lines, to explicitly specify this is \n' just a 2-port cal. \n'scpi.Execute \"sens:corr:coll:guid:conn:port3 \"\"Not used\"\" \" \n'scpi.Execute \"sens:corr:coll:guid:conn:port4 \"\"Not used\"\" \" \nMsgBox \"Connectors defined for Ports 1 and 2\" \n' Select the ECal module for each port being calibrated. \n' Replace N4691-60004 with the part number printed on your module \n' followed by User x if using a User characterization, then the word 'ECal' \n' Your ECal module must already be connected via USB to the PNA. \nscpi.Execute \"sens:corr:coll:guid:ckit:port1 \"\"N4691-60004 ECal\"\" \" \nscpi.Execute \"sens:corr:coll:guid:ckit:port2 \"\"N4691-60004 User 1 ECal\"\" \" \nMsgBox \"Cal kits defined for Ports 1 and 2\" \n' Initiate the calibration and query the number of steps \nscpi.Execute \"sens:corr:coll:guid:init\" \nnumSteps = scpi.Execute(\"sens:corr:coll:guid:steps?\") \nMsgBox \"Number of steps is \" + CStr(numSteps) \n' Measure the standards \nFor i = 1 To numSteps \nstep = \"Step \" + CStr(i) + \" of \" + CStr(numSteps) \nstrPrompt = scpi.Execute(\"sens:corr:coll:guid:desc? \" + CStr(i)) \nMsgBox strPrompt, vbOKOnly, step \nscpi.Execute \"sens:corr:coll:guid:acq STAN\" + CStr(i) \n1931\n\nNext \n' Conclude the calibration \nscpi.Execute \"sens:corr:coll:guid:save\" \nMsgBox \"Cal is done!\" \n1932\n\nPerform Guided Mechanical Cal using SCPI \nThis VBScript program performs a Guided Calibration using Mechanical standards. While this example is good to \nuse as a starting point for guided mechanical cal, the Guided comprehensive cal example has some advanced \nfeatures that are not in this program. \nThe SCPI commands in this example are sent over a COM interface using the SCPIStringParser object. You do \nNOT need a GPIB connection to run this example. \nThis VBScript (*.vbs) program can be run as a macro in the PNA. To do this, copy the following code into a text \neditor file such as Notepad and save it on the PNA hard drive as Guided.vbs. Learn how to setup and run the \nmacro. \n' Performing a 2-port cal (Ports 1 and 2) \nDim app \nDim scpi \n' Create / Get the PNA application. \nSet app = CreateObject(\"AgilentPNA835x.Application\") \nSet scpi = app.ScpiStringParser \n' Specify the DUT connectors \nscpi.Execute \"sens:corr:coll:guid:conn:port1 \"\"APC 3.5 female\"\" \" \nscpi.Execute \"sens:corr:coll:guid:conn:port2 \"\"APC 3.5 male\"\" \" \n' Note: If your PNA has more than 2 ports, you would need to uncomment \n' one or both of these next two lines, to explicitly specify this is \n' just a 2-port cal. \n'scpi.Execute \"sens:corr:coll:guid:conn:port3 \"\"Not used\"\" \" \n'scpi.Execute \"sens:corr:coll:guid:conn:port4 \"\"Not used\"\" \" \nMsgBox \"Connectors defined for Ports 1 and 2\" \n' Select the Cal Kit for each port being calibrated. \nscpi.Execute \"sens:corr:coll:guid:ckit:port1 \"\"85052D\"\" \" \nscpi.Execute \"sens:corr:coll:guid:ckit:port2 \"\"85052D\"\" \" \nMsgBox \"Cal kits defined for Ports 1 and 2\" \n' Initiate the calibration and query the number of steps \nscpi.Execute \"sens:corr:coll:guid:init\" \nnumSteps = scpi.Execute(\"sens:corr:coll:guid:steps?\") \nMsgBox \"Number of steps is \" + CStr(numSteps) \n' Measure the standards \n'The following series of commands shows that standards \n'can be measured in any order. These steps acquire \n'measurement of standards in reverse order. \n'It is easiest to iterate through standards using \n'a For-Next Loop. \nFor i = numSteps To 1 \nstep = \"Step \" + CStr(i) + \" of \" + CStr(numSteps) \nstrPrompt = scpi.Execute(\"sens:corr:coll:guid:desc? \" + CStr(i)) \nMsgBox strPrompt, vbOKOnly, step \n1933\n\nscpi.Execute \"sens:corr:coll:guid:acq STAN\" + CStr(i) \nNext \n' Conclude the calibration \nscpi.Execute \"sens:corr:coll:guid:save\" \nMsgBox \"Cal is done!\" \nLast Modified: \n20-Jan-2007 Added note about any order for steps. \n1934\n\nPerform a Guided 1-Port Cal on Port 2 \nThis VBScript program does the following: \nClear measurements from the PNA 1. \nCreate a new S22 measurement 2. \nSet an instrument state 3. \nSelect the connector types 4. \nSelect a cal kit 5. \nInitiate a Guided calibration 6. \nDisplay a prompt to connect each standard 7. \nSave the calibration to a newly created cal set 8. \nNote: This example illustrates an important step when calibrating a reflection measurement in the reverse direction. \nYou MUST create a reverse (S22) measurement and have it be the active (selected) measurement on the channel \nthat is being calibrated. This is not necessary for any calibrating any other measurement parameter. \nThe SCPI commands in this example are sent over a COM interface using the SCPIStringParser object. You do \nNOT need a GPIB connection to run this example. \nThis VBScript (*.vbs) program can be run as a macro in the PNA. To do this, copy the following code into a text \neditor file such as Notepad and save it on the PNA hard drive as Guided.vbs. Learn how to setup and run the \nmacro. \nDim App \nSet App = CreateObject(\"AgilentPNA835x.Application\") \nApp.Preset \nDim step \nDim Parser \nDim prompt \nDim txtDat \nDim Chan \nRem Clear old measurements \nApp.Reset \nRem Create a new Measurement \nSet Parser = App.SCPIStringParser \nParser.Parse \"DISPlay:WINDow1:STATE ON\" \nParser.Parse \"CALCulate:PARameter:DEFine 'MyMeas',S22\" \nParser.Parse \"DISPlay:WINDow1:TRACe1:FEED 'MyMeas'\" \nRem Initialize state \nSet Chan = App.ActiveChannel \nChan.StartFrequency = 200e6 \n1935\n\nChan.StopFrequency = 1.5e9 \nChan.IFBandwidth = 1000 \nstep = 3 \nRem Begin a guided calibration \nParser.Parse \"SENS:CORR:COLL:GUID:CONN:PORT1 'Not used'\" \nParser.Parse \"SENS:CORR:COLL:GUID:CONN:PORT2 'Type N (50) male'\" \nParser.Parse \"SENS:CORR:COLL:GUID:CKIT:PORT1 ''\" \nParser.Parse \"SENS:CORR:COLL:GUID:CKIT:PORT2 '85054D'\" \nParser.Parse \"SENS:CORR:COLL:GUID:INIT\" \nRem Query the number of steps \ntxtDat = Parser.Parse(\"SENS:CORR:COLL:GUID:STEP?\") \nRem Display the number of steps \nMsgBox(\"Number of steps is \" + txtDat) \nRem Set the loop counter limit \nstep = txtDat \nRem Measure the standards \nFor i = 1 To step \nIf i= 1 Then \nprompt = Parser.Parse(\"sens:corr:coll:guid:desc? 1\") \nMsgBox(prompt) \nParser.Parse (\"sens:corr:coll:guid:acq STAN1\") \nElseIf i = 2 then \nprompt = Parser.Parse(\"sens:corr:coll:guid:desc? 2\") \nMsgBox(prompt) \nParser.Parse (\"sens:corr:coll:guid:acq STAN2\") \nElseIf i = 3 then \nprompt = Parser.Parse(\"sens:corr:coll:guid:desc? 3\") \nMsgBox(prompt) \nParser.Parse (\"sens:corr:coll:guid:acq STAN3\") \nEnd If \nNext \nRem All standards have been measured. Save the result \nParser.Parse \"SENS:CORR:COLL:GUID:SAVE\" \nMsgBox(\"The calibration has been completed\") \n1936\n\nPerform Guided TRL Calibration \nThis VBScript file performs a 2-Port Guided TRL calibration on 2-port PNA analyzers. (See an example of TRL cal \non a 4-port PNA.) This program does the following: \nClear old measurements from the PNA \nCreate a new S22 measurement \nSet an instrument state \nSelect the connectors and cal kit \nInitiate a Guided calibration \nDisplay a prompt as each new standard must be connected \nSave the calibration to a newly created cal set. \nNote: This program runs without error on all PNA code revisions 7.21 and higher. \nThe SCPI commands in this example are sent over a COM interface using the SCPIStringParser object. You do \nNOT need a GPIB connection to run this example. \nThis VBScript (*.vbs) program can be run as a macro in the PNA. To do this, copy the following code into a text \neditor file such as Notepad and save it on the PNA hard drive as TRL.vbs. Learn how to setup and run the macro. \nDim App \nDim Parser \nDim Chan \nDim txtDat \nDim step \nDim parserTxt \nDim prompt \nSet App = CreateObject(\"AgilentPNA835x.Application\") \n' Clear old measurements \nApp.Reset \n' Create a new Measurement \nSet Parser = App.SCPIStringParser \nParser.Parse \"DISPlay:WINDow1:STATE ON\" \nParser.Parse \"CALCulate:PARameter:DEFine 'MyMeas',S12\" \nParser.Parse \"DISPlay:WINDow1:TRACe1:FEED 'MyMeas'\" \n' Initialize state \nSet Chan = App.ActiveChannel \n1937\n\nChan.StartFrequency = 18.0e9 \nChan.StopFrequency = 20.0e9 \nChan.IFBandwidth = 1000 \n' Begin a guided calibrations \nParser.Parse \"SENS:CORR:COLL:GUID:CONN:PORT1 'APC 3.5 male'\" \nParser.Parse \"SENS:CORR:COLL:GUID:CONN:PORT2 'APC 3.5 female'\" \nParser.Parse \"SENS:CORR:COLL:GUID:CKIT:PORT1 '85052C'\" \nParser.Parse \"SENS:CORR:COLL:GUID:CKIT:PORT2 '85052C'\" \n' Select TRL cal method. \nParser.Parse \"SENS:CORR:COLL:GUID:PATH:CMET 1,2,'TRL'\" \ntxtDat = Parser.Parse(\"SENS:CORR:COLL:GUID:PATH:CMET? 1,2\") \nMsgBox(\"Method \" + txtDat) \nParser.Parse \"SENS:CORR:COLL:GUID:INIT\" \n' Query the number of steps \ntxtDat = Parser.Parse(\"SENS:CORR:COLL:GUID:STEP?\") \n' Display the number of steps \nMsgBox(\"Number of steps is \" + txtDat) \n' Set the loop counter limit \nstep = CInt(txtDat) \n' Measure the standards \nFor i = 1 To step \nparserTxt = \"sens:corr:coll:guid:desc? \" + CStr(i) \nprompt = Parser.Parse(parserTxt) \nMsgBox(prompt) \nparserTxt = \"sens:corr:coll:guid:acq STAN\" + CStr(i) \nParser.Parse (parserTxt) \nNext \n' All standards have been measured. Save the result \nParser.Parse \"SENS:CORR:COLL:GUID:SAVE\" \nMsgBox(\"The TRL calibration has been completed\") \nLast Modified: \n9-Apr-2007 MX Updated for new CMethod command \n1938\n\nPerform Unknown Thru or TRL Cal \nThe following program performs either a 2-port SOLT Unknown Thru Cal or a 2-port TRL Cal. The 85052C Cal Kit \nused in this program contains both types of standards. This program can be run on 2-port or 4-port PNAs. When \nrun on a multiport (4 or more ports) PNA, which does not have a reference receiver per port, a Delta Match Cal is \nrequired. \nSee example of Delta Match Cal. \nSee the Guided Cal commands \nThis VBScript (*.vbs) program can be run as a macro in the PNA. To do this, copy the following code into a text \neditor file such as Notepad and save it on the PNA hard drive as Unknown.vbs. Learn how to setup and run the \nmacro. \nSub PerformUnknownThruOrTRLCal() \nSet pna = CreateObject(\"AgilentPNA835x.Application\") \nSet scpi = pna.ScpiStringParser \n' Specify connectors for Ports 1 and 2 \nscpi.Parse \"SENS:CORR:COLL:GUID:CONN:PORT1 'APC 3.5 female'\" \nscpi.Parse \"SENS:CORR:COLL:GUID:CONN:PORT2 'APC 3.5 male'\" \n'If your PNA has 3 or 4 ports, uncomment one or both of \n'these next two lines, to explicitly specify this is a 2-port cal. \n'scpi.Parse \"SENS:CORR:COLL:GUID:CONN:PORT3 'Not used'\" \n'scpi.Parse \"SENS:CORR:COLL:GUID:CONN:PORT4 'Not used'\" \n' Specify cal kit for Ports 1 and 2 \nscpi.Parse \"SENS:CORR:COLL:GUID:CKIT:PORT1 '85052C'\" \nscpi.Parse \"SENS:CORR:COLL:GUID:CKIT:PORT2 '85052C'\" \n' Since the 85052C cal kit contains SOLT standards and also TRL \n' standards, these next two lines set cal and thru method \nscpi.Execute \"SENS:CORR:COLL:GUID:PATH:CMEThod 1,2,\"SOLT\" \nscpi.Execute \"SENS:CORR:COLL:GUID:PATH:TMEThod 1,2,\"UNKN\" \n' To set up the cal as TRL, comment the previous line and uncomment \n' this next line. The TMEThod is set by default \n'scpi.Execute \"SENS:CORR:COLL:GUID:PATH:CMEThod 1,2,\"TRL\" \n' Initiate the calibration \nscpi.Parse \"SENS:CORR:COLL:GUID:INIT\" \n' Query the list of ports that need delta match \nretStr = scpi.Parse(\"SENS:CORR:COLL:GUID:DMAT:APPL:PORT?\") \nportList = Split(retStr, \",\") \n' If portList contains just one element and it's value is 0, then that indicates \n' none of the ports being calibrated require delta match data. \n' Note: if each testport on the PNA has it's own reference receiver (R channel), \n' then delta match is never needed, so portList will always be just 0. \nlowerBound = LBound(portList) \nIf (UBound(portList) <> lowerBound) Or (CInt( portList(lowerBound) ) <> 0) Then \n1939\n\n' Delta match data is required for at least one port. \n' For this example, we assume a Global Delta Match Cal has previously been \n' performed so the Global Delta Match CalSet exists. \n' The Global Delta Match CalSet is used when the APPL command is invoked \n' without a specific calset ID (GUID). \nscpi.Parse \"SENS:CORR:COLL:GUID:DMAT:APPL\" \nEnd If \n' Query the number of calibration steps \nretStr = scpi.Parse(\"SENS:CORR:COLL:GUID:STEP?\") \nnumSteps = CInt(retStr) \n' Measure the cal standards \nFor i = 1 To numSteps \nprompt = scpi.Parse(\"SENS:CORR:COLL:GUID:DESC? \" & CStr(i)) \nretVal = MsgBox(prompt, vbOKCancel) \nIf retVal = vbCancel Then Exit Sub \nretStr = scpi.Parse(\"SENS:CORR:COLL:GUID:ACQ STAN\" & CStr(i) & \";*OPC?\") \nNext \n' Compute the error coefficients and save the cal to CalSet, and turn it on \nscpi.Parse \"SENS:CORR:COLL:GUID:SAVE\" \nMsgBox \"Cal is done!\" \nEnd Sub \nLast Modified: \n14-May-2007 MX Updated for new CMET and TMET commands \n1940\n\nPerform Global Delta Match Cal \nThe following program performs a Global Delta Match Calibration. This is required when performing an Unknown \nThru Cal or TRL Cal on PNAs without a reference receiver for each test port. See example of Unknown Thru or \nTRL Cal. \nThis VBScript (*.vbs) program can be run as a macro in the PNA. To do this, copy the following code into a text \neditor file such as Notepad and save it on the PNA hard drive as Delta.vbs. Learn how to setup and run the macro. \nSub PerformGlobalDeltaMatchCal() \nSet pna = CreateObject(\"AgilentPNA835x.Application\") \nSet scpi = pna.ScpiStringParser \n' Initiate a Global Delta Match calibration, choosing connector and cal kit \nscpi.Parse \"SENS:CORR:COLL:GUID:DMAT 'APC 3.5 female', '85033D/E'\" \n' Query the number of calibration steps \nretStr = scpi.Parse(\"SENS:CORR:COLL:GUID:STEP?\") \nnumSteps = CInt(retStr) \n' Measure the cal standards \nFor i = 1 To numSteps \nprompt = scpi.Parse(\"SENS:CORR:COLL:GUID:DESC? \" & CStr(i)) \nretVal = MsgBox(prompt, vbOKCancel) \nIf retVal = vbCancel Then Exit Sub \nretStr = scpi.Parse(\"SENS:CORR:COLL:GUID:ACQ STAN\" & CStr(i) & \";*OPC?\") \nNext \n' Compute the error coefficients and save the cal to Global Delta Match CalSet \nscpi.Parse \"SENS:CORR:COLL:GUID:SAVE\" \nMsgBox \"Cal is done!\" \nEnd Sub \n1941\n\nPerform an Unguided ECal \nThis VBScript program performs an Unguided Full 2-Port ECal. \nThe SCPI commands in this example are sent over a COM interface using the SCPIStringParser object. You do \nNOT need a GPIB connection to run this example. \nThis VBScript (*.vbs) program can be run as a macro in the PNA. To do this, copy the following code into a text \neditor file such as Notepad and save it on the PNA hard drive as Unguided.vbs. Learn how to setup and run the \nmacro. \nSet pna = CreateObject(\"AgilentPNA835x.Application\") \nSet scpi = pna.ScpiStringParser \n' Preset the analyzer \nscpi.Execute \"SYSTem:PRESet\" \n' Start frequency of 10 MHz \nscpi.Execute \"SENSe:FREQuency:STARt 10E6\" \n' Stop frequency of 9 GHz \nscpi.Execute \"SENSe:FREQuency:STOP 9E9\" \n' Select the preset S11 measurement \nscpi.Execute \"CALCulate:PARameter:SELect 'CH1_S11_1'\" \n' Read the information about the Agilent factory \n' characterization data of ECal module #1 on the USB bus \nmodule1Info = scpi.Execute(\"SENSe:CORRection:COLLect:CKIT:INFormation? ECAL1,CHAR0\") \n' Prompt for the ECal module \nMsgBox \"Description of ECal Module #1:\" & Chr(10) & Chr(10) & module1Info & _Chr(10) \n& Chr(10) & \"Make port connections to the ECal module, then press enter\" \n' ECal full 1 port and 2 port \n' Choose a Calibration Type (comment out one of these) \nscpi.Execute \"SENSe:CORRection:COLLect:METHod refl3\" \nscpi.Execute \"SENSe:CORRection:COLLect:METHod SPARSOLT\" \n' Specify to have the PNA automatically determine which port of the \n' ECal module is connected to which port of the PNA. \nscpi.Execute \"SENSe:CORRection:PREFerence:ECAL:ORIentation ON\" \n' Alternatively, if you are measuring at very low power levels where \n' the PNA fails to sense the module's orientation, you may need to turn \n' off the auto orientation and specify how the module is connected (as in \n' these next two commented lines of code -- \"A1,B2\" would indicate Port A \n' of the module is connected to Port 1 and Port B is connected to Port 2). \n'scpi.Execute \"SENSe:CORRection:PREFerence:ECAL:ORIentation OFF\" \n'scpi.Execute \"SENSe:CORRection:PREFerence:ECAL:PMAP ECAL1,'A1,B2'\" \n' Acquire and store the calibration terms. *OPC? causes a \"+1\" to be \n' returned when finished. CHAR0 indicates to use the Agilent factory \n' characterized data within the ECal module (as opposed to a user characterization). \nx = scpi.Execute(\"SENSe:CORRection:COLLect:ACQuire ECAL1,CHAR0;*OPC?\") \nMsgBox \"Done with calibration.\" \n1942\n\nPerform an Unguided 2-Port Mechanical Cal \nThis VBScript program performs an Unguided, Full 2-Port, calibration using ONE set of mechanical calibration \nstandards. \nThe SCPI commands in this example are sent over a COM interface using the SCPIStringParser object. You do \nNOT need a GPIB connection to run this example. \nThis VBScript (*.vbs) program can be run as a macro in the PNA. To do this, copy the following code into a text \neditor file such as Notepad and save it on the PNA hard drive as Unguided.vbs. Learn how to setup and run the \nmacro. \nSet App = CreateObject(\"AgilentPNA835x.Application\") \nSet Scpi = App.SCPIStringParser \n'Initialize state \nScpi.Execute (\"SYSTem:PRESet\") \n'Select the Preset measurement \nScpi.Execute (\"CALCulate:PARameter:SELect 'CH1_S11_1'\") \n'Set the calibration method \nScpi.Execute (\"SENSe:CORRection:COLLect:METHod SPARSOLT\") \n'Select a cal kit \nScpi.Execute (\"SENSe:CORRection:COLLect:CKIT:SELect 1\") \n'Set one set of standards \nScpi.Execute (\"SENSe:CORRection:TSTandards OFF\") \n'Set acquisition to FORWARD \nScpi.Execute (\"SENSe:CORRection:SFORward ON\") \n'Measure the standards in forward direction \nMsgBox \"Connect OPEN to Port 1; then press OK\" \nScpi.Execute (\"SENSe:CORRection:COLLect:ACQuire stan1\") \nMsgBox \"Connect SHORT to Port 1; then press OK\" \nScpi.Execute (\"SENSe:CORRection:COLLect:ACQuire stan2\") \nMsgBox \"Connect LOAD to Port 1; then press OK\" \nScpi.Execute (\"SENSe:CORRection:COLLect:ACQuire stan3\") \n'Set acquisition to REVERSE \nScpi.Execute (\"SENSe:CORRection:SFORward OFF\") \n'Measure the standards in reverse direction \nMsgBox \"Connect OPEN to Port 2; then press OK\" \nScpi.Execute (\"SENSe:CORRection:COLLect:ACQuire stan1\") \nMsgBox \"Connect SHORT to Port 2; then press OK\" \nScpi.Execute (\"SENSe:CORRection:COLLect:ACQuire stan2\") \n1943\n\nMsgBox \"Connect LOAD to Port 2; then press OK\" \nScpi.Execute (\"SENSe:CORRection:COLLect:ACQuire stan3\") \n'Measure the thru standard \nMsgBox \"Connect THRU between Ports 1 and 2; then press OK\" \nScpi.Execute (\"SENSe:CORRection:COLLect:ACQuire stan4\") \n'OPTIONAL Measure Isolation \nMsgBox \"Connect LOADS to Port 1 AND Port 2; then press OK\" \nScpi.Execute (\"SENSe:CORRection:COLLect:ACQuire stan5\") \n'All standards have been measured. Save the result \nScpi.Execute (\"SENS:CORR:COLL:SAVE\") \nMsgBox \"The calibration has been completed\" \n1944\n\nPerform an Unguided 1-Port Cal on Port 2 \nThis VBScript program does the following: \nClear measurements from the PNA 1. \nCreate a new S22 measurement 2. \nSet an instrument state 3. \nSelect a cal kit 4. \nInitiate an Unguided calibration 5. \nDisplay a prompt to connect each standard 6. \nSave the calibration to a newly created cal set 7. \nNote: This example illustrates an important step when calibrating a reflection measurement in the reverse direction. \nYou MUST create a reverse (S22) measurement and have it be the active (selected) measurement on the channel \nthat is being calibrated. This is not necessary for any calibrating any other measurement parameter. \nThe SCPI commands in this example are sent over a COM interface using the SCPIStringParser object. You do \nNOT need a GPIB connection to run this example. \nThis VBScript (*.vbs) program can be run as a macro in the PNA. To do this, copy the following code into a text \neditor file such as Notepad and save it on the PNA hard drive as Unguided.vbs. Learn how to setup and run the \nmacro. \nDim App \nSet App = CreateObject(\"AgilentPNA835x.Application\") \nApp.Preset \nDim Parser \nDim Chan \nRem Clear old measurements \nApp.Reset \nRem Create a new Measurement \nSet Parser = App.SCPIStringParser \nParser.Parse \"DISPlay:WINDow1:STATE ON\" \nParser.Parse \"CALCulate:PARameter:DEFine 'MyMeas',S22\" \nParser.Parse \"DISPlay:WINDow1:TRACe1:FEED 'MyMeas'\" \nRem Initialize state \nSet Chan = App.ActiveChannel \nChan.StartFrequency = 200e6 \nChan.StopFrequency = 1.5e9 \nChan.IFBandwidth = 1000 \nRem Begin an unguided calibration \n1945\n\nRem Set the calibration method \nParser.Parse \"SENSe:CORRection:COLLect:METHod REFL3\" \nRem Turn off continuous sweep \nParser.Parse \"INITiate:CONTinuous OFF\" \nRem Select a cal kit \nParser.Parse \"SENSe:CORRection:COLLect:CKIT:SELect 1\" \nRem Measure the standards \nMsgBox(\"Connect OPEN to port 2. Then press OK\") \nParser.Parse (\"sens:corr:coll:acq STAN1\") \nMsgBox(\"Connect SHORT to port 2. Then press OK\") \nParser.Parse (\"sens:corr:coll:acq STAN2\") \nMsgBox(\"Connect LOAD to port 2. Then press OK\") \nParser.Parse (\"sens:corr:coll:acq STAN3\") \nRem All standards have been measured. Save the result \nParser.Parse \"SENS:CORR:COLL:SAVE\" \nRem Turn ON continuous sweep \nParser.Parse \"INITiate:CONTinuous ON\" \nMsgBox(\"The calibration has been completed\") \n1946\n\nPerform an Unguided Cal on a 4-Port PNA \nThis topic describes how to perform an unguided calibration on a multiport network analyzer using SCPI. The \nobjective here is to make clear the relationship between the physical port on which a standard is being measured, \nthe actual device in the cal kit, and the SCPI command used to acquire the device. \nThere are two sets of SCPI commands that acquire calibrations. One set is used for guided cal, the other for \nunguided. The SCPI commands that provide remote access to unguided cal are in the SENS:CORR:COLL block: \nSENS:CORR:COLL:METHod \nSENS:CORR:COLL:ACQuire \nSENS:CORR:COLL:SAVE \nOn a four port network analyzer, the remote programmer needs to be aware of the relationship between the \nphysical port and the calibration kit class assignments. The example program (below) illustrates the usage by \nperforming three unique 2 port cals, taking care to acquire the appropriate standards. \nCalibration standards classes are �categories� of standard types. To perform a 2 port calibration, the cal wizard \nrequires the user to measure: \n3 reflection standards on the forward port: \nClass S11A typically an open \nClass S11B typically a short \nClass S11C typically a load \nLikewise, 3 reflection standards are required for the reverse port: \nClass S22A typically an open \nClass S22B typically a short \nClass S22C typically a load \nThere is also a transmission standard that is measured in both directions: \nClass S21T typically a thru \nThe following illustrates the relationship between cal kit physical standards and calibration classes. \nHere is a list of the physical devices in my calibration kit. \nStandard #1 = \"3.5 mm male short\" \nStandard #2 = \"3.5 mm male open\" \nStandard #3 = \"3.5 mm male broadband load\" \nStandard #4 = \"Insertable thru standard\" \n1947\n\nStandard #5 = \"3.5 mm male sliding load\" \nStandard #6 = \"3.5 mm male lowband load\" \nStandard #7 = \"3.5 mm female short\" \nStandard #8 = \"female to female characterized thru adapter\" \nStandard #9 = \"0-2 Load\" \nStandard #10 = \"Open\" \nStandard #11 = \"Non-insertable thru\" \nStandard #12 = \"3.5 mm female lowband load\" \nStandard #13 = \"3.5 mm female sliding load\" \nStandard #14 = \"3.5 mm female broadband load\" \nStandard #15 = \"3.5 mm female open\" \nWhen you perform a calibration remotely using SCPI, you don�t specify the device number directly. Rather, you \nspecify the class you want to measure. Each device in the calibration kit is assigned to a class. And since more \nthan one device can be assigned to the same class, each class contains an ordered list of devices. The class \nassignments are user-settable using the Advanced Modify Cal Kit dialog or the SCPI command: \nSENS:CORR:COLL:CKIT:ORDer<class>, <std>, <std>, <std>, <std>,<std>,<std>,<std> \nThe 85052B kit used in the example program had the following standard list for each class: The list was obtained \nby issuing the corresponding SCPI query: \nSENS:CORR:COLL:CKIT:OLIST1? S11A = +2,+15,+0,+0,+0,+0,+0 \nSENS:CORR:COLL:CKIT:OLIST2? S11B = +1,+7,+0,+0,+0,+0,+0 \nSENS:CORR:COLL:CKIT:OLIST3? S11C = +6,+5,+3,+12,+13,+14,+0 \nSENS:CORR:COLL:CKIT:OLIST4? S21T = +4,+8,+0,+0,+0,+0,+0 \nSENS:CORR:COLL:CKIT:OLIST5? S22A = +2,+15,+0,+0,+0,+0,+0 \nSENS:CORR:COLL:CKIT:OLIST6? S22B = +1,+7,+0,+0,+0,+0,+0 \nSENS:CORR:COLL:CKIT:OLIST7? S22C = +6,+5,+3,+12,+13,+14,+0 \nSENS:CORR:COLL:CKIT:OLIST8? S12T = +4,+8,+0,+0,+0,+0,+0 \nWhen you perform the calibration, you acquire data by issuing the ACQuire command: \nSENS:CORR:COLL:ACQ <class>[, <subst> ] \nFor example: \nSENS:CORR:COLL:SFOR 1 \nSENS:CORR:COLL:ACQ STANA, SST2 \nThe SFOR command tells the wizard to make the next acquisition in the forward direction. The ACQuire command \nspecifies that we are measuring the 2nd device in the list for STANA. And since we are measuring SFORward, \nSTANA refers to class #1 or S11A. The list of devices for this class are specified in the OLIST1 query above. The \nassociations are shown in red. \nAlternately, you could modify the device order for the S11A class to move device #15 into the first position \n(SENS:CORR:COLL:CKIT:ORDER1). When the desired device is in the first position, you needn�t specify the \norder number in the ACQuire command. The default is the first device in the OLIST. This worked well for two port \nnetwork analyzers where the order for S11A,B,C classes were setup for port 1 and the order for S22A,B,C was set \nup for port 2. With the kit setup in the proper order, you could eliminate the specification of the substandard \n1948\n\nnumber (SST<n>). \nWhen performing 2 port calibrations on 4 Port Network Analyzers (e.g.: PNA Model N5230A), the wizard applies \nS11A,B,C standards to the lower numbered port, S22A,B,C standards to the higher numbered port. Since the two \nclasses (S11A,B,C and S22A,B,C) are applied to multiple ports, the programmer must take into account the ports \nbeing measured and take greater care when specifying the ACQuire command to ensure that the correct device is \nbeing measured. \nPort to class relationship \nPorts S11A Port S22A Port \n1,2 1 2 \n1,3 1 3 \n1,4 1 4 \n2,3 2 3 \n2,4 2 4 \n3,4 3 4 \nThe following example program shows one method of handling two port cals on a multiport network analyzer. The \nconnectors at the measurement plane are assumed to be (1) male, (2) female, (3) male, and (4) male. In the \nexample, three cals are performed: 1-2 (insertable male to female), 2-3 (insertable female to male), and 3-4 \n(noninsertable using an characterized adapter). \noption explicit \npublic scpi \npublic pna \n' assume a 4 port PNA with the following connectors: \n' the standard measured on these ports will be the opposite gender \n' PORT 1 = 3.5 male \n' PORT 2 = 3.5 female \n' PORT 3 = 3.5 male \n' PORT 4 = 3.5 male \n'To perform 2 port calibrations between 1-2, 2-3, and 3-4 you need to do the \nfollowing \ncall main \nsub main \nset pna = CreateObject(\"AgilentPnA835x.Application\") \nset scpi = pna.ScpiStringParser \npna.Preset \n' select a kit to use for this demonstration \n' kit #1 for the N5230A is the 85052B 3.5mm kit with sliding load \nscpi.execute(\"SENS:CORR:COLL:CKIT:SELECT 1\" ) \n1949\n\nPrintKitStandardInfo 1 \nPrintKitOlist 1 \n' -------------------------------------------- \n' CALIBRATE PORTS 1 and 2, insertable cal \n' -------------------------------------------- \nwscript.echo \nwscript.echo \"Calibrating ports 1 and 2\" \nscpi.execute(\"SYST:PRES;\") \nscpi.execute(\"calc:par:sel CH1_S11_1\") \nscpi.execute(\"SENS:CORR:TST:STATE 0\") \nscpi.execute(\"SENS:CORR:COLL:METHod SPARSOLT\") \nscpi.execute(\"SENS:CORR:SFOR 1\") \nMeasureFemaleStandards 1 \nscpi.execute(\"SENS:CORR:SFOR 0\") \nMeasureMaleStandards 2 \nMeasureTransmissionStandards 1,2 \nscpi.execute(\"SENS:CORR:COLL:SAVE\") \n' -------------------------------------------- \n' CALIBRATE PORTS 2 and 3, insertable cal \n' -------------------------------------------- \nwscript.echo \nwscript.echo \"Calibrating ports 2 and 3\" \nscpi.execute(\"SYST:PRES;\") \nscpi.execute(\"calc:par:sel CH1_S11_1\") \nscpi.execute(\"calc:par:mod S23\") \nscpi.execute(\"SENS:CORR:TST:STATE 0\") \nscpi.execute(\"SENS:CORR:COLL:METHod SPARSOLT\") \nscpi.execute(\"SENS:CORR:SFOR 1\") \nMeasureMaleStandards 2 \nscpi.execute(\"SENS:CORR:SFOR 0\") \nMeasureFemaleStandards 3 \nMeasureTransmissionStandards 2,3 \nscpi.execute(\"SENS:CORR:COLL:SAVE\") \n' -------------------------------------------- \n' CALIBRATE PORTS 3 and 4, non-insertable cal \n' -------------------------------------------- \nwscript.echo \nwscript.echo \"Calibrating ports 3 and 4\" \nscpi.execute(\"SYST:PRES;\") \nscpi.execute(\"calc:par:sel CH1_S11_1\") \nscpi.execute(\"calc:par:mod S43\") \nscpi.execute(\"SENS:CORR:COLL:METHod SPARSOLT\") \nscpi.execute(\"SENS:CORR:SFOR 1\") \nMeasureFemaleStandards 3 \nscpi.execute(\"SENS:CORR:SFOR 0\") \nMeasureFemaleStandards 4 \nMeasureAdapter 3, 4 \nscpi.execute(\"SENS:CORR:COLL:SAVE\") \nend sub \n1950\n\nsub MeasureMaleStandards ( portNumber ) \ndim portstr \nportstr = formatnumber(portNumber,0) \nPromptconnect1 1, 1, portNumber \nscpi.execute(\"SENS:CORR:COLL:ACQ STAN1;*OPC?\") \nPromptconnect1 2, 1, portNumber \nscpi.execute(\"SENS:CORR:COLL:ACQ STAN2;*OPC?\") \nPromptconnect1 3, 3, portNumber \nscpi.execute(\"SENS:CORR:COLL:ACQ STAN3,SST3;*OPC?\") \nend sub \nsub MeasureFemaleStandards (portNumber) \ndim portstr \nportstr = formatnumber(portNumber,0) \nPromptconnect1 1, 2, portNumber \nscpi.execute(\"SENS:CORR:COLL:ACQ STAN1,SST2;*OPC?\") \nPromptconnect1 2, 2, portNumber \nscpi.execute(\"SENS:CORR:COLL:ACQ STAN2,SST2;*OPC?\") \nPromptconnect1 3, 6, portNumber \nscpi.execute(\"SENS:CORR:COLL:ACQ STAN3,SST6;*OPC?\") \nend sub \nsub MeasureTransmissionStandards( port1, port2) \ndim p1str \ndim p2str \np1str = formatnumber( port1, 0) \np2str = formatnumber( port2, 0) \nPromptconnect2 4, 1, port1, port2 \nscpi.execute(\"SENS:CORR:COLL:ACQ STAN4;*OPC?\") \nend sub \nsub MeasureAdapter( port1, port2) \ndim p1str \ndim p2str \np1str = formatnumber( port1, 0) \np2str = formatnumber( port2, 0) \nPromptconnect2 4, 2, port1, port2 \nscpi.execute(\"SENS:CORR:COLL:ACQ STAN4,SST2;*OPC?\") \nend sub \n' return the nth item in the comma separated list \nFunction GetItemNumber( list, n) \ndim strVector \nstrVector = split(list,\",\",-1,1) \nGetItemNumber = strVector(n-1) \nend function \n' remove the trailing newline from str \nfunction chop( str ) \n1951\n\ndim tmp \ntmp = str \n' remove the appended newline \ndim pos \npos = InStrRev(tmp,vblf) \nif (pos >0) then \ntmp = mid(tmp,1,pos-1) \nend if \nchop = tmp \nend function \n'return the label for the nth standard assigned to the class described by \nclass_index. \n' if class_index = 1, class is S11A (STAN1) \n' if class_index = 2, class is S11B (STAN2), etc \nfunction GetStandardLabel( class_index, nth) \ndim olist \ndim stdnum \ndim resp \nolist = scpi.execute(\"SENS:CORR:COLL:CKIT:OLIST\" + formatnumber(class_index,0)+\"?\") \nstdnum = GetItemNumber( olist, nth) \nscpi.execute(\"SENS:CORR:COLL:CKIT:STAN \" + formatnumber(stdnum,0)) \nresp = scpi.execute(\"SENS:CORR:COLL:CKIT:STAN:LABel?\") \nGetStandardLabel = chop(resp) \nend function \nsub PromptConnect1( class_index, nth, port) \nwscript.echo \"CONNECT \" + GetStandardLabel( class_index, nth) + \" to port \" + \nformatnumber(port,0) \nend sub \nsub PromptConnect2( class_index, nth, port1, port2) \nwscript.echo \"CONNECT \" + GetStandardLabel( class_index, nth) + \" between ports \" + \nformatnumber(port1,0) + \" and \" + formatnumber(port2,0) \nend sub \n' Print the order of standards per class for this kit \nsub PrintKitOlist( kit ) \ndim i \ndim cmd \ndim resp \nwscript.echo \ndim olistcmd \nolistcmd = \"SENS:CORR:COLL:CKIT:OLIST\" \n' list the sub standards for each of the following classes \n' S11A, S11B, S11C, FWD TRANS, FWD ISOL, S22A, S22B, S22C, REV TRANS, REV ISOL \nfor i = 1 to 8 \ncmd = olistcmd + formatNumber(i,0) + \"?\" \nresp = scpi.execute(cmd) \nwscript.echo cmd + \"= \" + chop(resp) \nnext \nend sub \n1952\n\nsub PrintKitStandardInfo( kit ) \nwscript.echo scpi.execute(\"SENS:CORR:COLL:CKIT:NAME?\") \ndim i \nfor i = 1 to 30 \ndim slabel \ndim snum \nsnum = formatNumber(i,0) \nscpi.execute(\"SENS:CORR:COLL:CKIT:STAN \" + snum) \nslabel=scpi.execute(\"SENS:CORR:COLL:CKIT:STAN:LABel?\") \nwscript.echo \"Standard #\"+snum+ \" = \" + chop(slabel) \nnext \nend sub \nThe output from this program is as follows: \nMicrosoft (R) Windows Script Host Version 5.6 \nCopyright (C) Microsoft Corporation 1996-2001. All rights reserved. \n\"85052B 3.5 mm with sliding load\" \nStandard #1 = \"3.5 mm male short\" \nStandard #2 = \"3.5 mm male open\" \nStandard #3 = \"3.5 mm male broadband load\" \nStandard #4 = \"Insertable thru standard\" \nStandard #5 = \"3.5 mm male sliding load\" \nStandard #6 = \"3.5 mm male lowband load\" \nStandard #7 = \"3.5 mm female short\" \nStandard #8 = \"female to female characterized thru adapter\" \nStandard #9 = \"0-2 Load\" \nStandard #10 = \"Open\" \nStandard #11 = \"Non-insertable thru\" \nStandard #12 = \"3.5 mm female lowband load\" \nStandard #13 = \"3.5 mm female sliding load\" \nStandard #14 = \"3.5 mm female broadband load\" \nStandard #15 = \"3.5 mm female open\" \nStandard #16 = \"Open\" \nStandard #17 = \"Open\" \nStandard #18 = \"Open\" \nStandard #19 = \"Open\" \nStandard #20 = \"Open\" \nStandard #21 = \"Open\" \n1953\n\nStandard #22 = \"Open\" \nStandard #23 = \"Open\" \nStandard #24 = \"Open\" \nStandard #25 = \"Open\" \nStandard #26 = \"Open\" \nStandard #27 = \"Open\" \nStandard #28 = \"Open\" \nStandard #29 = \"Open\" \nStandard #30 = \"Open\" \nSENS:CORR:COLL:CKIT:OLIST1?= +2,+15,+0,+0,+0,+0,+0 \nSENS:CORR:COLL:CKIT:OLIST2?= +1,+7,+0,+0,+0,+0,+0 \nSENS:CORR:COLL:CKIT:OLIST3?= +6,+5,+3,+12,+13,+14,+0 \nSENS:CORR:COLL:CKIT:OLIST4?= +4,+8,+0,+0,+0,+0,+0 \nSENS:CORR:COLL:CKIT:OLIST5?= +2,+15,+0,+0,+0,+0,+0 \nSENS:CORR:COLL:CKIT:OLIST6?= +1,+7,+0,+0,+0,+0,+0 \nSENS:CORR:COLL:CKIT:OLIST7?= +6,+5,+3,+12,+13,+14,+0 \nSENS:CORR:COLL:CKIT:OLIST8?= +4,+8,+0,+0,+0,+0,+0 \nCalibrating ports 1 and 2 \nCONNECT \"3.5 mm female open\" to port 1 \nCONNECT \"3.5 mm female short\" to port 1 \nCONNECT \"3.5 mm female broadband load\" to port 1 \nCONNECT \"3.5 mm male open\" to port 2 \nCONNECT \"3.5 mm male short\" to port 2 \nCONNECT \"3.5 mm male broadband load\" to port 2 \nCONNECT \"Insertable thru standard\" between ports 1 and 2 \nCalibrating ports 2 and 3 \nCONNECT \"3.5 mm male open\" to port 2 \nCONNECT \"3.5 mm male short\" to port 2 \nCONNECT \"3.5 mm male broadband load\" to port 2 \nCONNECT \"3.5 mm female open\" to port 3 \nCONNECT \"3.5 mm female short\" to port 3 \nCONNECT \"3.5 mm female broadband load\" to port 3 \nCONNECT \"Insertable thru standard\" between ports 2 and 3 \nCalibrating ports 3 and 4 \nCONNECT \"3.5 mm female open\" to port 3 \nCONNECT \"3.5 mm female short\" to port 3 \n1954\n\nCONNECT \"3.5 mm female broadband load\" to port 3 \nCONNECT \"3.5 mm female open\" to port 4 \nCONNECT \"3.5 mm female short\" to port 4 \nCONNECT \"3.5 mm female broadband load\" to port 4 \nCONNECT \"female to female characterized thru adapter\" between ports 3 and 4 \n1955\n\nPerform an Unguided Cal on Multiple Channels \nThis VBScript program performs an Unguided Calibration simultaneously on two channels. \nThis could be used in the following cases: \nIf you need more than the current number of data points per trace, so the additional points must be added to \na different channel. \nIf you need several channels with independent settings, but you want to calibrate all channels with a minimal \nnumber of standard connections. This would be especially critical for on wafer calibration. \nThe SCPI commands in this example are sent over a COM interface using the SCPIStringParser object. You do \nNOT need a GPIB connection to run this example. \nThis VBScript (*.vbs) program can be run as a macro in the PNA. To do this, copy the following code into a text \neditor file such as Notepad and save it on the PNA hard drive as Unguided.vbs. Learn how to setup and run the \nmacro. \nDim app \nDim scpi \nDim NumberOfActiveChannels \nNumberOfActiveChannels = 2 \n' Create / Get the PNA application. \nSet app = CreateObject(\"AgilentPNA835x.Application\") \nSet scpi = app.ScpiStringParser \n' Query the list of connectors that the PNA system recognizes \nscpi.Execute(\"SYST:PRES\") \n'Wait for successful preset before continuing \ndone=scpi.Execute(\"*OPC?\") \n'The following section sets up 2 channels with different frequency ranges \nscpi.Execute(\"DISP:WIND1:STATE OFF\") \n'Reset Windows \nscpi.Execute(\"DISP:WIND1:STATE ON\") \nscpi.Execute(\"DISP:WIND2:STATE ON\") \n'\n' Assign a measurement to the first window \nscpi.Execute(\"CALC1:PAR:DEF 'Meas1', S21\") \nscpi.Execute(\"DISP:WIND1:TRAC1:FEED 'Meas1'\") \n'Assign a measurement to the second window \nscpi.Execute(\"CALC2:PAR:DEF 'Meas2', S21\") \nscpi.Execute(\"DISP:WIND2:TRAC1:FEED 'Meas2'\") \n1956\n\n'Set up two channels with independent parameters \nscpi.Execute(\"SENS1:FREQ:SPAN 1e9\") \nscpi.Execute(\"SENS2:FREQ:SPAN 1e6\") \n'Wait for changes before continuing \ndone=scpi.Execute(\"*OPC?\") \n'\n'This section sets the calibration kits for channel 1 and channel 2 \n'Select a trace from channel 1 and set calibration type and cal kit \nscpi.Execute(\"CALC1:PAR:SEL 'Meas1'\") \nscpi.Execute(\"SENS1:CORR:COLL:METH SPARSOLT\") \nscpi.Execute(\"SENS1:CORR:COLL:CKIT 2\") '85056D for default settings \n'Same standards for forward and reverse direction \nscpi.Execute(\"SENS1:CORR:TST OFF\") \n'Select a trace from channel 2 and set calibration type and cal kit \nscpi.Execute(\"CALC2:PAR:SEL 'Meas2'\") \nscpi.Execute(\"SENS2:CORR:COLL:METH SPARSOLT\") \nscpi.Execute(\"SENS2:CORR:COLL:CKIT 2\") '85056D for default settings \n'Same standards for forward and reverse direction \nscpi.Execute(\"SENS2:CORR:TST OFF\") \n'Set both channels to manual triggering \nscpi.Execute(\"INIT1:CONT OFF\") \nscpi.Execute(\"INIT2:CONT OFF\") \n'\n'The following assumes female port connector on port 1 \n' and male port connector on port 1 \n'Step through all active channels and calibrate and measure all standards. \nscpi.Execute(\"SENS1:CORR:SFOR ON\") 'Set acquisition to forward \nscpi.Execute(\"SENS2:CORR:SFOR ON\") 'Set acquisition to forward \nMsgBox(\"Connect OPEN standard to port 1\") \nFor CurrentChannel = 1 To NumberOfActiveChannels \nscpi.Execute(\"CALC\" & CurrentChannel & \":PAR:SEL 'Meas\" & CurrentChannel & \"'\") \nscpi.Execute(\"SENS\" & CurrentChannel & \":CORR:COLL stan1\") \ndone= scpi.Execute(\"*OPC?\") \nNext \n1957\n\nMsgBox(\"Connect SHORT standard to port 1\") \nFor CurrentChannel = 1 To NumberOfActiveChannels \nscpi.Execute(\"CALC\" & CurrentChannel & \":PAR:SEL 'Meas\" & CurrentChannel & \"'\") \nscpi.Execute(\"SENS\" & CurrentChannel & \":CORR:COLL stan2\") \ndone=scpi.Execute(\"*OPC?\") \nNext \nMsgBox(\"Connect LOAD standard to port 1\") \nFor CurrentChannel = 1 To NumberOfActiveChannels \nscpi.Execute(\"CALC\" & CurrentChannel & \":PAR:SEL 'Meas\" & CurrentChannel & \"'\") \nscpi.Execute(\"SENS\" & CurrentChannel & \":CORR:COLL stan3\") \ndone=scpi.Execute(\"*OPC?\") \nNext \nscpi.Execute(\"SENS1:CORR:SFOR OFF\") 'Set acquisition to reverse \nscpi.Execute(\"SENS2:CORR:SFOR OFF\") 'Set acquisition to forward \nMsgBox(\"Connect OPEN standard to port 2\") \nFor CurrentChannel = 1 To NumberOfActiveChannels \nscpi.Execute(\"CALC\" & CurrentChannel & \":PAR:SEL 'Meas\" & CurrentChannel & \"'\") \nscpi.Execute(\"SENS\" & CurrentChannel & \":CORR:COLL stan1\") \ndone=scpi.Execute(\"*OPC?\") \nNext \nMsgBox(\"Connect SHORT standard to port 2\") \nFor CurrentChannel = 1 To NumberOfActiveChannels \nscpi.Execute(\"CALC\" & CurrentChannel & \":PAR:SEL 'Meas\" & CurrentChannel & \"'\") \nscpi.Execute(\"SENS\" & CurrentChannel & \":CORR:COLL stan2\") \ndone=scpi.Execute(\"*OPC?\") \nNext \nMsgBox(\"Connect LOAD standard to port 2\") \nFor CurrentChannel = 1 To NumberOfActiveChannels \nscpi.Execute(\"CALC\" & CurrentChannel & \":PAR:SEL 'Meas\" & CurrentChannel & \"'\") \nscpi.Execute(\"SENS\" & CurrentChannel & \":CORR:COLL stan3\") \ndone=scpi.Execute(\"*OPC?\") \nNext \n1958\n\n'\n'Measure thru standard for all channels in both forward and reverse direction \nMsgBox(\"Connect THRU between ports 1 and 2\") \nscpi.Execute(\"SENS1:CORR:SFOR ON\") 'Set acquisition to forward \nscpi.Execute(\"SENS2:CORR:SFOR ON\") 'Set acquisition to forward \nFor CurrentChannel = 1 To NumberOfActiveChannels \nscpi.Execute(\"CALC\" & CurrentChannel & \":PAR:SEL 'Meas\" & CurrentChannel & \"'\") \nscpi.Execute(\"SENS\" & CurrentChannel & \":CORR:COLL stan4\") \ndone=scpi.Execute(\"*OPC?\") \nNext \nscpi.Execute(\"SENS1:CORR:SFOR OFF\") 'Set acquisition to reverse \nscpi.Execute(\"SENS2:CORR:SFOR OFF\") 'Set acquisition to reverse \nFor CurrentChannel = 1 To NumberOfActiveChannels \nscpi.Execute(\"CALC\" & CurrentChannel & \":PAR:SEL 'Meas\" & CurrentChannel & \"'\") \nscpi.Execute(\"SENS\" & CurrentChannel & \":CORR:COLL stan4\") \ndone=scpi.Execute(\"*OPC?\") \nNext \nFor CurrentChannel = 1 To NumberOfActiveChannels \nscpi.Execute(\"CALC\" & CurrentChannel & \":PAR:SEL 'Meas\" & CurrentChannel & \"'\") \nscpi.Execute(\"SENS\" & CurrentChannel & \":CORR:COLL:SAVE\") \ndone=scpi.Execute(\"*OPC?\") \nNext \n'Set both channels to continuous triggering \nscpi.Execute(\"INIT1:CONT ON\") \nscpi.Execute(\"INIT2:CONT ON\") \n1959\n\nECALConfidence Check using SCPI \nThis Visual Basic program performs a complete ECAL confidence check. \nTo run this program, you need: \nAn established GPIB interface connection \nAgilent's VISA or National Instrument's VISA installed on your PC \nThe module visa32.bas added to your VB project. \nA form with two buttons: cmdRun and cmdQuit \nA calibrated S11 1-port or N-port measurement active on Channel 1 \nWindow 1 is visible \nSee Other SCPI Example Programs \n'Session to VISA Default Resource Manager \nPrivate defRM As Long \n'Session to PNA \nPrivate viPNA As Long \n'VISA function status return code \nPrivate status As Long \nPrivate Sub Form_Load() \ndefRM = 0 \nEnd Sub \nPrivate Sub cmdRun_Click() \n'String to receive data from the PNA \nDim strReply As String * 200 \n' Open the VISA default resource manager \nstatus = viOpenDefaultRM(defRM) \nIf (status < VI_SUCCESS) Then HandleVISAError \n' Open a VISA session (viPNA) to the PNA at GPIB address 16. \nstatus = viOpen(defRM, \"GPIB0::16::INSTR\", 0, 0, viPNA) \nIf (status < VI_SUCCESS) Then HandleVISAError \n' Need to set the VISA timeout value to give all our GPIB Reads \n' sufficient time to complete before a timeout error occurs. \n' For this example, let's try setting the limit to \n' 10000 milliseconds (10 seconds). \nstatus = viSetAttribute(viPNA, VI_ATTR_TMO_VALUE, 10000) \nIf (status < VI_SUCCESS) Then HandleVISAError \n' Get the catalog of all the measurements currently on Channel 1. \nstatus = myGPIBWrite(viPNA, \"CALC1:PAR:CAT?\") \nIf (status < VI_SUCCESS) Then HandleVISAError \nstatus = myGPIBRead(viPNA, strReply) \nIf (status < VI_SUCCESS) Then HandleVISAError \n1960\n\n' If an S11 measurement named \"MY_S11\" doesn't already exist, \n' then create it. \nIf InStr(strReply, \"MY_S11\") = 0 Then \nstatus = myGPIBWrite(viPNA, \"CALC1:PAR:DEF MY_S11,S11\") \nIf (status < VI_SUCCESS) Then HandleVISAError \nEnd If \nstrReply = \"\" \n' Get the catalog of all the trace numbers currently active \n' in Window 1. \nstatus = myGPIBWrite(viPNA, \"DISP:WIND1:CAT?\") \nIf (status < VI_SUCCESS) Then HandleVISAError \nstatus = myGPIBRead(viPNA, strReply) \nIf (status < VI_SUCCESS) Then HandleVISAError \n' If a trace number 4 already exists in Window 1, then this \n' will remove it. \nIf InStr(strReply, \"4\") > 0 Then \nstatus = myGPIBWrite(viPNA, \"DISP:WIND1:TRAC4:DEL\") \nIf (status < VI_SUCCESS) Then HandleVISAError \nEnd If \n' Set trace number 4 to MY_S11. \nstatus = myGPIBWrite(viPNA, \"DISP:WIND1:TRAC4:FEED MY_S11\") \nIf (status < VI_SUCCESS) Then HandleVISAError \n' Set up trace view so we are viewing only the data trace. \nstatus = myGPIBWrite(viPNA, \"DISP:WIND1:TRAC4 ON\") \nIf (status < VI_SUCCESS) Then HandleVISAError \nstatus = myGPIBWrite(viPNA, \"DISP:WIND1:TRAC4:MEM OFF\") \nIf (status < VI_SUCCESS) Then HandleVISAError \n' Select MY_S11 as the measurement to be used for the \n' Confidence Check. \nstatus = myGPIBWrite(viPNA, \"SENS1:CORR:CCH:PAR MY_S11\") \nIf (status < VI_SUCCESS) Then HandleVISAError \n' Acquire the S11 confidence check data from ECal Module A \n' into the memory buffer (asking for an OPC reply when it's done). \nstatus = myGPIBWrite(viPNA, \"SENS1:CORR:CCH:ACQ ECAL1;*OPC?\") \nIf (status < VI_SUCCESS) Then HandleVISAError \n' The PNA sends an OPC reply (\"+1\") when the confidence data \n' acquisition into memory is complete, so this Read is waiting on \n' the reply until it is received. \nstatus = myGPIBRead(viPNA, strReply) \nIf (status < VI_SUCCESS) Then HandleVISAError \n' Turn on trace math so the trace shows data divided by memory. \n' You can be confident the S11 calibration is reasonably good if \n1961\n\n' the displayed trace varies no more than a few tenths of a dB \n' from 0 dB across the entire span. \nstatus = myGPIBWrite(viPNA, \"CALC1:PAR:SEL MY_S11\") \nIf (status < VI_SUCCESS) Then HandleVISAError \nstatus = myGPIBWrite(viPNA, \"CALC1:MATH:FUNC DIV\") \nIf (status < VI_SUCCESS) Then HandleVISAError \nEnd Sub \nPrivate Sub cmdQuit_Click() \n' Turn off trace math \nstatus = myGPIBWrite(viPNA, \"CALC1:MATH:FUNC NORM\") \nIf (status < VI_SUCCESS) Then HandleVISAError \n' Conclude the confidence check to set the ECal module \n' back to it's idle state. \nstatus = myGPIBWrite(viPNA, \"SENS1:CORR:CCH:DONE\") \nIf (status < VI_SUCCESS) Then HandleVISAError \n' Close the resource manager session (which also closes \n' the session to the PNA). \nIf defRM <> 0 Then Call viClose(defRM) \n' End the program \nEnd \nEnd Sub \nPrivate Function myGPIBWrite(ByVal viHandle As Long, ByVal strOut As String) As Long \n' The \"+ Chr$(10)\" appends an ASCII linefeed character to the output, for \n' terminating the write transaction. \nmyGPIBWrite = viVPrintf(viHandle, strOut + Chr$(10), 0) \nEnd Function \nPrivate Function myGPIBRead(ByVal viHandle As Long, strIn As String) As Long \nmyGPIBRead = viVScanf(viHandle, \"%t\", strIn) \nEnd Function \nSub HandleVISAError() \nDim strVisaErr As String * 200 \nCall viStatusDesc(defRM, status, strVisaErr) \nMsgBox \"*** Error : \" + strVisaErr, vbExclamation \nEnd \nEnd Sub \n1962\n\nPerform a Source and Receiver Power Cal using SCPI \nProgramming the PNA using COM or using SICL/VISA over LAN (as in this example) leaves the PNA free to \ncontrol GPIB devices as needed. \nThe first example, using Visual Basic, demonstrates the following: \nPerforming a source power calibration of Port 2 for Channel 1. \nReading the calibration data. \nThe second example performs a Receiver Power Cal using VBScript. \nLearn more about Power Calibrations. \nSee an example that Uploads a Source Power Cal. \nOther SCPI Example Programs \nTo run this program, you need: \nOne of the following power meters connected to the PNA through GPIB: E4416A, E4417A, E4418A/B, \nE4419A/B, 437B, 438A, EPM-441A, EPM-442A \nNote: If your power meter is other than these, you can create your own Power Meter Driver using our template. \nYour PC and PNA both connected to a LAN (for communicating with each other). \nThe SICL and VISA components of Agilent�s I/O Libraries software installed on your PC (both are included when \nyou install the software, unless you already have another vendor's VISA installed. Then specify Full SICL and \nVISA installation to overwrite the other vendor's VISA. \nThe module visa32.bas added to your VB project. \nA form with one button labeled cmdRun. \nA VISA interface configured on your remote PC to control the PNA. This could be GPIB interface or a VISA LAN \nClient. \nOn the PNA connect a Thru cable from port 1 to port 2. \nNote: The SOURce:POWer:CORRection:COLLect:ACQuire command, when used with a power meter, cannot be \nsent over the GPIB unless the power meter is connected to a different GPIB interface. See the alternative methods \ndescribed in the command details. \n'Session to VISA Default Resource Manager \nPrivate defRM As Long \n1963\n\n'Session to PNA \nPrivate viPNA As Long \n'VISA function status return code \nPrivate status As Long \nPrivate Sub Form_Load() \ndefRM = 0 \nEnd Sub \nPrivate Sub cmdRun_Click() \n' String to receive data from the PNA. \n' Dimensioned large enough to receive scalar comma-delimited values \n' for 21 frequency points (20 ASCII characters per point) \nDim strReply As String * 420 \nDim strStimulus, strCalValue \nDim strResult As String \n' Open the VISA default resource manager \nstatus = viOpenDefaultRM(defRM) \nIf (status < VI_SUCCESS) Then HandleVISAError \n' Open a session (viPNA) to the PNA at \"address 16\" on the VISA \n' interface configured as \"GPIB1\" on this PC. This could be a \n' VISA LAN Client pointing to the SICL LAN Server on the PNA, or \n' an actual GPIB interface on this PC connected to the PNA GPIB \n' (in which case the power meter would need to be connected to a \n' different GPIB interface on the PNA, such as the Agilent 82357A \n' USB-to-GPIB). \nstatus = viOpen(defRM, \"GPIB0::16::INSTR\", 0, 0, viPNA) \nIf (status < VI_SUCCESS) Then HandleVISAError \n' Set the number of sweep points to 21 on Channel 1. \nstatus = myGPIBWrite(viPNA, \"SENS1:SWE:POIN 21\") \nIf (status < VI_SUCCESS) Then HandleVISAError \n1964\n\n' Specify the GPIB address of the power meter \n' that will be used in performing the calibration. \nstatus = myGPIBWrite(viPNA, \"SYST:COMM:GPIB:PMET:ADDR 13\") \nIf (status < VI_SUCCESS) Then HandleVISAError \n' Turn use of the loss table OFF (this assumes there is \n' virtually no loss in the RF path to the power sensor \n' due to a splitter, coupler or adapter). \nstatus = myGPIBWrite(viPNA, \"SOUR:POW:CORR:COLL:TABL:LOSS OFF\") \nIf (status < VI_SUCCESS) Then HandleVISAError \n' Turn frequency checking OFF (so one power sensor is used for the entire cal \n' acquisition sweep regardless of frequency span). \nstatus = myGPIBWrite(viPNA, \"SOUR:POW:CORR:COLL:FCH OFF\") \nIf (status < VI_SUCCESS) Then HandleVISAError \n' Specify a nominal power accuracy tolerance (NTOLerance) in dB for the \ncalibration, \n' and the maximum number (COUNt) of iterations to adjust power at each point, \n' attempting to achieve within tolerance of the desired power. If at any \nstimulus \n' point the power fails to reach within the set tolerance of the desired power \n' after the maximum number of iterations, the power at that point will be set to \nthe \n' value determined by the last iteration (the Source Power Cal dialog box will \n' indicate the FAIL, but we can still apply the cal if desired when it's \ncomplete). \n' Each iteration is based upon a SETTLED power reading (see comments preceding \nthe \n' next two commands below). \nstatus = myGPIBWrite(viPNA, \"SOUR1:POW2:CORR:COLL:ITER:NTOL 0.1\") \nIf (status < VI_SUCCESS) Then HandleVISAError \nstatus = myGPIBWrite(viPNA, \"SOUR1:POW2:CORR:COLL:ITER:COUN 3\") \nIf (status < VI_SUCCESS) Then HandleVISAError \n' The worst-case window of power uncertainty (for a calibration which meets \n' tolerance) is the sum of the iteration tolerance and the power meter settling \n' tolerance (which is described below). \n1965\n\n' At each stimulus point, the PNA takes power meter readings and determine when \n' they have settled by comparing the magnitude difference between consecutive \n' readings versus a nominal dB tolerance limit (NTOLerance) on that magnitude \n' difference. When consecutive readings are within tolerance of each other, or \n' if they are not within tolerance but we've taken a maximum number of readings \n' (COUNt), the PNA does a weighted average of the readings taken at that stimulus \n' point and that is considered our settled power reading. \nstatus = myGPIBWrite(viPNA, \"SOUR1:POW2:CORR:COLL:AVER:NTOL 0.1\") \nIf (status < VI_SUCCESS) Then HandleVISAError \nstatus = myGPIBWrite(viPNA, \"SOUR1:POW2:CORR:COLL:AVER:COUN 5\") \nIf (status < VI_SUCCESS) Then HandleVISAError \n' Specify if the cal power level is offset (positive value for a gain, negative \n' value for a loss) from the PNA port power setting on the channel when no source \n' power cal is active. This is to account for components between the PNA test \n' port and cal reference plane. In this example, we will calibrate at the PNA \n' test port, so there is no offset (it is zero). \nstatus = myGPIBWrite(viPNA, \"SOUR1:POW2:CORR:OFFS 0 DB\") \nIf (status < VI_SUCCESS) Then HandleVISAError \n' Show the source power cal dialog during the source power cal acquisition. \n' (this is the default, so this command is only necessary if this setting \n' may have been changed beforehand, perhaps by another program). \nstatus = myGPIBWrite(viPNA, \"SOUR1:POW2:CORR:COLL:DISP ON\") \nIf (status < VI_SUCCESS) Then HandleVISAError \n' Specify the method (type of device) that will be used to perform the cal. \n' Choose from power meter (PMETer), power meter and receiver (PMReceiver) \n' or just receiver (RECeiver). \n' PMReceiver uses the power meter for the first iteration of each point and \n' the PNA's reference receiver for subsequent iterations, so is much faster \n' than using power meter only. But the power meter accounts for compression \n' when calibrating at the output of an active device, whereas the reference \n' receiver cannot unless it is coupled to the cal reference plane (on a PNA \n1966\n\n' which allows direct access to the receivers). \n' Perform the source power cal acquisition sweep using the sensor attached to \n' Channel A of the power meter (asking for an OPC reply when it�s done). This \n' assumes that the power sensor is already connected to Port 2 of the PNA. \n' We'll put up an hourglass cursor while waiting for the acquire to complete. \nScreen.MousePointer = vbHourglass \nstatus = myGPIBWrite(viPNA, \"SOUR1:POW2:CORR:COLL:ACQ PMET,'ASEN';*OPC?\") \nIf (status < VI_SUCCESS) Then HandleVISAError \n' Other valid selections would be the following: \n� This mode uses Power Meter and Reference Receiver \n�status = myGPIBWrite(viPNA, \"SOUR1:POW2:CORR:COLL:ACQ PMR,'BSEN';*OPC?\") \n� This mode uses PNA receiver only (no power meter) \n�status = myGPIBWrite(viPNA, \"SOUR1:POW2:CORR:COLL:ACQ REC,'b1';*OPC?\") \n' In the process of beginning a source power cal acquisition, the PNA searches \n' for the power meter on VISA interfaces configured in the Agilent I/O Libraries \n' on the PNA. One of those interfaces is the SICL/VISA LAN server, so if this \n' program is using that interface, we need to ensure our program is not pending \n' an operation on that interface when the PNA wants to search it. So this \n' Wait subroutine suspends execution of our program (for 6000 milliseconds = \n' 6 seconds), giving the PNA time to search that interface and discover that the \n' power meter is not there (the 6 seconds is just to be safe, the search actually \n' takes only a few seconds). \n' Note: If instead of using the VISA LAN server interface, you are having this \n' program communicate with the PNA via it's GPIB interface (which requires the \n' power meter be connected to a different GPIB interface on the PNA, such as the \n' Agilent 82357A USB-to-GPIB), then this Wait is not needed. \nWait 6000 \n' The PNA sends an OPC reply (\"+1\") when the cal acquisition is complete, so \n' our Read operation will wait on the reply until it is received. We need to \n' set the VISA timeout value long enough to give our Read sufficient time to \n' complete before a timeout error occurs. For this example, let's try setting \n' the limit to 60000 milliseconds (60 seconds). \nstatus = viSetAttribute(viPNA, VI_ATTR_TMO_VALUE, 60000) \n1967\n\nIf (status < VI_SUCCESS) Then HandleVISAError \nstatus = myGPIBRead(viPNA, strReply) \nIf (status < VI_SUCCESS) Then HandleVISAError \n' Change mouse cursor from hourglass back to normal \nScreen.MousePointer = vbDefault \n' Conclude the calibration. This applies the cal data to PNA channel memory, \n' and turns the correction ON for Port 2 on Channel 1, \n' but does NOT save the calibration. \nstatus = myGPIBWrite(viPNA, \"SOUR1:POW2:CORR:COLL:SAVE\") \nIf (status < VI_SUCCESS) Then HandleVISAError \n' At this point, if you choose to save the instrument state as a \".CST\" file, \n' the calibration will be saved with the instrument state in that file. \n' Prepare for doing data transfer in ASCII format. \nstatus = myGPIBWrite(viPNA, \"FORM:DATA ASCII\") \nIf (status < VI_SUCCESS) Then HandleVISAError \n' Read the stimulus values from Channel 1. \nstatus = myGPIBWrite(viPNA, \"SENS1:X?\") \nIf (status < VI_SUCCESS) Then HandleVISAError \nstatus = myGPIBRead(viPNA, strReply) \nIf (status < VI_SUCCESS) Then HandleVISAError \n' Tokenize the reply string into an array containing the values \nstrStimulus = Split(strReply, \",\") \n' Read the source power correction data. \nstatus = myGPIBWrite(viPNA, \"SOUR1:POW2:CORR:DATA?\") \nIf (status < VI_SUCCESS) Then HandleVISAError \nstatus = myGPIBRead(viPNA, strReply) \nIf (status < VI_SUCCESS) Then HandleVISAError \n' Tokenize the reply string into an array containing the values \n1968\n\nstrCalValue = Split(strReply, \",\") \n' Print the data using a message box (here, Chr returns the ASCII characters \n' for Tab (9) and Linefeed (10)). \nstrResult = \"Stimulus\" & Chr(9) & Chr(9) & \"Cal Value\" & Chr(10) \nFor i = 0 To UBound(strStimulus) \nstrResult = strResult & Val(strStimulus(i)) & Chr(9) & Val(strCalValue(i)) & \nChr(10) \nNext \nMsgBox strResult \nEnd Sub \nPrivate Function myGPIBWrite(ByVal viHandle As Long, ByVal strOut As String) As \nLong \n' The \"+ Chr$(10)\" appends an ASCII linefeed character to the \n' output, for terminating the write transaction. \nmyGPIBWrite = viVPrintf(viHandle, strOut + Chr$(10), 0) \nEnd Function \nPrivate Function myGPIBRead(ByVal viHandle As Long, strIn As String) As Long \nmyGPIBRead = viVScanf(viHandle, \"%t\", strIn) \nEnd Function \nSub HandleVISAError() \nDim strVisaErr As String * 200 \nCall viStatusDesc(defRM, status, strVisaErr) \nMsgBox \"*** Error : \" + strVisaErr, vbExclamation \n' Close the resource manager session (which also closes \n' the session to the PNA). \nIf defRM <> 0 Then Call viClose(defRM) \nEnd \nEnd Sub \nPublic Sub Wait(ByVal mS_delay As Long) \n1969\n\nDim t0 As Single \nt0 = Timer \nDo While Timer - t0 < mS_delay / 1000 \nDim dummy As Integer \ndummy = DoEvents() ' if we cross midnight, back up one day \nIf Timer < t0 Then t0 = t0 - 86400 \nLoop \nEnd Sub \nPerform a Receiver Power Cal \nThe SCPI commands in this example are sent over a COM interface using the SCPIStringParser object. You do \nNOT need a GPIB connection to run this example. \nThis VBScript (*.vbs) program can be run as a macro in the PNA. To do this, copy the following code into a text \neditor file, such as Notepad, and save it on the PNA hard drive as *.vbs. \nLearn how to setup and run the macro. \nDim pna \nDim scpi \nSet pna = CreateObject(\"AgilentPNA835x.Application\") \nSet scpi = pna.ScpiStringParser \n' For simplicity, this example starts from the preset instrument state \nscpi.Execute \"SYST:PRESet\" \n' Turn off continuous sweep \nscpi.Execute \"INITiate:CONTinuous OFF\" \n' Select the S11 measurement that was created by the instrument preset \nscpi.Execute \"CALCulate:PARameter:SELect 'CH1_S11_1'\" \n' Change the measurement parameter to measure the B receiver \nscpi.Execute \"CALCulate:PARameter:MODify B,1\" \n' Specify the Calibration Type, then Prompt \n' to ensure the receiver is connected to port 1. \nscpi.Execute \"SENSe:CORRection:COLLect:METHod RPOWer\" \nMsgBox \"Connect port 1 to port 2 so power is supplied to the B receiver, then press \nenter\" \n' Acquire the power measurement; returning reply to *OPC? when finished. \nresponse = scpi.Execute( \"SENSe:CORRection:COLLect:ACQuire POWer;*OPC?\" ) \n' Compute the error term, store to calset and turn on the calibration. \nresponse = scpi.Execute( \"SENSe:CORRection:COLLect:SAVE\" ) \nMsgBox \"Done with calibration.\" \nLast modified: \n9/22/06 Modified for receiver only feature \n1970\n\n1971\n\nUploading a Source Power Cal using SCPI \nProgramming the PNA using COM or using SICL/VISA over LAN (as in this example) leaves the PNA free to \ncontrol GPIB devices as needed. This Visual Basic program demonstrates: \nUploading a source power calibration of Port 2 for Channel 1. \nReading the calibration data. \nLearn more about Power Calibrations \nOther SCPI Example Programs \nTo run this program, you need: \nYour PC and PNA both connected to a LAN (if using VISA LAN server / client). \nThe SICL and VISA components of Agilent�s I/O Libraries software installed on your PC (both are included when \nyou install the software, unless you already have another vendor's VISA installed. Then specify Full SICL and \nVISA installation to overwrite the other vendor's VISA. \nThe module visa32.bas added to your VB project. \nA form with two buttons: cmdRun and cmdQuit. \nA VISA interface configured on your remote PC to control the PNA. This could be GPIB interface or a VISA LAN \nClient. \n'Session to VISA Default Resource Manager \nPrivate defRM As Long \n'Session to PNA \nPrivate viPNA As Long \n'VISA function status return code \nPrivate status As Long \nPrivate Sub Form_Load() \ndefRM = 0 \nEnd Sub \nPrivate Sub cmdRun_Click() \n' String to receive data from the PNA. \n' Dimensioned large enough to receive scalar comma-delimited values \n' for 21 frequency points (20 ASCII characters per point) \nDim strReply As String * 420 \nDim strPower As String, strCalPower As String \nDim strStimulus, strCalValue \nDim strResult As String \n' Open the VISA default resource manager \n1972\n\nstatus = viOpenDefaultRM(defRM) \nIf (status < VI_SUCCESS) Then HandleVISAError \n' Open a session (viPNA) to the PNA at \"address 16\" on the VISA \n' interface configured as \"GPIB0\" on this PC. \nstatus = viOpen(defRM, \"GPIB0::16::INSTR\", 0, 0, viPNA) \nIf (status < VI_SUCCESS) Then HandleVISAError \n' Set the number of sweep points to 2 on Channel 1. \nstatus = myGPIBWrite(viPNA, \"SENS1:SWE:POIN 2\") \nIf (status < VI_SUCCESS) Then HandleVISAError \n' Ensure there's currently no source power cal on for this channel and port. \nstatus = myGPIBWrite(viPNA, \"SOUR1:POW2:CORR OFF\") \nIf (status < VI_SUCCESS) Then HandleVISAError \n' Specify if the cal power level is offset (positive value for a gain, negative \n' value for a loss) from the PNA port power setting on the channel when no source \n' power cal is active. This is to account for components between the PNA test \n' port and cal reference plane. In this example, let's set up our calibration \n' at the output of an amplifier with 15 dB gain. \nstatus = myGPIBWrite(viPNA, \"SOUR1:POW2:CORR:OFFS 15 DB\") \nIf (status < VI_SUCCESS) Then HandleVISAError \n' Prepare for doing data transfer in ASCII format. \nstatus = myGPIBWrite(viPNA, \"FORM:DATA ASCII\") \nIf (status < VI_SUCCESS) Then HandleVISAError \n' Send our source power correction data to the PNA. For purpose of simplicity \n' in this example, we'll set up for no correction (0) at our start stimulus and \n' 0.5 dB at our stop stimulus (recall that our sweep currently has just 2 points). \nstatus = myGPIBWrite(viPNA, \"SOUR1:POW2:CORR:DATA 0,0.5\") \nIf (status < VI_SUCCESS) Then HandleVISAError \n' Set the number of sweep points to 21 on Channel 1. \nstatus = myGPIBWrite(viPNA, \"SENS1:SWE:POIN 21\") \nIf (status < VI_SUCCESS) Then HandleVISAError \n' Read the fixed power level for this port on Channel 1. \nstatus = myGPIBWrite(viPNA, \"SOUR1:POW2:LEV?\") \nIf (status < VI_SUCCESS) Then HandleVISAError \nstatus = myGPIBRead(viPNA, strReply) \nIf (status < VI_SUCCESS) Then HandleVISAError \nstrPower = strReply \n' Turn the source power cal on. \nstatus = myGPIBWrite(viPNA, \"SOUR1:POW2:CORR ON\") \nIf (status < VI_SUCCESS) Then HandleVISAError \n' Again read the fixed power level for this port on Channel 1 \n' (with our calibration turned on, this should now include the 15 dB offset \n' we indicated our power amplifier provides). \n1973\n\nstatus = myGPIBWrite(viPNA, \"SOUR1:POW2:LEV?\") \nIf (status < VI_SUCCESS) Then HandleVISAError \nstatus = myGPIBRead(viPNA, strReply) \nIf (status < VI_SUCCESS) Then HandleVISAError \nstrCalPower = strReply \n' Read the stimulus values from Channel 1. \nstatus = myGPIBWrite(viPNA, \"SENS1:X?\") \nIf (status < VI_SUCCESS) Then HandleVISAError \nstatus = myGPIBRead(viPNA, strReply) \nIf (status < VI_SUCCESS) Then HandleVISAError \n' Tokenize the reply string into an array containing the values \nstrStimulus = Split(strReply, \",\") \n' Read back the source power correction data, now interpolated for 21 points \nstatus = myGPIBWrite(viPNA, \"SOUR1:POW2:CORR:DATA?\") \nIf (status < VI_SUCCESS) Then HandleVISAError \nstatus = myGPIBRead(viPNA, strReply) \nIf (status < VI_SUCCESS) Then HandleVISAError \n' Tokenize the reply string into an array containing the values \nstrCalValue = Split(strReply, \",\") \n' Print the data using a message box (here, Chr returns the ASCII characters \n' for Tab (9) and Linefeed (10)). \nstrResult = \"PNA port power = \" & Val(strPower) & Chr(10) \nstrResult = strResult & \"Power at reference plane = \" & Val(strCalPower) & Chr(10) \nChr(10) \nstrResult = strResult & \"Stimulus\" & Chr(9) & Chr(9) & \"Cal Value\" & Chr(10) \nFor i = 0 To UBound(strStimulus) \nstrResult = strResult & Val(strStimulus(i)) & Chr(9) & Val(strCalValue(i)) & \nChr(10) \nNext \nMsgBox strResult \nEnd Sub \nPrivate Sub cmdQuit_Click() \n' Close the resource manager session (which also closes \n' the session to the PNA). \nIf defRM <> 0 Then Call viClose(defRM) \n' End the program \nEnd \nEnd Sub \nPrivate Function myGPIBWrite(ByVal viHandle As Long, ByVal strOut As String) As Long \n' The \"+ Chr$(10)\" appends an ASCII linefeed character to the \n' output, for terminating the write transaction. \nmyGPIBWrite = viVPrintf(viHandle, strOut + Chr$(10), 0) \nEnd Function \nPrivate Function myGPIBRead(ByVal viHandle As Long, strIn As String) As Long \n1974\n\nmyGPIBRead = viVScanf(viHandle, \"%t\", strIn) \n' Remove trailing linefeed character \nIf Right(strIn, 1) = Chr(10) Then strIn = Left(strIn, Len(strIn) - 1) \nEnd Function \nSub HandleVISAError() \nDim strVisaErr As String * 200 \nCall viStatusDesc(defRM, status, strVisaErr) \nMsgBox \"*** Error : \" + strVisaErr, vbExclamation \n' Close the resource manager session (which also closes \n' the session to the PNA). \nIf defRM <> 0 Then Call viClose(defRM) \nEnd \nEnd Sub \n1975\n\nPerform a Sliding Load Calibration using GPIB \nThis Visual Basic program does a only the sliding load portion of a Calibration. \nTo run this program, you need: \nAn established GPIB interface connection \nA measurement and calibration routine to call this sub-program \nSTAN3 set up as a sliding load standard \nSee Other SCPI Example Programs \nSub slide() \n'Measure the sliding load for at least 5 and no more than 7 slides \n'Note that \"SLSET\" and \"SLDONE\" must be executed before the actual acquisition of a \nslide \nMsgBox \"Connect Sliding Load; set to Position 1; then press OK\" \nGPIB.Write \"SENS:CORR:COLL SLSET\" \nGPIB.Write \"SENS:CORR:COLL STAN3;\" \nMsgBox \"Set Sliding Load to position 2; then press OK\" \nGPIB.Write \"SENS:CORR:COLL SLSET\" \nGPIB.Write \"SENS:CORR:COLL STAN3;\" \nMsgBox \"Set Sliding Load to position 3; then press OK\" \nGPIB.Write \"SENS:CORR:COLL SLDONE\" \nGPIB.Write \"SENS:CORR:COLL STAN3;\" \nEnd Sub \n1976\n\nLoad Error Terms during a Cal Sequence \nThis example requires that you already have a Cal Set named \"foo\" that contains a 1-port cal on port 1 and a 1-port \ncal on port 2. \nThis example starts a Guided Calibration specifying an Unknown Thru. It loads the 1-port Cals from the existing \n\"foo\" Cal Set, then recalculates the number of steps required to complete the cal. After loading the 1-port cals, only \nthe Unknown Thru standard is left to acquire. \nSENS:CORR:COLL:GUID:CONN:PORT1 \"APC 3.5 female\" \nSENS:CORR:COLL:GUID:CONN:PORT2 \"APC 3.5 female\" \nSENS:CORR:COLL:GUID:CKIT:PORT1 \"85033D/E\" \nSENS:CORR:COLL:GUID:CKIT:PORT2 \"85033D/E\" \nSENS:CORR:COLL:GUID:METH UNKN \n' auto-create user calsets for SCPI \nSENS:CORR:PREF:CSET:SAVU 1 \nSENS:CORR:COLL:GUID:INIT \n' should return the number 7 \nSENS:CORR:COLL:GUID:STEPS? \n' to port 1, from port 1 in calset \nSENS:CORR:COLL:GUID:ETER:LOAD \"foo\",1,1 \n' to port 2, from port 2 in calset \nSENS:CORR:COLL:GUID:ETER:LOAD \"foo\",2,2 \n' should now return the number 1 \nSENS:CORR:COLL:GUID:STEPS? \n' measure the unknown thru \nSENS:CORR:COLL:GUID:ACQ STAN1 \n' save the cal to new user calset \nSENS:CORR:COLL:GUID:SAVE \n1977\n\nCreate New Cal Kit using SCPI \nWhen creating new cal kits programmatically, the order in which cal kit commands are sent can be important. \nFor example to create a kit with opens, shorts, loads, and thrus. Be sure to use the following sequence for each \nnewly defined standard. \nProgrammatically select the standard number 1. \nProgrammatically select the standard type. 2. \nProgram the cal standard's values. 3. \nRepeat steps 1, 2, 3 for additional new standards being defined. 4. \n10 ! \n20 ! \n30 ! This example program demonstrates how to create \n40 ! new PNA calibration kits. \n50 ! \n60 ! 1) Select a kit not previously defined \n70 ! 2) Define open, short, load, and thru cal standards \n80 ! Note: Each of the newly defined standards is assigned \n90 ! a default connector name. These default connector names \n100 ! will be replaced in subsequent steps. \n110 ! 3) Use the delete connector command to remove default \n120 ! connector names. \n130 ! 4) Add connectors. Specify: \n140 ! Start and Stop Freq \n150 ! Z - Impedance \n160 ! sex - MALE, FEMALE, NONE \n170 ! media - COAX, WAVE \n180 ! cutoff - Frequency for waveguide \n190 ! 5) Assign the appropriate connector to each standard \n200 ! 6) Modify the class assignments for the standards defined \n210 ! 7) Verify the kit values \n220 ! \n230 ! Additional Note: After setting each new cal kit value, it is \n240 ! recommended that the program periodically perform queries to \n250 ! verify the new values. \n260 ! \n270 ! This will prevent program synchronization issues that can affect \n280 ! final values stored within new cal kits. \n290 ! \n300 !------------------------------------------------------------ \n310 ! \n320 ! Set up I/O path \n330 ASSIGN @Na TO 716 \n340 DIM Calkname$[80],Conn$[80] \n350 INTEGER Calkitnum \n1978\n\n360 ! \n370 CLEAR SCREEN \n380 ! \n390 !!!!!!!!!!!!!!!!!!!!!!!!!!!!!!!!!!!!!!!!!!!!!!!!!!!!!!! \n400 ! Designate the kit selection to be used for performing cal's \n410 OUTPUT @Na;\":sens:corr:ckit:count?\" \n420 ENTER @Na;Calkitnum \n430 Calkitnum=Calkitnum+1 \n440 OUTPUT @Na;\":sens:corr:coll:ckit \"&VAL$(Calkitnum) \n450 ! \n460 ! Name this kit with your own name \n470 OUTPUT @Na;\":sens:corr:coll:ckit:name \"\"Special 2.4 mm Model 85056\"\"\" \n480 ! \n490 ! \n500 DISP \"Defining kit std 1...\" \n510 ! Now set up standard #1 \n520 OUTPUT @Na;\":sens:corr:coll:ckit:stan 1\" \n530 OUTPUT @Na;\":sens:corr:coll:ckit:stan:type SHORT\" \n540 Get_std \n550 OUTPUT @Na;\":sens:corr:coll:ckit:stan:char coax\" \n560 OUTPUT @Na;\":sens:corr:coll:ckit:stan:label \"\"My Short\"\"\" \n570 Get_label \n580 ! \n590 DISP \"Defining kit std 2...\" \n600 ! Now set up standard #2 \n610 OUTPUT @Na;\":sens:corr:coll:ckit:stan 2\" \n620 OUTPUT @Na;\":sens:corr:coll:ckit:stan:type OPEN\" \n630 Get_std \n640 OUTPUT @Na;\":sens:corr:coll:ckit:stan:char coax\" \n650 OUTPUT @Na;\":sens:corr:coll:ckit:stan:label \"\"My Open\"\"\" \n660 Get_label \n670 ! \n680 DISP \"Defining kit std 3...\" \n690 ! Now set up standard #3 \n700 OUTPUT @Na;\":sens:corr:coll:ckit:stan 3\" \n710 OUTPUT @Na;\":sens:corr:coll:ckit:stan:type LOAD\" \n720 Get_std \n730 OUTPUT @Na;\":sens:corr:coll:ckit:stan:char coax\" \n740 OUTPUT @Na;\":sens:corr:coll:ckit:stan:label \"\"My Fixed Load\"\"\" \n750 Get_label \n760 ! \n770 DISP \"Defining kit std 4...\" \n780 ! Now set up standard #4 \n790 OUTPUT @Na;\":sens:corr:coll:ckit:stan 4\" \n800 OUTPUT @Na;\":sens:corr:coll:ckit:stan:type THRU\" \n810 Get_std \n820 OUTPUT @Na;\":sens:corr:coll:ckit:stan:char coax\" \n830 OUTPUT @Na;\":sens:corr:coll:ckit:stan:label \"\"My Thru\"\"\" \n840 Get_label \n1979\n\n850 ! \n860 DISP \"Defining kit std 5...\" \n870 ! Now set up standard #5 \n880 OUTPUT @Na;\":sens:corr:coll:ckit:stan 5\" \n890 OUTPUT @Na;\":sens:corr:coll:ckit:stan:type SLOAD\" \n900 Get_std \n910 OUTPUT @Na;\":sens:corr:coll:ckit:stan:char coax\" \n920 OUTPUT @Na;\":sens:corr:coll:ckit:stan:label \"\"Sliding Load\"\"\" \n930 Get_label \n940 ! \n950 DISP \"Defining kit std 6...\" \n960 ! Now set up standard #6 \n970 ! \n980 OUTPUT @Na;\":sens:corr:coll:ckit:stan 6\" \n990 OUTPUT @Na;\":sens:corr:coll:ckit:stan:type SHORT\" \n1000 Get_std \n1010 OUTPUT @Na;\":sens:corr:coll:ckit:stan:char coax\" \n1020 OUTPUT @Na;\":sens:corr:coll:ckit:stan:label \"\"Short\"\"\" \n1030 Get_label \n1040 ! \n1050 DISP \"Defining kit std 7...\" \n1060 ! Now set up standard #7 \n1070 OUTPUT @Na;\":sens:corr:coll:ckit:stan 7\" \n1080 OUTPUT @Na;\":sens:corr:coll:ckit:stan:type SHORT\" \n1090 Get_std \n1100 OUTPUT @Na;\":sens:corr:coll:ckit:stan:char coax\" \n1110 OUTPUT @Na;\":sens:corr:coll:ckit:stan:label \"\"Short\"\"\" \n1120 Get_label \n1130 ! \n1140 DISP \"Defining kit std 8...\" \n1150 ! Now set up standard #8 \n1160 ! \n1170 OUTPUT @Na;\":sens:corr:coll:ckit:stan 8\" \n1190 OUTPUT @Na;\":sens:corr:coll:ckit:stan:type ARBI\" \n1200 Get_std \n1210 OUTPUT @Na;\":sens:corr:coll:ckit:stan:char coax\" \n1220 OUTPUT @Na;\":sens:corr:coll:ckit:stan:TZR 15;\" \n1230 OUTPUT @Na;\":sens:corr:coll:ckit:stan:TZI -9;\" \n1240 OUTPUT @Na;\":sens:corr:coll:ckit:stan:label \"\"Z Load\"\"\" \n1250 Get_label \n1260 ! \n1270 ! \n1280 ! \n1290 ! First remove any old connector names \n1300 OUTPUT @Na;\":sens:corr:coll:ckit:conn:del\" \n1310 ! Verify that no connectors are currently installed \n1320 OUTPUT @Na;\":sens:corr:coll:ckit:conn:cat?\" \n1330 ENTER @Na;Conn$ \n1340 PRINT \"Verify empty list: \";Conn$ \n1980\n\n1350 ! \n1360 ! Define your new connectors \n1370 OUTPUT @Na;\":sens:corr:coll:ckit:conn:add \"\"PSC \n2.4\"\",0HZ,999GHZ,50.0,MALE,COAX,0.0\" \n1380 OUTPUT @Na;\":sens:corr:coll:ckit:conn:add \"\"PSC \n2.4\"\",0HZ,999GHZ,50.0,FEMALE,COAX,0.0\" \n1390 ! \n1400 ! Verify that the new connectors are installed \n1410 OUTPUT @Na;\":sens:corr:coll:ckit:conn:cat?\" \n1420 ENTER @Na;Conn$ \n1430 PRINT \"Verify new connectors: \";Conn$ \n1440 DISP \"\" \n1450 ! \n1460 DISP \"Defining conn std 1...\" \n1470 ! Now set up standard #1 \n1480 OUTPUT @Na;\":sens:corr:coll:ckit:stan 1\" \n1490 Verify_std \n1500 OUTPUT @Na;\":sens:corr:coll:ckit:conn:snam \"\"PSC 2.4\"\",FEMALE,1\" \n1510 Print_connector \n1520 ! \n1530 DISP \"Defining conn std 2...\" \n1540 ! Now set up standard #2 \n1550 OUTPUT @Na;\":sens:corr:coll:ckit:stan 2\" \n1560 Verify_std \n1570 OUTPUT @Na;\":sens:corr:coll:ckit:conn:snam \"\"PSC 2.4\"\",FEMALE,1\" \n1580 Print_connector \n1590 ! \n1600 DISP \"Defining conn std 3...\" \n1610 ! Now set up standard #3 \n1620 OUTPUT @Na;\":sens:corr:coll:ckit:stan 3\" \n1630 Verify_std \n1640 OUTPUT @Na;\":sens:corr:coll:ckit:conn:snam \"\"PSC 2.4\"\",FEMALE,1\" \n1650 Print_connector \n1660 ! \n1670 DISP \"Defining conn std 4...\" \n1680 ! Now set up standard #4 \n1690 OUTPUT @Na;\":sens:corr:coll:ckit:stan 4\" \n1700 Verify_std \n1710 OUTPUT @Na;\":sens:corr:coll:ckit:conn:snam \"\"PSC 2.4\"\",FEMALE,1\" \n1720 OUTPUT @Na;\":sens:corr:coll:ckit:conn:snam \"\"PSC 2.4\"\",MALE,2\" \n1730 Print_connector \n1740 ! \n1750 DISP \"Defining conn std 5...\" \n1760 ! Now set up standard #5 \n1770 OUTPUT @Na;\":sens:corr:coll:ckit:stan 5\" \n1780 OUTPUT @Na;\":sens:corr:coll:ckit:stan:label \"\"Sliding Load\"\"\" \n1790 Verify_std \n1800 OUTPUT @Na;\":sens:corr:coll:ckit:conn:snam \"\"PSC 2.4\"\",MALE,1\" \n1810 Print_connector \n1981\n\n1820 ! \n1830 DISP \"Defining conn std 6...\" \n1840 ! Now set up standard #6 \n1850 ! \n1860 OUTPUT @Na;\":sens:corr:coll:ckit:stan 6\" \n1870 Verify_std \n1880 OUTPUT @Na;\":sens:corr:coll:ckit:conn:snam \"\"PSC 2.4\"\",MALE,1\" \n1890 Print_connector \n1900 ! \n1910 DISP \"Defining conn std 7...\" \n1920 ! Now set up standard #7 \n1930 OUTPUT @Na;\":sens:corr:coll:ckit:stan 7\" \n1940 Verify_std \n1950 OUTPUT @Na;\":sens:corr:coll:ckit:conn:snam \"\"PSC 2.4\"\",MALE,1\" \n1960 Print_connector \n1970 ! \n1980 DISP \"Defining conn std 8...\" \n1990 ! Now set up standard #8 \n2000 OUTPUT @Na;\":sens:corr:coll:ckit:stan 8\" \n2010 Verify_std \n2020 OUTPUT @Na;\":sens:corr:coll:ckit:conn:snam \"\"PSC 2.4\"\",MALE,1\" \n2030 Print_connector \n2040 ! \n2050 DISP \"Class assignments...\" \n2060 ! \n2070 ! Designate the \"order\" associated with measuring the standards \n2080 ! \n2090 ! Set Port 1, 1st standard measured to be standard #2 \n2100 OUTPUT @Na;\":sens:corr:coll:ckit:order1 2\" \n2110 ! Set Port 1, 2nd standard measured to be standard #1 \n2120 OUTPUT @Na;\":sens:corr:coll:ckit:order2 1,6,7\" \n2130 ! Set Port 1, 3nd standard measured to be standard #3 and #5 \n2140 OUTPUT @Na;\":sens:corr:coll:ckit:order3 3,5\" \n2150 ! Set Port 1, 4th standard measured to be standard #4 \n2160 OUTPUT @Na;\":sens:corr:coll:ckit:order4 4\" \n2170 ! \n2180 ! Set Port 2, 1st standard measured to be standard #2 \n2190 OUTPUT @Na;\":sens:corr:coll:ckit:order5 2\" \n2200 ! Set Port 2, 2nd standard measured to be standard #1 \n2210 OUTPUT @Na;\":sens:corr:coll:ckit:order6 1,6,7\" \n2220 ! Set Port 2, 3nd standard measured to be standard #3 and #6 \n2230 OUTPUT @Na;\":sens:corr:coll:ckit:order7 3,5\" \n2240 ! Set Port 2, 4th standard measured to be standard #4 \n2250 OUTPUT @Na;\":sens:corr:coll:ckit:order8 4\" \n2260 ! \n2270 ! Set Port 1, 1st standard \n2280 OUTPUT @Na;\":sens:corr:coll:ckit:olabel1 \"\"MyOpen1\"\"\" \n2290 ! Set Port 1, 2nd standard \n2300 OUTPUT @Na;\":sens:corr:coll:ckit:olabel2 \"\"MyShorts1\"\"\" \n1982\n\n2310 ! Set Port 1, 3nd standard \n2320 OUTPUT @Na;\":sens:corr:coll:ckit:olabel3 \"\"MyLoads1\"\"\" \n2330 ! Set Port 1, 4th standard measured to be standard #4 \n2340 OUTPUT @Na;\":sens:corr:coll:ckit:olabel4 \"\"MyThru1\"\"\" \n2350 ! \n2360 ! Set Port 2, 1st standard \n2370 OUTPUT @Na;\":sens:corr:coll:ckit:olabel5 \"\"MyOpen2\"\"\" \n2380 ! Set Port 2, 2nd standard \n2390 OUTPUT @Na;\":sens:corr:coll:ckit:olabel6 \"\"MyShorts2\"\"\" \n2400 ! Set Port 2, 3nd standard \n2410 OUTPUT @Na;\":sens:corr:coll:ckit:olabel7 \"\"MyLoads2\"\"\" \n2420 ! Set Port 2, 4th standard \n2430 OUTPUT @Na;\":sens:corr:coll:ckit:olabel8 \"\"MyThrus2\"\"\" \n2440 ! \n2450 BEEP \n2460 DISP \"Done!\" \n2470 END \n2480 SUB Get_label \n2490 OUTPUT 716;\":sens:corr:coll:ckit:stan:label?\" \n2500 ENTER 716;Label$ \n2510 PRINT Label$ \n2520 SUBEND \n2530 ! \n2540 SUB Get_std \n2550 OUTPUT 716;\":sens:corr:coll:ckit:stan:type?\" \n2560 ENTER 716;Type$ \n2570 PRINT Type$ \n2580 SUBEND \n2590 ! \n2600 SUB Print_connector \n2610 DIM Nam$[40] \n2620 OUTPUT 716;\":sens:corr:coll:ckit:conn:sname?\" \n2630 ENTER 716;Nam$ \n2640 PRINT Nam$ \n2650 SUBEND \n2660 ! \n2670 SUB Verify_std \n2680 OUTPUT 716;\":sens:corr:coll:ckit:stan:label?\" \n2690 ENTER 716;Label$ \n2700 SUBEND \n2710 ! \n1983\n\nModify a Calibration Kit using SCPI \nThis Visual Basic program: \nModifies Calibration kit number 3 \nCompletely defines standard #4 (thru) \nTo run this program, you need: \nAn established GPIB interface connection \nSee Other SCPI Example Programs \n'Modifying cal kit number 3 \nCalkitnum = 3 \n'Designate the kit selection to be used for performing cal's \nGPIB.Write \"SENSe:CORRection:COLLect:CKIT:SELect \" & Val(Calkitnum) \n'Reset to factory default values. \nGPIB.Write \"SENSe:CORRection:COLLect:CKIT:RESet \" & Val(Calkitnum) \n'Name this kit with your own name \nGPIB.Write \"SENSe:CORRection:COLLect:CKIT:NAME 'My Cal Kit'\" \n'Assign standard numbers to calibration classes \n'Set Port 1, class 1 (S11A) to be standard #8 \nGPIB.Write \"SENSe:CORRection:COLLect:CKIT:ORDer1 8\" \n'Set Port 1, class 2 (S11B) to be standard #7 \nGPIB.Write \"SENSe:CORRection:COLLect:CKIT:ORDer2 7\" \n'Set Port 1, class 3 (S11C) to be standard #3 \nGPIB.Write \"SENSe:CORRection:COLLect:CKIT:ORDer3 3\" \n'Set Port 1, class 4 (S21T) to be standard #4 \nGPIB.Write \"SENSe:CORRection:COLLect:CKIT:ORDer4 4\" \n'Set Port 2, class 1 (S22A) to be standard #8 \nGPIB.Write \"SENSe:CORRection:COLLect:CKIT:ORDer5 8\" \n'Set Port 2, class 2 (S22B) to be standard #7 \nGPIB.Write \"SENSe:CORRection:COLLect:CKIT:ORDer6 7\" \n'Set Port 2, class 3 (S22C) to be standard #3 \nGPIB.Write \"SENSe:CORRection:COLLect:CKIT:ORDer7 3\" \n'Set Port 2, class 4 (S12T) to be standard #4 \nGPIB.Write \"SENSe:CORRection:COLLect:CKIT:ORDer8 4\" \n'Set up Standard #4 completely \n'Select Standard #4; the rest of the commands act on it \nGPIB.Write \"SENSe:CORRection:COLLect:CKIT:STANdard 4\" \nGPIB.Write \"SENSe:CORRection:COLLect:CKIT:STANdard:FMIN 300KHz\" \nGPIB.Write \"SENSe:CORRection:COLLect:CKIT:STANdard:FMAX 9GHz\" \nGPIB.Write \"SENSe:CORRection:COLLect:CKIT:STANdard:IMPedance 50\" \nGPIB.Write \"SENSe:CORRection:COLLect:CKIT:STANdard:DELay 1.234 ns\" \n1984\n\nGPIB.Write \"SENSe:CORRection:COLLect:CKIT:STANdard:LOSS 23e6\" \nGPIB.Write \"SENSe:CORRection:COLLect:CKIT:STANdard:C0 0\" \nGPIB.Write \"SENSe:CORRection:COLLect:CKIT:STANdard:C1 1\" \nGPIB.Write \"SENSe:CORRection:COLLect:CKIT:STANdard:C2 2\" \nGPIB.Write \"SENSe:CORRection:COLLect:CKIT:STANdard:C3 3\" \nGPIB.Write \"SENSe:CORRection:COLLect:CKIT:STANdard:L0 10\" \nGPIB.Write \"SENSe:CORRection:COLLect:CKIT:STANdard:L1 11\" \nGPIB.Write \"SENSe:CORRection:COLLect:CKIT:STANdard:L2 12\" \nGPIB.Write \"SENSe:CORRection:COLLect:CKIT:STANdard:L3 13\" \nGPIB.Write \"SENSe:CORRection:COLLect:CKIT:STANdard:LABel 'My Special Thru'\" \nGPIB.Write \"SENSe:CORRection:COLLect:CKIT:STANdard:TYPE THRU\" \nGPIB.Write \"SENSe:CORRection:COLLect:CKIT:STANdard:CHARacteristic Coax\" \n1985\n\nCreate and Calibrate a VMC Measurement \nThis VB Script example creates and calibrates a Vector mixer measurement. To run this example without \nmodification you need the following: \nA Mixer setup file saved on the PNA: C:\\Program Files\\Agilent\\Network \nAnalyzer\\Documents\\Mixer\\MyMixer.mxr. \nIf the mixer file uses an external LO source, it must also be attached and configured. \nAn ECal module that covers the frequency range of the measurement. \nThe SCPI commands in this example are sent over a COM interface using the SCPIStringParser object. You do \nNOT need a GPIB connection to run this example. However, some modification is necessary to make the program \nrun on a traditional GPIB Interface. \nThis VBScript (*.vbs) program can be run as a macro in the PNA. To do this, copy the following code into a text \neditor file such as Notepad and save it on the PNA hard drive as VMC.vbs. Learn how to setup and run the macro. \nDim app \nDim scpi \n' Create / Get the PNA application. \nSet app = CreateObject(\"AgilentPNA835x.Application\") \nSet scpi = app.ScpiStringParser \n'---Create a Vector Mixer Measurement \n'First, delete all measurements on the channel \nscpi.Execute \"CALC:PAR:DEL:ALL\" \n'Create a forward scalar mixer measurement and configure \n'it in channel 1. \n'The first parameter is a unique identifying string \n'(specified by the user) to allow subsequent \n'commands to be directed at this specific measurement. \nSCPI.Execute \"CALC:CUST:DEF 'My VC21', 'Vector Mixer/Converter', 'VC21'\" \n'Setup the new measurement as the 2nd trace in the active window \nSCPI.Execute \"DISP:WIND:TRAC2:FEED 'My VC21'\" \n'Make the new trace the active measurement \nSCPI.Execute \"CALC:PAR:SEL 'My VC21'\" \n'The parameters of the mixer measurement can now be configured. \n'This can be done by either using the SENS:MIX commands \n'for each of the parameters or by loading a mixer setup file. \n'This example loads a mixer setup file. The path name \n'for the mixer file may be loaded from other mapped drives. \nSCPI.Execute \"SENS:MIXer:Load 'C:\\Program Files\\Agilent\\Network \nAnalyzer\\Documents\\Mixer\\MyMixer.mxr'\" \n'--------------Perform A Vector Mixer Calibration------------- \n'Initialize an VMC guided calibration for session number 6 \nSCPI.Execute \"SENS:CORR:COLL:SESS6:INIT \"\"VMC\"\"\" \n'This sets the VMC operation to full system cal as opposed to \n'performing a mixer characterization only. \n1986\n\nSCPI.Execute \"SENS:CORR:COLL:SESS6:VMC:OPER \"\"CAL\"\"\" \n'This example uses ECal for the 2-port cal portion of the procedure \n'To use a mechanical kit you will have to use the following command: \n'SCPI.Execute \"SENS:CORR:COLL:SESS6:SMC:TWOPort:OPTion\"\"MECH\"\"\" \nSCPI.Execute \"SENS:CORR:COLL:SESS6:VMC:TWOPort:OPTion \"\"ECAL\"\"\" \n'If you select the mechanical method then you also have to \n'specify the connector types and the cal kits for each of the ports. \n'The comments below show an example of how that is done: \n'SCPI.Execute \"SENS:CORR:COLL:SESS6:CONN:PORT1:SEL \"\"APC 3.5 male\"\"\" \n'SCPI.Execute \"SENS:CORR:COLL:SESS6:CONN:PORT2:SEL \"\"APC 3.5 female\"\"\" \n'SCPI.Execute \"SENS:CORR:COLL:SESS6:CKIT:PORT1:SEL \"\"85052D\"\"\" \n'SCPI.Execute \"SENS:CORR:COLL:SESS6:CKIT:PORT2:SEL \"\"85052D\"\"\" \n'Choose the between ECal or Mechanical calibration for the \n'Mixer Characterization portion of the VMC cal. \nSCPI.Execute \"SENS:CORR:COLL:SESS6:VMC:MIX:CHAR:CAL:OPT \"\"ECAL\"\"\" \n'This command sets the port mapping for the ECal to be used \n'during the Mixer Characterization portion of the VMC cal. \n'It is a required command if in the previous command the option \n'was set to 'ECAL'. The only valid port maps are either 'A1' \n'or 'B1'. \nSCPI.Execute \"SENS:CORR:COLL:SESS6:VMC:MIX:ECAL:PORT 1, \"\"A1\"\"\" \n'Specify the ECal module and the ECal characterization for the \n'two port calibration portion of this session. FCA calibrations \n'currently only support ECal module number 1. In this example \n'the factory characterization is used by specifying 0 for the \n'characterization number. \nSCPI.Execute \"SENS:CORR:COLL:SESS6:VMC:TWOP:ECAL:CHAR 1,0\" \n'Specify the ECal module and the ECal characterization for the \n'Mixer Characterization portion of this session. FCA calibrations \n'currently only support ECal module number 1. In this example \n'the factory characterization is used by specifying 0 for the \n'characterization number. \nSCPI.Execute \"SENS:CORR:COLL:SESS6:VMC:MIX:ECAL:CHAR 1,0\" \n'Specify the thru measurement method. This applies to both ECal \n'and mechanical calibrations. For ECal 'DEFAULT' will use the ECal \n'thru. Other choices may be used depending on the genders and types \n'of the connectors on the test interface. \nSCPI.Execute \"SENS:CORR:COLL:SESS6:VMC:TWOP:METH \"\"DEFAULT\"\"\" \n'Omit the isolation part of the 2-port cal \nSCPI.Execute \"SENS:CORR:COLL:SESS6:VMC:TWOP:OMIT 1\" \n'Turn on auto orientation for the ECal \nSCPI.Execute \"SENS:CORR:COLL:SESS6:VMC:TWOP:ECAL:ORI:STATE 1\" \n'Tell the wizard to generate and report the number of steps in this \n'cal session \nDim steps \nDim desc \n'Determine the number of steps required to complete the calibration. \n'First send the write command, then the query. \nSCPI.Execute \"SENS:CORR:COLL:SESS6:STEP\" \nsteps = SCPI.Execute (\"SENS:CORR:COLL:SESS6:STEP?\") \nFor i = 1 To steps \n1987\n\n'Display the prompt for each step \ndesc = SCPI.Execute (\"SENS:CORR:COLL:SESS6:DESC? \" & CStr(i)) \nMsgBox (desc) \n'Perform the measurement for each step \nSCPI.Execute \"SENS:CORR:COLL:SESS6:ACQ \" & CStr(i) \nNext \nDim calset \n'Finish the cal and save the calset \ncalset = SCPI.Execute (\"SENS:CORR:COLL:SESS6:SAVE?\") \nMsgbox (\"VMC Cal Complete!\") \n1988\n\nCreate and Cal an SMC Measurement \nThis Visual Basic example creates and calibrates a scalar mixer measurement. \nTo run this example without modification you need the following: \nA Mixer setup file saved on the PNA: C:\\Program Files\\Agilent\\Network \nAnalyzer\\Documents\\Mixer\\MyMixer.mxr. \nIf the mixer file uses an external LO source, it must also be attached and configured. \nAn ECAL module that covers the frequency range of the measurement. \nA power meter must be attached to the PNA. If this example is run in the PNA, the power meter does not \nneed to be attached using a GPIB/USB interface. \nThe SCPI commands in this example are sent over a COM interface using the SCPIStringParser object. You do \nNOT need a GPIB connection to run this example. However, some modification is necessary to make the program \nrun on a traditional GPIB Interface. For example, during the power meter portion of this calibration, scpi.Execute \nwill not process a command until the power meter routine has completed. Traditional GPIB would require a serial \npolling technique to ensure the routine has completed before proceeding. \nThis VBScript (*.vbs) program can be run as a macro in the PNA. To do this, copy the following code into a text \neditor file such as Notepad and save it on the PNA hard drive as SMC.vbs. Learn how to setup and run the macro. \nDim app \nDim scpi \n' Create / Get the PNA application. \nSet app = CreateObject(\"AgilentPNA835x.Application\") \nSet scpi = app.ScpiStringParser \n'---Create a Scalar Mixer Forward Measurement \n'First, delete all measurements on the channel \nscpi.Execute \"CALC:PAR:DEL:ALL\" \n'Create a forward scalar mixer measurement and configure it in \n'channel 1. The first parameter is a unique \n'identifying string (specified by the user) to allow subsequent \n'commands to be directed at this specific measurement. \nscpi.Execute \"CALC:CUST:DEF 'My SC21', 'Scalar Mixer/Converter', 'SC21'\" \n'Setup the new measurement as the 2nd trace in the active window \nscpi.Execute \"DISP:WIND:TRAC2:FEED 'My SC21'\" \n'Make the new trace the active measurement \nscpi.Execute \"CALC:PAR:SEL 'My SC21'\" \n'The parameters of the mixer measurement can now be configured. \n'This can be done by either using the individual SENS:MIX commands \n'for each of the parameters or by loading a mixer setup file. This \n'example loads a mixer setup file. The path name \n'for the mixer file may be loaded from other mapped drives \nscpi.Execute \"SENS:MIXer:Load \"\"C:\\Program Files\\Agilent\\Network \nAnalyzer\\Documents\\Mixer\\MyMixer.mxr\"\"\" \n'--------------Perform A Scalar Mixer Calibration---------------------- \n'Initialize an SMC guided calibration for session number 6 \n1989\n\nscpi.Execute \"SENS:CORR:COLL:SESS6:INIT \"\"SMC\"\"\" \n'Select to use an ECal for the 2-port cal portion of the procedure \n'To use a mechanical kit you will have to use the following command: \n'scpi.Execute \"SENS:CORR:COLL:SESS6:SMC:TWOPort:OPTion \"\"MECH\"\"\" \nscpi.Execute \"SENS:CORR:COLL:SESS6:SMC:TWOPort:OPTion \"\"ECAL\"\"\" \n'If you select the mechanical method then you also have to \n'specify the connector types and the cal kits for each of the ports. \n'The comments below show an example of how that is done: \n'scpi.Execute \"SENS:CORR:COLL:SESS6:CONN:PORT1:SEL \"\"APC 3.5 male\"\"\" \n'scpi.Execute \"SENS:CORR:COLL:SESS6:CONN:PORT2:SEL \"\"APC 3.5 female\"\"\" \n'scpi.Execute \"SENS:CORR:COLL:SESS6:CKIT:PORT1:SEL \"\"85052D\"\"\" \n'scpi.Execute \"SENS:CORR:COLL:SESS6:CKIT:PORT2:SEL \"\"85052D\"\"\" \n'Specify the ECal module and the ECal characterization for this \n'session. FCA calibrations currently only support ECal module \n'number 1. In this example the factory characterization is used \n'by specifying 0 for the characterization number. \nscpi.Execute \"SENS:CORR:COLL:SESS6:SMC:ECAL:CHAR 1,0\" \n'Specify the thru measurement method. This applies to both ECal \n'and mechanical calibrations. For ECal 'DEFAULT' will use the ECal \n'thru. Other choices may be used depending on the genders and types \n'of the connectors on the test interface. \nscpi.Execute \"SENS:CORR:COLL:SESS6:SMC:TWOP:METH \"\"DEFAULT\"\"\" \n'Omit the isolation part of the 2-port cal \nscpi.Execute \"SENS:CORR:COLL:SESS6:SMC:TWOP:OMIT 1\" \n'Turn on auto orientation for the ECal \nscpi.Execute \"SENS:CORR:COLL:SESS6:SMC:TWOP:ECAL:ORI:STATE 1\" \n'Tell the wizard to generate and report the number of steps in this \n'cal session \nDim steps \nDim desc \n'Determine the number of steps required to complete the calibration. \n'First send the write command, then the query. \nscpi.Execute \"SENS:CORR:COLL:SESS6:STEP\" \nsteps = scpi.Execute (\"SENS:CORR:COLL:SESS6:STEP?\") \nFor i = 1 To steps \n'Display the prompt for each step \ndesc = scpi.Execute (\"SENS:CORR:COLL:SESS6:DESC? \" & CStr(i)) \nMsgBox (desc) \n'Perform the measurement for each step \nscpi.Execute \"SENS:CORR:COLL:SESS6:ACQ \" & CStr(i) \nNext \nDim calset \n'Finish the cal and save the calset \ncalset = scpi.Execute (\"SENS:CORR:COLL:SESS6:SAVE?\") \nMsgbox (\"SMC Cal Complete!\") \n1990\n\nCreate an SMC Fixed Output Measurement \nThis VB Script example creates a calibrated SMC fixed output measurement using a controlled LO. Then a single \nsweep is taken and data is retrieved. \nThis example requires that an external LO be previously setup and named '8360'. \nFixed output measurements require that an external LO source be swept and synchronized with the PNA source. \nFCA performs this synchronization using the external source configuration settings. \nThe fastest, and recommended, method of controlling the LO source is Hardware List (BNC) triggering mode. \nHowever, in this mode, FCA channels will not respond to manual triggers. Therefore, the example uses the \nfollowing mechanism to trigger a sweep: \nWrite \"SENS:SWE:MODE HOLD\" 'place channel 1 in HOLD mode \nWrite \"INIT:CONT ON\" 'place PNA in internal trigger mode \nWrite \"SENS:SWE:GRO:COUNT 1\" 'specify that the group count is 1 sweep \nWrite \"SENS:SWE:MODE GROUPS\" 'execute group count (1 sweep) \nWrite \"*OPC?\" 'wait until the sweep is complete \nRead \nThe SCPI commands in this example are sent over a COM interface using the SCPIStringParser object. You can \nrun a VBScript (*.vbs) program from the PNA using Macros. To run this program, copy the following code into a text \neditor and save it as a *.vbs file. \noption explicit \n' Setup infrastructure to use the SCPI over COM \ndim app \nset app = createobject(\"Agilentpna835x.application\") \ndim p \nset p = app.scpistringparser \ndim returnStr \nsub Write (command) \nif len(returnStr) <> 0 then \nerr.Raise 55,\"Write\",\"Query Unterminated\" \nend if \nreturnStr = p.parse(command) \nend sub \nsub WriteIgnoreError(command) \nreturnStr = p.Execute(command) \np.Parse(\"SYST:ERR?\") ' clear error queue \nend sub \nfunction Read \nif len(returnStr) = 0 then \nerr.Raise 55,\"Read\",\"Bad read\" \n1991\n\nend if \nRead = returnStr \nreturnStr = \"\" \nend function \nWrite \"SYST:PRES\" \n' When programming in remote mode, hold mode is recommended \nWrite \"SENS:SWE:MODE HOLD\" \n' Delete the standard measurement \nWrite \"CALC:PAR:DEL:ALL\" \n' Create an SC21 measurement \nWrite \"CALC:CUST:DEF 'MySMC', 'Scalar Mixer/Converter', 'SC21'\" \nWrite \"DISP:WIND:TRACE:FEED 'MySMC'\" \nWrite \"CALC:PAR:SEL 'MySMC'\" \n' Set number of points to 11 \nWrite \"SENS:SWE:POIN 11 \" \n' Setup the mixer parameters for a swept LO, fixed output measurement \nWrite \"SENS:MIX:INP:FREQ:START 200e6\" \nWrite \"SENS:MIX:INP:FREQ:STOP 700e6\" \nWrite \"SENS:MIX:LO:FREQ:MODE Swept\" \nWrite \"SENS:MIX:OUTPUT:FREQ:FIX 3.4e9\" \nWrite \"SENS:MIX:OUTP:FREQ:SID HIGH\" \nWrite \"SENS:MIX:INP:POW -17\" \nWrite \"SENS:MIX:LO:POW 10\" \n' Specify the LO name, for controlled LO. \n' This name is setup in the External Source Config Dialog \n'Write \"SENS:MIX:LO:NAME '8360'\" \n' The CALC method calculates the LO frequency from the other parameters, \n' It also applies the mixer parameters to the channel. \nWrite \"SENS:MIX:CALC LO_1\" \n' Create an S11 in the same channel \nWrite \"CALC:CUST:DEF 'MyS11', 'Scalar Mixer/Converter', 'S11'\" \nWrite \"DISP:WIND:TRACE2:FEED 'MyS11'\" \nWrite \"CALC:PAR:SEL 'MyS11'\" \n' Create an IPwr in the same channel \nWrite \"CALC:CUST:DEF 'MyIPwr', 'Scalar Mixer/Converter', 'IPwr'\" \nWrite \"DISP:WIND:TRACE3:FEED 'MyIPwr'\" \n1992\n\nWrite \"CALC:PAR:SEL 'MyIPwr'\" \n' Create an OPwr in the same channel \nWrite \"CALC:CUST:DEF 'MyOPwr', 'Scalar Mixer/Converter', 'OPwr'\" \nWrite \"CALC:PAR:SEL 'MyOPwr'\" \nWrite \"DISP:WIND:TRACE4:FEED 'MyOPwr'\" \n' Perform a single sweep, synchronously. When *OPC returns, the sweep is done \nWrite \"SENS:SWE:GRO:COUN 1\" \nWrite \"SENS:SWE:MODE GROUPS\" \nWrite \"*OPC?\" \nRead \n' Retrieve the SC21 data \nWrite \"CALC:PAR:SEL 'MySMC'\" \nWrite \"CALC:DATA? SDATA\" \ndim data \ndata = Read() \nwscript.echo(data) \n'Retrieve the S11 data \nWrite \"CALC:PAR:SEL 'MyS11'\" \nWrite \"CALC:DATA? SDATA\" \ndata = Read() \nwscript.echo(data) \n1993\n\nGetting and Putting Data using SCPI \nThis Visual Basic Program does the following: \nReads data from the analyzer \nPuts the data back into memory \nTo see the data on the analyzer after running the program, from the front panel click: \nTrace - Math/Memory - Memory Trace \nTo run this program, you need: \nAn established GPIB interface connection \nSee Other SCPI Example Programs \nNote: To change the read and write location of data, removing the comment from the beginning of ONE of the \nlines, and replace the comment in the beginning of the SDATA and SMEM lines. \nPrivate Sub ReadWrite_Click() \nDim i As Integer \nDim t As Integer \nDim q As Integer \nDim dat As String \nDim cmd As String \nDim datum() As Double \nGPIB.Configure \nGPIB.Write \"SYSTem:PRESet;*wai\" \n'Select the measurement \nGPIB.Write \"CALCulate:PARameter:SELect 'CH1_S11_1'\" \n'Read the number of data points \nGPIB.Write \"SENSe1:SWEep:POIN?\" \nnumpts = GPIB.Read \n'Turn continuous sweep off \nGPIB.Write \"INITiate:CONTinuous OFF\" \n'Take a sweep \nGPIB.Write \"INITiate:IMMediate;*wai\" \n'Ask for the Data \n'PICK ONE OF THESE LOCATIONS TO READ \n'GPIB.Write \"CALCulate:DATA? FDATA\" 'Formatted Meas \n'GPIB.Write \"CALCulate:DATA? FMEM\" 'Formatted Memory \nGPIB.Write \"CALCulate:DATA? SDATA\" 'Corrected, Complex Meas \n'GPIB.Write \"CALCulate:DATA? SMEM\" 'Corrected, Complex Memory \n'GPIB.Write \"CALCulate:DATA? SCORR1\" 'Error-Term Directivity \n'Number of values returned per data point \n1994\n\n'q = 1 ' Pick this if reading FDATA or FMEM \nq = 2 ' Otherwise pick this \n'Parse the data \nReDim datum(q, numpts) \nFor i = 0 To numpts - 1 \nFor t = 0 To q - 1 \n'Read the Data \ndat = GPIB.Read(20) \n'Parse it into an array \ndatum(t, i) = Val(dat) \nNext t \nNext i \n'PUT THE DATA BACK IN \nGPIB.Write \"format ascii\" \n'PICK ONE OF THESE LOCATIONS TO PUT THE DATA \n'cmd = \"CALCulate:DATA FDATA,\" 'Formatted Meas \n'cmd = \"CALCulate:DATA FMEM,\" 'Formatted Memory \n'cmd = \"CALCulate:DATA SDATA,\" 'Corrected, Complex Meas \ncmd = \"CALCulate:DATA SMEM,\" 'Corrected, Complex Memory \n'cmd = \"CALCulate:DATA SCORR1,\" 'Error-Term Directivity \nFor i = 0 To numpts - 1 \nFor t = 0 To q - 1 \nIf i = numpts - 1 And t = q - 1 Then \ncmd = cmd & Format(datum(t, i)) \nElse \ncmd = cmd & Format(datum(t, i)) & \",\" \nEnd If \nNext t \nNext i \nGPIB.Write cmd \nEnd Sub \n1995\n\nGetting and Putting Data \nThis Rocky Mountain Basic example does the following: \nTakes a sweep, and reads the formatted data trace into an array. The trace is read as a definite length \nblock. \n1. \nInstructs you to remove DUT 2. \nDownloads the trace back to the analyzer as an definite length block. 3.\nSee Other SCPI Example Programs \n100 DIM A$[10],Data1(1:51) \n110 INTEGER Digits,Bytes \n120 ! \n130 COM /Sys_state/ @Hp87xx,Scode \n140 ! Identify I/O Port \n150 CALL Iden_port \n160 ! \n170 ! \n180 OUTPUT @Hp87xx;\"SYST:PRES\" \n190 ! \n200 OUTPUT @Hp87xx;\"CALC:PAR:SEL 'CH1_S11_1'\" \n210 ! \n220 ! Set up the analyzer to measure 51 data points. \n230 OUTPUT @Hp87xx;\"SENS1:SWE:POIN 51;*OPC?\" \n240 ENTER @Hp87xx;Opc \n250 ! \n260 ! Take a single sweep, leaving the analyzer \n270 ! in trigger hold mode. \n280 OUTPUT @Hp87xx;\"ABOR;:INIT1:CONT OFF;:INIT1;*WAI\" \n290 ! \n300 ! Select binary block transfer \n310 OUTPUT @Hp87xx;\"FORM:DATA REAL,64\" \n320 ! \n330 ! Request the channel 1 formatted data array \n340 ! from the analyzer. \n350 OUTPUT @Hp87xx;\"CALC:DATA? FDATA\" \n360 ! \n370 ! Turn on ASCII formatting on the I/O path. \n380 ! It is needed for reading the header \n390 ! information. \n400 ASSIGN @Hp87xx;FORMAT ON \n410 ! \n420 ! Get the data header. \"A$\" will contain the \n430 ! \"#\" character indicating a block data transfer. \n440 ! \"Digits\" will contain the number of characters \n1996\n\n450 ! for the number of bytes value which follows. \n460 ENTER @Hp87xx USING \"%,A,D\";A$,Digits \n470 ! \n480 ! Get the rest of the header. The number of \n490 ! bytes to capture in the data array will be \n500 ! placed in \"Bytes\". Note the use of \"Digits\" \n510 ! in the IMAGE string. \n515 ! \n520 ENTER @Hp87xx USING \"%,\"&VAL$(Digits)&\"D\";Bytes \n525 PRINT \"HEADER\",A$,Digits,Bytes \n530 ! \n540 ! Turn off ASCII formatting on the I/O path; \n550 ! it is not needed for transferring binary \n560 ! formatted data. \n570 ASSIGN @Hp87xx;FORMAT OFF \n580 ! \n590 ! Get the data. \n600 ENTER @Hp87xx;Data1(*) \n610 ! \n620 ! Turn on ASCII formatting again. \n630 ASSIGN @Hp87xx;FORMAT ON \n640 ! \n650 ! Get the \"end of data\" character. \n660 ENTER @Hp87xx;A$ \n670 ! \n680 ! Display the first three numbers in the array. \n690 DISP \"Trace: \";Data1(1);Data1(2);Data1(3);\"...\" \n700 ! \n710 ! Use this time to visually compare the \n720 ! numbers to the visible data trace. \n730 WAIT 5 \n740 ! \n750 ! Prompt the operator to disconnect the test \n760 ! device and how to continue the program. \n770 DISP \"Disconnect the test device -- Press Continue\" \n780 PAUSE \n790 ! \n800 ! Update the display line. \n810 DISP \"Taking a new sweep...\"; \n820 ! \n830 ! Take a sweep so the display shows new data. \n840 OUTPUT @Hp87xx;\":INIT1;*WAI\" \n850 DISP \" Done.\" \n860 WAIT 5 \n870 ! \n880 ! Send the header for an indefinite block length \n890 ! data transfer. \n900 DISP \"Downloading saved trace...\"; \n915 ! The first byte '3' indicates the next three digits equal number of transfer \nbytes \n916 ! The number of transfer bytes equals 8x the number of tracepoints. \n920 OUTPUT @Hp87xx;\"CALC:DATA FDATA, #3408\"; \n1997\n\n930 ! \n940 ! Turn off ASCII formatting. \n950 ASSIGN @Hp87xx;FORMAT OFF \n960 ! \n970 ! Send the data array back to the analyzer. \n980 OUTPUT @Hp87xx;Data1(*),END \n990 ! \n1000 ! Turn on ASCII formatting again. \n1010 ASSIGN @Hp87xx;FORMAT ON \n1020 DISP \" Done!\" \n1030 END \n1040 ! \n1050 !************************************************************** \n1060 ! Iden_port: Identify io port to use \n1070 ! Description: This routines sets up the I/O port address for \n1080 ! the SCPI interface. For \"HP 87xx\" instruments, \n1090 ! the address assigned to @Hp87xx = 800 otherwise, \n1100 ! 716. \n1110 !************************************************************** \n1120 SUB Iden_port \n1130 COM /Sys_state/ @Hp87xx,Scode \n1140 ! \n1150 IF POS(SYSTEM$(\"SYSTEM ID\"),\"HP 87\")<>0 THEN \n1160 ASSIGN @Hp87xx TO 800 \n1170 Scode=8 \n1180 ELSE \n1190 ASSIGN @Hp87xx TO 716 \n1200 Scode=7 \n1210 END IF \n1220 ! \n1230 SUBEND !Iden_port \n1240 ! \n1998\n\nExternal Test Set Control using SCPI \nThis program demonstrates the use of several External Test Set Control commands. \nThe SCPI commands in this example are sent over a COM interface using the SCPIStringParser object. You do \nNOT need a GPIB connection to run this example. \nThis VBScript (*.vbs) program can be run as a macro in the PNA. To do this, copy the following code into a text \neditor file such as Notepad and save it on the PNA hard drive as ExtTS.vbs. Learn how to setup and run the \nmacro. \n' Demonstrate some SCPI commands for external testsets. \nDim pna \nSet pna = CreateObject(\"AgilentPNA835x.Application\") \nSet scpi = pna.ScpiStringParser \n' The K64 testset is only usable on a 4-port PNA \nIf (pna.NumberOfPorts <> 4) Then \nMsgBox(\"This program only runs on 4-port analyzers.\") \nElse \n'If Help is active, show the measurement window and help \nscpi.Execute(\"DISP:ARR TILE\") \n'Return the list of supported test sets \nlist=scpi.Execute(\"SENS:MULT:CATalog?\") \nMsgBox(list) \n'************* K64 ***************** \n'The K64 is connected using the Testset I/O \n'connector. There is no handshake information. \n'Therefore, a testset need not be connected. \n' Load a configuration file. \nscpi.Execute(\"SENS:MULT1:TYPE 'Z5623AK64'\") \nscpi.Execute(\"SENS:MULT1:ADDR 0\") \n'return stuff about the test set \n' Returns number of input ports \nInports=scpi.Execute(\"SENS:MULT1:INCount?\") \nMsgBox(\"Input Ports: \" & CStr(Inports)) \n' Returns number of output ports \nports=scpi.Execute(\"SENS:MULT1:COUNt?\") \nMsgBox(\"Output Ports: \" & CStr(ports)) \n' Returns valid output ports for each input port \n1999\n\nFor portNum = 1 To Inports \nports=scpi.Execute(\"SENS:MULT1:PORT\" & CStr(portNum) & \":CAT?\") \nMsgBox(\"Port \" & CStr(portNum) & \" catalog: \" & (ports)) \nNext \n'Set different port mapping \nscpi.Execute(\"SENS:MULT1:ALLPorts '1 ext R,2 ext R,3 ext R,4 ext R'\") \n'Return port mapping \nportMap=scpi.Execute(\"SENS:MULT1:ALLPorts?\") \nMsgBox(\"Ports will be mapped to \" & CStr(portMap)) \n' Enable external testset control and execute port mapping. This automatically \nenables status bar display as well. \nscpi.Execute(\"SENS:MULT1:STATe 1\") \nMsgBox(\"Z5623A K64 Enabled\") \nEnd If \n2000\n\nTransfer Data using GPIB \nThe following RMB examples transfer data to and from a remote PC using the MMEM:TRANsfer command. \nTransferring data FROM the PNA -- TO a remote PC: \n30 ! \n40 ! Set up I/O paths \n50 ! \n60 ! Network analyzer address \n70 ASSIGN @Na TO 716 \n75 ! \n77 ! File to be stored on local computer \n80 ! First time -- need to create the file. \n90 ! After file name, number records set to 0 (ignored by WinOS) \n95 ! Use \"PURGE\" command to delete if desired. \n100 CREATE \"mytestdata.s2p\",0 \n110 ASSIGN @File TO \"mytestdata.s2p\" \n120 ! \n122 ! TRANSFER the data (download) \n123 ! \n125 ! Analyzer has file 'testdata.s2p' in default directory \n130 OUTPUT @Na;\":MMEM:TRAN? \"\"testdata.s2p\"\"\" \n135 ! \n137 ! Now unravel the bytes coming back from the analyzer. \n140 ENTER @Na USING \"#,A\";A$ \n150 ENTER @Na USING \"#,A\";Digit$ \n160 ! \n170 ! Create appropriate \"image\" \n180 Img$=\"#,\"&Digit$&\"A\" \n190 ! \n200 ! Byte$ holds the number of bytes in string format \n210 ENTER @Na USING Img$;Byte$ \n220 ! \n230 ! Allocate a buffer for holding the data \n240 ALLOCATE Dat$[VAL(Byte$)] \n250 ! \n260 ! Set up a different image for filling the buffer \n270 Img$=Byte$&\"A\" \n280 ! \n290 ! Retrieve the actual file data \n300 ENTER @Na USING Img$;Dat$ \n305 ! \n307 ! Now save the file locally. \n310 OUTPUT @File;Dat$ \n320 END \nTransferring data FROM the remote PC - TO the PNA: \n40 ! Set up I/O paths \n2001\n\n50 ! \n60 ! Network analyzer address \n70 ASSIGN @Na TO 716 \n77 ! File to be retrieved from local computer \n78 ASSIGN @File TO \"mytestdata.s2p\" \n79 ! \n120 ! \n122 ! TRANSFER the data \n123 ! \n230 ! Allocate a buffer for holding the data \n240 ALLOCATE Dat$[26236] \n250 ! \n260 ! Get data from the file and fill Dat$ \n270 ENTER @File;Dat$ \n280 ! \n325 ! Data to be transferred to analyzer file 'testupld.s2p' \n325 ! in default directory. \n326 ! \n327 ! A specific block transfer designator must follow the \n328 ! file name: \n329 ! '#' specifies a block transfer. \n330 ! '6' specifies 6 digits to follow. \n331 ! '026236' matches the buffer size allocated above \n332 ! not counting <NL><END> (new line and end of file). \n430 OUTPUT @Na;\":MMEM:TRAN \"\"testupld.s2p\"\",#6026236\",Dat$ \n520 END \n2002\n\nEstablish a VISA Session \nThis Visual Basic program demonstrates how to send a SCPI command using VISA and the Agilent IO libraries. To \nrun this program, you need: \nYour PC and PNA both connected to a LAN (for communicating with each other). \nThe SICL and VISA components of Agilent�s I/O Libraries software installed on your PC. Both are included \nwhen you install the software, unless you already have another vendor's VISA installed. Then specify Full \nSICL and VISA installation to overwrite the other vendor's VISA. \nThe module visa32.bas added to your VB project. After you install VISA, the module will be located at \nC:\\VXIPNP\\WINNT (or equivalent)\\INCLUDE\\Visa32.bas \nA form with two buttons: cmdRun and cmdQuit. \nYour PC configured to be a VISA LAN Client, and the SICL Server capability enabled on the PNA. See \nConfigure for VISA and SICL \nSee Other SCPI Example Programs \nNote: This example is a piece of a larger VISA program that performs a source power calibration. \n'Session to VISA Default Resource Manager \nPrivate defRM As Long \n'Session to PNA \nPrivate viPNA As Long \n'VISA function status return code \nPrivate status As Long \nPrivate Sub Form_Load() \ndefRM = 0 \nEnd Sub \nPrivate Sub cmdRun_Click() \n' String to receive data from the PNA. \n' Dimensioned large enough to receive scalar comma-delimited values \n' for 21 frequency points (20 ASCII characters per point) \nDim strReply As String * 420 \n' Open the VISA default resource manager \nstatus = viOpenDefaultRM(defRM) \nIf (status < VI_SUCCESS) Then HandleVISAError \n' Open a VISA session (viPNA) to the SICL LAN server \n' at �address 16� on the PNA pointed to by the �GPIB0� \n' VISA LAN Client on this PC. \n' CHANGE GPIB0 TO WHATEVER YOU PNA IS SET TO \nstatus = viOpen(defRM, \"GPIB0::16::INSTR\", 0, 0, viPNA) \nIf (status < VI_SUCCESS) Then HandleVISAError \n' Need to set the VISA timeout value to give all our calls to \n2003\n\n' myGPIBRead sufficient time to complete before a timeout \n' error occurs. \n' For this example, let's try setting the limit to \n' 30000 milliseconds (30 seconds). \nstatus = viSetAttribute(viPNA, VI_ATTR_TMO_VALUE, 30000) \nIf (status < VI_SUCCESS) Then HandleVISAError \n' Preset the PNA \nstatus = myGPIBWrite(viPNA, \"SYST:PRES\") \nIf (status < VI_SUCCESS) Then HandleVISAError \n' Print the data using a message box \nMsgBox strReply \nEnd Sub \nPrivate Sub cmdQuit_Click() \n' Close the resource manager session (which also closes \n' the session to the PNA). \nIf defRM <> 0 Then Call viClose(defRM) \n' End the program \nEnd \nEnd Sub \nPrivate Function myGPIBWrite(ByVal viHandle As Long, ByVal strOut As String) As Long \n' The \"+ Chr$(10)\" appends an ASCII linefeed character to the \n' output, for terminating the write transaction. \nmyGPIBWrite = viVPrintf(viHandle, strOut + Chr$(10), 0) \nEnd Function \nPrivate Function myGPIBRead(ByVal viHandle As Long, strIn As String) As Long \nmyGPIBRead = viVScanf(viHandle, \"%t\", strIn) \nEnd Function \nSub HandleVISAError() \nDim strVisaErr As String * 200 \nCall viStatusDesc(defRM, status, strVisaErr) \nMsgBox \"*** Error : \" + strVisaErr, vbExclamation \nEnd \nEnd Sub \n2004\n\nSee Other SCPI Example Programs \nStatus Reporting using SCPI \nThis Visual Basic program demonstrates two methods of reading the analyzer's status registers: \nPolled Bit Method - reads the Limit1 register continuously. \nSRQ Method - enables an interrupt of the program when bit 6 of the status byte is set to 1. The program then \nqueries registers to determine if the limit line failed. \nTo run this program, you need: \nAn established GPIB interface connection \nA form with two buttons: Poll and SRQ Method \nA means of causing the limit line to fail, assuming it passes initially. \nPrivate Sub Poll_Click() \n' POLL THE BIT METHOD \n' Clear status registers \nGPIB.Write \"*CLS\" \n'Loop FOREVER \nDo \nDoEvents \nGPIB.Write \"STATus:QUEStionable:LIMit1:EVENt?\" \nonn = GPIB.Read \nLoop Until onn = 2 \nMsgBox \"Limit 1 Failed \" \nEnd Sub \nPrivate Sub SRQMethod_Click() \n'SRQ METHOD \nGPIB.Write \"SYSTem:PRESet\" \nGPIB.Write \"CALCulate:PARameter:SELect 'CH1_S11_1'\" \n'slow down the trace \nGPIB.Write \"SENS:BWID 150\" \n'Setup limit line \nGPIB.Write \"CALC:LIM:DATA 2,3e9,6e9,-2,-2\" \nGPIB.Write \"CALC:LIMit:DISP ON\" \nGPIB.Write \"CALC:LIMit:STATe ON\" \n' Clear status registers. \nGPIB.Write \"*CLS;*wai\" \n' Clear the Service Request Enable register. \nGPIB.Write \"*SRE 0\" \n' Clear the Standard Event Status Enable register. \nGPIB.Write \"*ESE 0\" \n2005\n\n' Enable questionable register, bit(10) to report to the status byte. \nGPIB.Write \"STATus:QUEStionable:ENABle 1024\" \n' Enable the status byte register bit3 (weight 8) to notify controller \nGPIB.Write \"*SRE 8\" \n' Enable the onGPIBNotify event \nGPIB.NotifyMask = cwGPIBRQS \nGPIB.Notify \nEnd Sub \n---------------------------------------------------- \nPrivate Sub GPIB_OnGPIBNotify(ByVal mask As Integer) \n' check to see what failed \n' was it the analyzer? \nGPIB.Write \"*STB?\" \nonn = GPIB.Read \nIf onn <> 0 Then \n' If yes, then was it the questionable register? \nGPIB.Write \"STATus:QUEStionable:EVENt?\" \nonn = GPIB.Read \n' Determine if the limit1 register, bit 8 is set. \nIf onn = 1024 Then \n'if yes, then was it trace 1? \nGPIB.Write \"STAT:QUES:LIMIT1:EVEN?\" \nonn = GPIB.Read \nIf onn = 2 Then MsgBox (\"Limit Line1 Failed\") \nEnd If \nEnd If \nEnd Sub \n2006\n\nCreate a Custom Power Meter Driver \nThis topic requires that you have a working knowledge of Visual Basic. \nThis topic will help you create your own power meter driver for use with Source Power Calibration on the PNA. If \nyou are using an Agilent Power Meter to perform a Source Power Calibration, you do NOT need to create your own \ndriver. \nYour Power Meter driver will be created from a template written in Visual Basic using VISA over the GPIB bus. \nNote: This procedure applies to Visual Basic 6.0. Applicability to Visual Basic .NET has not yet been investigated. \nPrepare Template Files \nModify Template Files \nCompile, Copy, and Register, Your New Driver \nTest Your new Driver \nOther SCPI Example Programs \nPrepare Template Files \nCopy all the files from the PNA hard drive C:\\Program Files\\Agilent\\Network Analyzer\\Automation\\Power Meter \nDriver Template folder, to a folder on your development PC. \n1. \nIn Visual Basic click File, then Open Project�, find MyPowerMeter.vbp (a file you copied from the PNA). Click \nOpen. This is a VB ActiveX EXE template, which you will fill in to become your driver. \n2. \nClick Project, then MyPowerMeter Properties. Click the General tab. 3. \nOverwrite the Project Name with a name of your own choosing. This will be the name of your driver�s type library \n(also the default name of your exe). \n4.\nNote If the name of your exe does not match the VB Project Name with which it was compiled, registration of the \nexe on the PNA will not succeed. \nSet the Project Description. After building your driver if you wish to test it using VB, this is the string that will \nshow up in the VB References list of your test project, and also in the lower pane of the VB Object Browser. \n5. \nSet the Thread Pool size to 1 thread. 6. \nClick OK to close the project properties dialog. 7. \nFrom the VB Project menu, click References� Ensure that Agilent PNA Power Meter 1.0 Type Library and \nVISA Library are checked. Click OK. \n8.\nNote: Agilent's implementation of VISA is installed as part of the Agilent I/O Libraries on the PNA. For help on \n2007\n\nVISA, go to the Windows Start button on your PNA, select Programs, Agilent IO Libraries, VISA Help. \nModify Template Files \nFrom Visual Basic View menu click Project Explorer. Expand the Modules and Class Modules folders. Ensure \nthere is one module (WinAPI) and one class module (PowerMeter). \nLet's look at the WinAPI module first. \nIn the Project Explorer window, click WinAPI. 1. \nFrom the View menu click Code. 2.\nThere is only one line of code you should need to modify in this module: the value of the string constant named \nsIDSEARCH. The comments preceding the declaration of that string describe how to change it. The rest of this \nmodule contains functions which will use the Microsoft Windows API to insure proper registration of your driver on \nthe PNA. If you know of other Windows API functions you feel might be helpful to call from within your PowerMeter \nclass module (to help in formatting data, for example), this module would be the place to declare them. \nNow let's look at the class module. \nIn the Project Explorer window, click PowerMeter. 1. \nFrom the View menu click Properties Window. The Instancing property must be set to MultiUse. This allows \nother applications to create objects from this class, such that one instance of your driver EXE can supply more \nthan one such object at a time. \n2. \nFrom the View menu click Code. 3.\nDo NOT modify the Interfaces to IPowerMeter subroutines and functions. PNA source power cal expects to find \nthese interfaces as they are currently defined. \nThe only members that you need to supply code to are those containing �Your code here� comments. \nIn addition, comments have been provided at the beginning of each member to describe the information that \nmember needs to be read from or written to the power meter. \nTo get an idea of how communicate with the power meter using the VISA functions viWrite and viRead, examine \nthe code which has been implemented for you in IPowerMeter_Connect, IPowerMeter_QueryMeter, and \nIPowerMeter_WriteMeter. \nCompile, Copy, and Register Your New Driver \nWhen your driver is ready to run, you will first need to compile it into an EXE. \nFrom the File menu select Make exe. \nAfter compiling, the following will instruct VB to use the same ID (GUID) every time you re-compile your project. \nFrom the Project menu, click PowerMeter Properties. 1. \nOn the Component tab, select Binary Compatibility and click ... 2. \nBrowse to and select your project EXE. Click Open. 3. \n4. \n5. \n2008\n\n2. \n3. \nClick OK to close Project Properties. 4. \nSave your project. 5. \nCopy your driver EXE file to a folder on your PNA (do NOT use C:\\Program Files\\Agilent\\Network \nAnalyzer\\Automation\\Power Meter Driver Template folder). \n6. \nRun the EXE file. A message box will pop up reporting whether or not registration was successful. If not \nsuccessful, it will make a suggestion on what to fix. \n7.\nWhen your driver is properly registered, PNA Source Power Cal should be able to associate it with the ID string of \nyour power meter. \nTest Your Power Meter Driver \nWe have also provided a Visual Basic project to test your new Power Meter driver. This project individually calls \nevery IPowerMeter method and property in your driver to verify that it performs correctly. Before running the test \nyour PC and PNA must be configured to communicate using DCOM. \nConnect your PC and the PNA to LAN. 1. \nAdd your PC logon to the PNA. Both logons and password must match to communicate using DCOM. See \nAdditional PNA users. \n2. \nConfigure your driver using DCOM Config on the PNA. This will give you permission to launch and access the \ndriver. See Configure for COM-DCOM Programming. \n3.\nModify the Test Project \nIn Visual Basic click File, then Open Project�, find MyPowerMeterTest.vbp (a file you copied from the PNA). \nClick Open. \n1. \nFrom the Project menu, click References� From the list, find and check your new Power Meter Driver. (It \nshould have been registered on your PC when you successfully made your driver EXE.) Click OK. \n2. \nFrom the View menu click Code. 3. \nModify the CreateObject line as follows: \nReplace MyPowerMeter with the Project Name that you chose for your driver \nReplace MyPNA with the Computer Name of your PNA. \nFor example: \n4.\nSet PowerMeterObj = CreateObject(\"AcmeBrand.PowerMeter\", \"AGILENT-PNA123\") \n(This assumes that you kept PowerMeter as class module name in your driver.) \nRun the Test Project \nEnsure your power meter is connected to the PNA with a GPIB cable. \nPut the PNA in system controller mode: \n1. \n2. \n2009\n\nFrom the PNA System menu point to Configure then click SICL/GPIB. 1. \nIn the GPIB box click System Controller. 2.\nRun the test project. If there are no errors, the driver is created successfully. If there are errors, try to figure out \nwhat went wrong and fix it. Then re-compile, re-copy the .exe to the PNA, and re-run the test. You should not need \nto re-register the driver or re-modify the test program. \n2010\n\nGPIB Pass-Through Example \nThe SCPI SYSTem commands used in this example allow you to send GPIB commands to another GPIB device \nthrough the PNA. The other GPIB device cannot be connected to the GPIB bus through the PNA rear panel if the \nPNA is being controlled by a remote PC using that connector. The other device would typically be connected to the \nPNA using a USB/GPIB interface. \nThis VB Script example uses the COM SCPIStringParser object. However, this is not critical to the use of these \ncommands; they can be sent using the normal syntax of your programming environment. Using the \nSCPIStringParser over LAN allows you to communicate with GPIB devices without requiring your remote PC to \nhave a GPIB interface card installed. \nAlthough this method of pass-through works for most applications, there are a couple of limitations: \nAll data is transferred using ASCII format. Therefore, transferring large blocks of data is very slow. \nOnly read and write functions are possible. Service Interrupts are not supported. \nSee Other SCPI Example Programs \noption explicit \ndim app \nset app = CreateObject(\"AgilentPNA835x.Application\") \ndim p \nset p = app.ScpiStringParser \n' Open a new GPIB session on Bus:2 Device:14 Timeout: 100ms \np.Parse \"SYST:COMM:GPIB:RDEV:OPEN 2,14,100\" \ndim handleAsStr \n' Retrieve the handle (ID number) \nhandleAsStr = p.Parse (\"SYST:COMM:GPIB:RDEV:OPEN?\") \n' Convert the handle to an integer \ndim handleAsInt \nhandleAsInt = CInt(handleAsStr) \n' Send the \"*IDN?\" query \np.Parse \"SYST:COMM:GPIB:RDEV:WRITE \" & handleAsInt & \",'*IDN?'\" \n' Read its results \ndim idn \nidn = p.Parse(\"SYST:COMM:GPIB:RDEV:READ? \" & handleAsInt) \nmsgbox idn \n' Close the GPIB session \np.Parse \"SYST:COMM:GPIB:RDEV:CLOSE \" & handleAsInt \n2011\n\nPNA as Controller and Talker / Listener \nThis Visual Basic Program uses VISA to do the following: \nControl the PNA using a VISA LAN Client interface on the PNA. \nControl another instrument using the PNA as GPIB controller. \nQueries both the analyzer and other instrument to identify themselves with *IDN? \nNote: This program can be modified to work from a remote PC to control both instruments. In that case, set up the \nPNA to be a talker/listener. \nTo run this program, you need to do the following: \nAdd module visa32.bas to the VB project. It is located on the analyzer at C:\\Program \nFiles\\HP\\VXIPNP\\WINNT\\Include\\VISA32.bas \nConfigure the PNA for VISA / SICL \nSet up the PNA to be GPIB system controller. \nOn the System menu, point to Configure. Click SICL / GPIB 1. \nClick System Controller 2. \nConnect another instrument to the analyzer through a GPIB cable with Primary address of 13 on GPIB0 \ninterface \nSee Other SCPI Example Programs \nSub main() \n'This application run from onboard the PNA \n'can control both the PNA and another GPIB instrument. \n'\n'To run this program the module visa32.bas must be added \n'to the project. \n'VISA function status return code \nDim status As Long \n'Session to Default Resource Manager \nDim defRM As Long \n'Session to instrument \nDim viPNA As Long \n'Session to other GPIB instrument \nDim viInstrument As Long \n'String to hold results \nDim strRes As String * 200 \nOn Error GoTo ErrorHandler \nstatus = viOpenDefaultRM(defRM) \n2012\n\nIf (status < VI_SUCCESS) Then GoTo VisaErrorHandler \n'Open the session to the PNA \nstatus = viOpen(defRM, \"GPIB1::16::INSTR\", 0, 0, viPNA) \nIf (status < VI_SUCCESS) Then GoTo VisaErrorHandler \n'Ask for the PNA's ID. \nstatus = viVPrintf(viPNA, \"*IDN?\" + Chr$(10), 0) \nIf (status < VI_SUCCESS) Then GoTo VisaErrorHandler \n'Read the ID as a string. \nstatus = viVScanf(viPNA, \"%t\", strRes) \nIf (status < VI_SUCCESS) Then GoTo VisaErrorHandler \n'Display the results \nMsgBox \"PNA is: \" + strRes \n'Open the session to the other instrument \nstatus = viOpen(defRM, \"GPIB0::13::INSTR\", 0, 0, viInstrument) \nIf (status < VI_SUCCESS) Then GoTo VisaErrorHandler \n'Ask for the instrument's ID. \nstatus = viVPrintf(viInstrument, \"*IDN?\" + Chr$(10), 0) \nIf (status < VI_SUCCESS) Then GoTo VisaErrorHandler \n'Read the ID as a string. \nstatus = viVScanf(viPNA, \"%t\", strRes) \nIf (status < VI_SUCCESS) Then GoTo VisaErrorHandler \n'Display the results \nMsgBox \"Other instrument is: \" + strRes \n' Close the resource manager session (which closes everything) \nCall viClose(defRM) \nEnd \nErrorHandler: \n'Display the error message \nMsgBox \"*** Error : \" + Error$, MB_ICONEXCLAMATION \nEnd \nVisaErrorHandler: \nDim strVisaErr As String * 200 \nCall viStatusDesc(defRM, status, strVisaErr) \nMsgBox \"*** Error : \" + strVisaErr \nEnd \nEnd Sub \n2013\n\nSocket Client \nThe following C# example demonstrates how to send a SCPI program to an Agilent TCP socket-enabled \ninstrument such as the PNA or ENA network analyzer. If the command is a query, the program will read the \ninstrument's response. You can add or replace the SCPI commands in this program with your own. \nLearn how to enable Sockets communication on the PNA. \nFor both of the following methods, first copy the example text below into a Notepad file and name it \nSocketClient.cs. \nTo run using Microsoft Visual Studio 2003 or 2005 \nFrom the Visual Studio File menu, select New, then Project. 1. \nIn the New Project window, select the following items (noting the location of the file folder it is creating for \nyou) then click OK. \n2. \nProject Type: Visual C# \nTemplate: Console Application \nProject Name: SocketClient \nCopy SocketClient.cs into the folder that was created in the previous step. 1. \nIn the Solution Explorer window pane, right-click Class1.cs (if Visual Studio 2003) or Program.cs (if Visual \nStudio 2005). Select Delete to delete that file. \n2. \nIn the Solution Explorer, right-click SocketClient , and select Add, then Existing Item�. 3. \nBrowse to select SocketClient.cs and click OK. 4. \nYou should then be able to build the project, and test the resulting SocketClient.exe from a command prompt \n(shell) window. \nTo run using Mono \nMono is a cross-platform version of .NET. You can download a free version of Mono at http:\\www.monoproject.\ncom. Once downloaded and installed: \nRun the Mono command prompt (shell) window. 1. \nNavigate to the directory where the example SocketClient.cs is stored. 2. \nType: MCS SocketClient.cs (builds the .exe and saves in that same folder.) 3. \nType mono SocketClient.exe <PNA name or IP address> 4. \nThis example was compiled and tested successfully with Mono version 1.1.13. It was run on a PC using the Red \n2014\n\n4. \nHat version 9.0 distribution of the Linux operating system. It was also run on a PC using Windows XP. This \nprogram has not been tested with other versions of Mono, or on other operating systems. \nTo run with Agilent T&M Toolkit \nAgilent T&M Toolkit 2.0 is the first version to support communication using Sockets. \nUse the following to address the Sockets port: TCPIP0::<PNA name or IP address>::5025::SOCKET \nusing System; \nusing System.Net; \nusing System.Net.Sockets; \n// This C# \"Console Application\" example program demonstrates sending \n// SCPI commands to an Agilent TCP socket-enabled instrument \n// (for example, a PNA or ENA network analyzer), and reading back the \n// instrument's response if the command is a query. \nnamespace CSharpSocketClient \n{\n/// <summary> \n/// The class supporting the main entry point for the application. \n/// </summary> \nclass MainClass \n{\n/// <summary> \n/// The main entry point for the application. \n/// </summary> \n[STAThread] \nstatic int Main(string[] args) \n{\ntry \n{\nif (args.Length != 1) \n{\nConsole.WriteLine(\"\"); \nConsole.WriteLine(\"Usage -- with Microsoft's .NET runtime:\"); \nConsole.WriteLine(\"SocketClient servernameoraddress\"); \nConsole.WriteLine(\"Example: SocketClient 192.168.0.1\"); \nConsole.WriteLine(\"\"); \nConsole.WriteLine(\"Usage -- with Mono's (www.mono-project.com) .NET runtime:\"); \n2015\n\nConsole.WriteLine(\"mono SocketClient.exe servernameoraddress\"); \nConsole.WriteLine(\"Example: mono SocketClient.exe 192.168.0.1\"); \nreturn 1; \n}\nstring server = args[0]; \nInt32 port = 5025; // default socket port number for the PNA \n// Create a TcpClient for the server instrument \n// and associated with the necessary port number. \nTcpClient client = new TcpClient(server, port); \n// Send a preset command to the instrument. \nParse(client, \"SYST:PRES\"); \n// Query the instrument ID. \nstring id = Parse(client, \"*IDN?\"); \n// Close the client session. \nclient.Close(); \n}\ncatch (ArgumentNullException e) \n{\nConsole.WriteLine(\"ArgumentNullException: {0}\", e); \n}\ncatch (SocketException e) \n{\nConsole.WriteLine(\"SocketException: {0}\", e); \n}\nConsole.WriteLine(\"\\n Press Enter to continue...\"); \nConsole.Read(); \nreturn 0; \n} \nstatic string Parse(TcpClient client, string command) \n{\n// Translate the passed command into ASCII and store it as a Byte array. \nByte[] data = System.Text.Encoding.ASCII.GetBytes(command); \n// Get a client stream for reading and writing. \nNetworkStream stream = client.GetStream();\n2016\n\n// Send the command to the socket-enabled instrument. \nstream.Write(data, 0, data.Length); \n// Has to be followed by a linefeed character as terminator. \nByte[] lf = {(Byte)'\\n'}; \nstream.Write(lf, 0, 1); \nConsole.WriteLine(\"Sent: {0}\", command); \n// If the message was a query (involved a question mark) \n// receive the instrument response. \nif (command.IndexOf(\"?\") >= 0) \n{\n// Buffer to store the response bytes. \n// For simplicity of this example, we allocate just for a 256-byte maximum \n// response size. \ndata = new Byte[256]; \n// String to store the response ASCII representation. \nstring responseData = String.Empty; \n// Read the batch of response bytes. \nInt32 bytes = stream.Read(data, 0, data.Length); \nresponseData = System.Text.Encoding.ASCII.GetString(data, 0, bytes); \nConsole.WriteLine(\"Received: {0}\", responseData); \nreturn responseData; \n}\nreturn \"\"; \n}}} \n2017\n\nGPIB Fundamentals \nThe General Purpose Interface Bus (GPIB) is a system of hardware and software that allows you to control test \nequipment to make measurements quickly and accurately. This topic contains the following information: \nThe GPIB Hardware Components \nThe GPIB / SCPI Programming Elements \nSpecifications \nGPIB Interface Capability Codes \nNote: All of the topics related to programming assume that you already know how to program, preferably using a \nlanguage that can control instruments. \nOther Topics about GPIB Concepts \nThe GPIB Hardware Components \nThe system bus and its associated interface operations are defined by the IEEE 488 standard. The following \nsections list and describe the main pieces of hardware in a GPIB system: \nGPIB Addresses \nEvery GPIB instrument must have its own unique address on the bus. The PNA address (716) consists of two \nparts: \nThe Interface select code (typically 7) indicates which GPIB port in the system controller is used to \ncommunicate with the device. \n1. \nThe primary address (16) is set at the factory. You can change the primary address of any device on the \nbus to any number between 0 and 30. To change the analyzer address click System \\ Configure \\ SICL-GPIB \n2. \nThe secondary address is sometimes used to allow access to individual modules in a modular instrument system, \nsuch as a VXI mainframe. The analyzer does not have secondary addresses. \nControllers \nControllers specify the instruments that will be the talker and listener in a data exchange. The controller of the bus \nmust have a GPIB interface card to communicate on the GPIB. \nThe Active Controller is the computer or instrument that is currently controlling data exchanges. \nThe System Controller is the only computer or instrument that can take control and give up control of the \nGPIB to another computer or instrument, which is then called the active controller. \nThe PNA can NOT be passed control of the GPIB. However, you can communicate with other GPIB devices \nthrough the PNA using one of, or a combination of, the following methods: \n2018\n\nUse the SCPI SYST:COMM:GPIB:RDEV: commands. \nUse VISA or SICL over LAN to accomplish this. See an example. \nUse USB / GPIB Interface \nUse a PNA with dedicated Controller and Talker/Listener GPIB ports. \nTalker / Listener Instruments \nThe PNA is configured as a Talker / Listener by default. \nTalkers are instruments that can be addressed to send data to the controller. \nListeners are instruments that can be addressed to receive a command, and then respond to the command. \nAll devices on the bus are required to listen. \nCables \nGPIB Cables are the physical link connecting all of the devices on the bus. There are eight data lines in a GPIB \ncable that send data from one device to another. There are also eight control lines that manage traffic on the data \nlines and control other interface operations. \nYou can connect instruments to the controller in any arrangement with the following limitations: \nDo not connect more than 15 devices on any GPIB system. This number can be extended with the use of a \nbus extension. \nDo not exceed a total of 20 meters of total cable length or 2 meters per device, whichever is less. \nAvoid stacking more than three connectors on the back panel of an instrument. This can cause unnecessary \nstrain on the rear-panel connector. \nThe GPIB / SCPI Programming Elements \nThe following software programming elements combine to become a GPIB program: \nGPIB / SCPI Commands \nProgramming Statements \nInstrument Drivers \nGPIB Commands \nThe GPIB command is the basic unit of communication in a GPIB system. The analyzer responds to three types of \nGPIB commands: \n1. IEEE 488.1 Bus-management Commands \nThese commands are used primarily to tell some or all of the devices on the bus to perform certain interface \noperations. \n2019\n\nAll of the functions that can be accomplished with these commands can also be done with IEEE 488.2 or SCPI \ncommands. Therefore, these commands are not documented in this Help system. For a complete list of IEEE 488.1 \ncommands refer to the IEEE 488 standard. Examples of IEEE 488.1 Commands \nCLEAR - Clears the bus of any pending operations \nLOCAL - Returns instruments to local operation \n2. IEEE 488.2 Common Commands \nThese commands are sent to instruments to perform interface operations. An IEEE 488.2 common command \nconsists of a single mnemonic and is preceded by an asterisk ( * ). Some of the commands have a query form \nwhich adds a \"?\" after the command. These commands ask the instrument for the current setting. See a complete \nlist of the Common Commands that are recognized by the analyzer. Examples of IEEE 488.2 Common Commands \n*OPC - Operation Complete \n*RST - Reset \n*OPT? - Queries the option configuration \n3. SCPI Commands \nThe Standard Commands for Programmable Instruments (SCPI) is a set of commands developed in 1990. The \nstandardization provided in SCPI commands helps ensure that programs written for a particular SCPI instrument \nare easily adapted to work with a similar SCPI instrument. SCPI commands tell instruments to do device specific \nfunctions. For example, SCPI commands could tell an instrument to make a measurement and output data to a \ncontroller. Examples of SCPI Commands: \nCALCULATE:AVERAGE:STATE ON \nSENSE:FREQUENCY:START? \nFor more information on SCPI: \nThe Rules and Syntax of SCPI Commands provides more detail of the SCPI command structure. \nSCPI Command Tree is a complete list of the SCPI commands for the analyzer \nProgramming Statements \nSCPI commands are included with the language specific I/O statements to form program statements. The \nprogramming language determines the syntax of the programming statements. SCPI programs can be written in a \nvariety of programming languages such as VEE, HP BASIC, or C++. Example of a Visual Basic statement: \nGPIB.Write \"SOURCE:FREQUENCY:FIXED 1000 MHz\" \nNote about examples \nInstrument Drivers \nInstrument drivers are subroutines that provide routine functionality and can be reused from program to program. \nGPIB industry leaders have written standards for use by programmers who develop drivers. When programmers \nwrite drivers that comply with the standards, the drivers can be used with predictable results. To comply with the \n2020\n\nstandard, each instrument driver must include documentation describing its functionality and how it should be \nimplemented. \nGPIB Specifications \nInterconnected devices - Up to 15 devices (maximum) on one contiguous bus. \nInterconnection path - Star or linear (or mixed) bus network, up to 20 meters total transmission path length or 2 \nmeters per device, whichever is less. \nMessage transfer scheme - Byte-serial, bit-parallel, asynchronous data transfer using an interlocking 3-wire \nhandshake. \nMaximum data rate - 1 megabyte per second over limited distances, 250 to 500 kilobytes per second typical \nmaximum over a full transmission path. The devices on the bus determine the actual data rate. \nAddress capability - Primary addresses, 31 Talk and 31 Listen; secondary addresses, 961 Talk and 961 Listen. \nThere can be a maximum of 1 Talker and up to 14 Listeners at a time on a single bus. See also previous section \non GPIB addresses. \nGPIB Interface Capability Codes \nThe IEEE 488.1 standard requires that all GPIB compatible instruments display their interface capabilities on the \nrear panel using codes. The codes on the analyzer, and their related descriptions, are listed below: \nSH1 full source handshake capability \nAH1 full acceptor handshake capability \nT6 basic talker, serial poll, no talk only, unaddress if MLA (My Listen Address) \nTEO no extended talker capability \nL4 basic listener, no listen only, unaddress if MTA (My Talk Address) \nLEO no extended listener capability \nSR1 full service request capability \nRL1 full remote / local capability \nPPO no parallel poll capability \nDC1 full device clear capability \nDT1 full device trigger capability \nC1 system controller capability \nC2 send IFC (Interface Clear) and take charge controller capability \nC3 send REN (Remote Enable) controller capability \n2021\n\nC4 respond to SRQ (Service Request) \n2022\n\nThe Rules and Syntax of SCPI \nMost of the commands used for controlling instruments on the GPIB are SCPI commands. The following sections \nwill help you learn to use SCPI commands in your programs. \nBranches on the Command Tree \nCommand and Query \nMultiple Commands \nCommand Abbreviation \nBracketed (Optional) Keywords \nVertical Bars (Pipes) \nMIN and MAX Parameters \nOther Topics about GPIB Concepts \nBranches on the Command Tree \nAll major functions on the analyzer are assigned keywords which are called ROOT commands. (See GPIB \nCommand Finder for a list of SCPI root commands). Under these root commands are branches that contain one or \nmore keywords. The branching continues until each analyzer function is assigned to a branch. A root command \nand the branches below it is sometimes known as a subsystem. \nFor example, the following graphic shows the SOURce subsystem. Under the SOURce and POWer keywords are \nseveral branch commands. \nSometimes the same keyword, such as STATE, is used in several branches of the command tree. To keep track of \nthe current branch, the analyzer's command parser uses the following rules: \nPower On and Reset - After power is cycled or after *RST, the current path is set to the root level \ncommands. \nMessage Terminators - A message terminator, such as a <NL> character, sets the current path to the root \ncommand level. Many programming language output statements send message terminators automatically. \nMessage terminators are described in Sending Messages to the Analyzer. \nColon (:) - When a colon is between two command keywords, it moves the current path down one level in \nthe command tree. For example, the colon in :SOURCE:POWER specifies that POWER is one level below \nSOURCE. When the colon is the first character of a command, it specifies that the following keyword is a root \nlevel command. For example, the colon in :SOURCE specifies that source is a root level command. \nNote: You can omit the leading colon if the command is the first of a new program line. For example, the following \ntwo commands are equivalent: \nSOUR:POW:ATT:AUTO \n:SOUR:POW:ATT:AUTO \n2023\n\n<WSP> - Whitespace characters, such as <tab> and <space>, are generally ignored. There are two \nimportant exceptions: \nWhitespace inside a keyword, such as :CALC ULATE, is not allowed. \nMost commands end with a parameter. You must use whitespace to separate these ending parameters \nfrom commands. Always refer to the command documentation. In the following example, there is \nwhitespace between STATE and ON. \nCALCULATE1:SMOOTHING:STATE ON \nComma (,) - If a command requires more than one parameter, you must separate adjacent parameters using \na comma. For example, the SYSTEM:TIME command requires three values to set the analyzer clock: one for \nhours, one for minutes, and one for seconds. A message to set the clock to 8:45 AM would be \nSYSTEM:TIME 8,45,0. Commas do not affect the current path. \nSemicolon(;) - A semicolon separates two commands in the same message without changing the current \npath. See Multiple Commands later in this topic. \nIEEE 488.2 Common Commands - Common commands, such as *RST, are not part of any subsystem. An \ninstrument interprets them in the same way, regardless of the current path setting. \nCommand and Query \nA SCPI command can be an Event command, Query command (a command that asks the analyzer for \ninformation), or both. The following are descriptions and examples of each form of command. GPIB Command \nFinder lists every SCPI command that is recognized by the analyzer, and its form. \nForm Examples \nEvent commands - cause an action to occur inside the \nanalyzer. \n:INITIATE:IMMEDIATE \nQuery commands - query only; there is no associated \nanalyzer state to set. \n:SYSTem:ERRor? \nCommand and query - set or query an analyzer setting. The \nquery form appends a question mark (?) to the set form \n:FORMat:DATA ! Command \n:FORMat:DATA? ! Query \nMultiple Commands \nYou can send multiple commands within a single program message. By separating the commands with semicolons \nthe current path does not change. The following examples show three methods to send two commands: \n1. \n2024\n\nTwo program messages: 1. \nSOURCE:POWER:START 0DBM \nSOURCE:POWER:STOP 10DBM \nOne long message. A colon follows the semicolon that separates the two commands causing the command \nparser to reset to the root of the command tree. As a result, the next command is only valid if it includes the \nentire keyword path from the root of the tree: \n2. \nSOURCE:POWER:START 0DBM;:SOURCE:POWER:STOP 10DBM \nOne short message. The command parser keeps track of the position in the command tree. Therefore, you \ncan simplify your program messages by including only the keyword at the same level in the command tree. \n3. \nSOURCE:POWER:START 0DBM;STOP 10DBM \nCommon Commands and SCPI Commands \nYou can send Common commands and SCPI commands together in the same message. (For more information on \nthese types of commands see GP-IB Fundamentals.) As in sending multiple SCPI commands, you must separate \nthem with a semicolon. \nExample of Common command and SCPI commands together \n*RST;SENSE:FREQUENCY:CENTER 5MHZ;SPAN 100KHZ \nCommand Abbreviation \nEach command has a long form and an abbreviated short form. The syntax used in this Help system use \nuppercase characters to identify the short form of a particular keyword. The remainder of the keyword is lower case \nto complete the long form. \nSOUR - Short form \nSOURce - Long form \nEither the complete short form or complete long form must be used for each keyword. However, the keywords used \nto make a complete SCPI command can be a combination of short form and long form. \nThe following is unacceptable - The first three keywords use neither short or long form. \nSOURc:Powe:Atten:Auto on \nThe following is acceptable - All keywords are either short form or long form. \nSOUR:POWer:ATT:AUTO on \nIn addition, the analyzer accepts lowercase and uppercase characters as equivalent as shown in the following \nequivalent commands: \nsource:POW:att:auto ON \nSource:Pow:Att:Auto on \nOptional [Bracketed] Keywords \n2025\n\nYou can omit some keywords without changing the effect of the command. These optional, or default, keywords are \nused in many subsystems and are identified by brackets in syntax diagrams. \nExample of Optional Keywords \nThe HCOPy subsystem contains the optional keyword IMMediate at its first branching point. Both of the following \ncommands are equivalent: \n\"HCOPY:IMMEDIATE\" \n\"HCOPY\" \nThe syntax in this Help system looks like this: \nHCOPy[:IMMediate] \nVertical Bars | Pipes \nVertical bars, or \"pipes\", can be read as \"or\". They are used in syntax diagrams to separate alternative parameter \noptions. \nExample of Vertical Bars:"
uses:
  PNA-X.lvlib
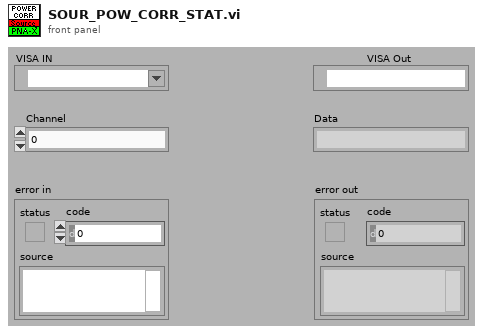
[diagram p1: front panel]
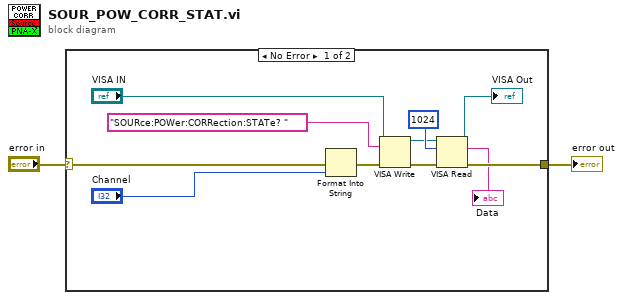
[diagram p0: block diagram]
diagram:
  n1 = case shown="No Error" "error in" {
    selector: "error in" -> [w13 w14]
    tunnel: [w7 w14] -> w1
    frame No Error {
      n2 = Format Into String(error in=w13, "Channel") -> (error out=w12:errorcluster)  [unwired: 2 in, 1 out]
      n3 = VISA Write(VISA resource name="VISA IN", write buffer="SOURce:POWer:CORRection:STATe? " ("Cmdline"), error in (no error)=w12) -> (VISA resource name out=w8:refnum<visa-resource-name>, error out=w10:errorcluster)  [unwired: 1 out]
      n4 = VISA Read(VISA resource name=w8, byte count=1024, error in (no error)=w10) -> (VISA resource name out=→"VISA Out":refnum<visa-resource-name>, read buffer=→"Data":string, error out=w7:errorcluster)  [unwired: 1 out]
    }
    frame Error {
    }
  }
  "error out" <- w1
